vi "MC_8_27_12b_JW.vi"() -> ()   [LabVIEW 2011]
uses:
  <vilib>/Utility/file.llb/Read From Spreadsheet File (string).vi
  <vilib>/Utility/inputDevices.llb/keyboardAcquire.vi
  <vilib>/Utility/file.llb/Write To Spreadsheet File (DBL).vi
  <vilib>/Utility/file.llb/Write To Spreadsheet File (string).vi
  <vilib>/regexp/Match Regular Expression.xnode
panel:
  out "Vd Header Row 2":sgl
  in  "default (0 dbl)":ext format="%.2e"
  out "Vd Header Row":sgl
  out "Transport Array":string[][](array[string])
  in  "Treatment Concentration (mM):":dbl=nan
  in  "Surface Treatment:":string="NaN"
  in  "# Drops*:":dbl=inf
  in  "Solution Temp (C):":dbl=nan
  in  "Relative Humidity (%):":dbl=nan
  in  "Room Temp (F):":dbl=nan
  in  "Time (s):":dbl=nan
  in  "RPM:":dbl=nan
  in  "Wait Time (s):":dbl=nan
  in  "Sample #:":dbl=1.0
  in  "Fabricator:":string="NaN"
  in  "Ramp (s):":dbl=3.0
  out "X Axis Display Type":string
  out "Opj X Axis":string
  in  "Room Temp":dbl=294.0
  out "No Image 2":path=path "\\\\acad1\\physics/Jurchescu-group/JW-PD/Image Not Found.png"
  out "Save1 Array":string[][](array[string])
  out "Lin Vd":dbl
  out "Lin-Vg Array-Used":dbl[](array[numeric])
  out "Lin Id-Used":dbl[](array[numeric])
  out "Rec: Comments":string
  out "Folder Index":dbl caption="Length"
  out "Current \nRecord":string[](array[string])
  out "Transformer \nHeaders":string[](array[string])
  out "Current Device ID":string
  out "Column":string
  out "Row":string
  out "Rec: Concentration":dbl
  out "Rec: Solvent":string
  out "Rec: Method":string
  in  "?":T1(tab)
  in  "Transport File":path
  out "Transport Folder":path
  out "Rec: Material":string
  out "Accel (RPM/s):":dbl
  in  "Transfer File":path
  out "Transfer Folder":path
  in  "Image Folder":path
  out "Image File":path=path "D:/UserData/Desktop/Jeremy/WFU/Research/Programs/VI mods/Image Not Found.png"
  in  "Manual Comments":bool
  in  "Comments:":string
  out "Calc: On/Off":dbl caption="On/Off-Sat" format="%#.2e"
  out "Calc: Off I-Sat":dbl caption="Off I-Sat" format="%#.2e"
  in  "Manuel-Dielectric":bool
  in  "Manuel-Length":bool
  out "Calc: VT-Lin":dbl
  out "New: VT-Lin":dbl
  out "Rec: VT-Lin":dbl caption="VT-Lin" format="%#_3g"
  out "Calc: Trap Density-STS":dbl format="%#.2e"
  out "New: Trap Density-STS":dbl format="%#.2e"
  out "Rec: Trap Density-STS":dbl caption="N-Sat (STS)" format="%#.2e"
  out "Calc: Trap Density-VT":dbl format="%#.2e"
  out "New: Trap Density-VT":dbl format="%#.2e"
  out "Rec: Trap Density-VT":dbl caption="N-Sat (VT)" format="%#.2e"
  out "Calc: Mobility-Lin":dbl format="%#.2e"
  out "New: Mobility-Lin":dbl format="%#_4e"
  out "Rec: Mobility-Lin":dbl caption="Mobility-Lin" format="%#_3e"
  out "Calc: Mobility-Sat":dbl format="%#.2e"
  out "Rec: Length":dbl caption="Length" format="%#_3g"
  out "Rec: Width":dbl caption="Width" format="%#_4g"
  out "Rec: Dielectric (d)":dbl caption="Dielectric (d)" format="%#_3g"
  in  "Cancel Button":bool
  in  "Up Button":bool
  in  "Down Button":bool
  out "Data Name:":string
  in  "Save Changes?":bool
  in  "New: Dielectric":dbl
  in  "New: Length":dbl
  in  "New: Width":dbl
  out "New: Mobility-Sat":dbl format="%#.2e"
  in  "Blank Button":bool
  in  "Zoom":i16(slide)=-3 scale=-5.0..5.0
  out "Image Out 2":T2(plugin-control)
  out "Image Out":T2(plugin-control)
  in  "Magnification":u16(ring) items=["5x", "10x", "20x", "50x", "80x"]
  out "Total Width":dbl
  out "Distances":dbl[](array[numeric])
  in  "Undo Button":bool
  in  "Remove Button":bool
  out "Rec: Mobility-Sat":dbl caption="Mobility-Sat" format="%#.2e"
  in  "Export":bool
  out "Calc: VT-Sat":dbl format="%#.2g"
  out "New: VT-Sat":dbl format="%#.2g"
  in  "Manual-Width":bool caption="Manual"
  out "Calc: STS":dbl format="%#.2g"
  out "New: STS":dbl format="%#.2g"
  out "Rec: VT-Sat":dbl caption="VT-Sat" format="%#.2g"
  out "Rec: STS":dbl caption="STS-Sat" format="%#.2g"
  out "Rec: On/Off":dbl caption="On/Off-Sat" format="%#.2e"
  in  "Save Changes? 2":bool
  in  "Save Changes? 3":bool
  out "Rec: Temp":dbl caption="Sample Temp" format="%.1f"
  in  "New: Temp":dbl format="%.1f"
  out "Rec: Off I-Sat":dbl caption="Off I-Sat" format="%#.2e"
  in  "Independant Variable":string(combo)="Length (um):"
  in  "Transfer Plots":T3(tab)=enum."Saturation"
  in  "Lin-Trans Slider":dbl(slide) step=1.0 scale=-22.0..89.0 scale format="%#_1p"
  out "Sqrt-Lin":cluster{dbl[], dbl[]}[](graph)
  in  "Next Sqrt Lin":bool
  in  "Previous Sqrt Lin":bool
  in  "Sat-Trans Slider":dbl(slide) step=1.0 scale=-22.0..89.0 scale format="%#_1p"
  out "Sqrt-Sat":cluster{dbl[], dbl[]}[](graph)
  in  "Previous Sqrt Sat":bool
  in  "Next Sqrt Sat":bool
  out "Raw- Lin":cluster{dbl[], dbl[]}[](graph)
  out "Raw- Sat":cluster{dbl[], dbl[]}[](graph)
  in  "Log Plots":enum32{"Linear", "Saturation", "Transport"}(tab)=enum."Saturation"
  in  "Lin-Log Slider":dbl(slide) step=1.0 scale=-1.0..82.0 scale format="%#_1p"
  in  "Previous Log Lin":bool
  in  "Next Log Lin":bool
  out "Log-Lin":cluster{dbl[], dbl[]}[](graph)
  in  "Sat-Log Slider":dbl(slide) step=1.0 scale=-1.0..82.0 scale format="%#_1p"
  out "Log-Sat":cluster{dbl[], dbl[]}[](graph)
  in  "Previous Log Sat":bool
  in  "Next Log Sat":bool
  out "Transport":cluster{dbl[], dbl[]}[](graph)
  in  "Manual-Temp":bool caption="Manual"
  out "Date Created":string caption="Fabricated"
  out "Date Recorded":string="Date Recorded" caption="Measured"
  out "Image Name":string
  out "Index":string
  in  "Num Pts":dbl=5.0
  in  "NumPoints Log":dbl=5.0 caption="Num Pts"
  in  "Origin Project File":path=path "\\\\acad1\\physics/Jurchescu-group/JW-PD/Group Library/Origin Project Files/DeviceData_8_10_12a_JW.opj"
  in  "No Image File":path=path "\\\\acad1\\physics/Jurchescu-group/JW-PD/Mega Awesome/Image Not Found.png"
  out "String":string
  out "Index 2":dbl
  out "Sat Id-Log-Used":dbl[](array[numeric])
  out "Vg Array-Log-Used":dbl[](array[numeric])
  out "ROI Descriptor out":T4 {"Contours"."Type" items=["No Selection", "Point", "Line", "Rectangle", "Oval", "Polygon", "Freehand Region", "Annulus", "Unused2", "Unused3", "Broken Line", "Freehand Line", "Rotated Rectangle"]}
  out "ROI Descriptor":T4 {"Contours"."Type" items=["No Selection", "Point", "Line", "Rectangle", "Oval", "Polygon", "Freehand Region", "Annulus", "Unused2", "Unused3", "Broken Line", "Freehand Line", "Rotated Rectangle"]}
  out "Numeric 3":dbl
  out "Array 6":dbl[][](array[numeric])
  out "Cluster":T5
  out "Array 5":dbl[](array[numeric])
  out "Array 4":dbl[](array[numeric])
  out "Array 3":dbl[](array[numeric])
  out "Numeric 2":dbl
  out "Numeric":dbl
  out "Sat Id-Used":dbl[](array[numeric])
  out "Sat Vg Array-Used":dbl[](array[numeric])
  out "MobVi Index":dbl
  in  "Row Start":dbl=20.0
  # "Sample Properties"
  # "*     Inf = Full coverage\n   NaN = Unknown or Not Applicable"
  # "Data Locations"
  # "Transport Location"
  # "Transfer Location"
  # "Image Location"
  # "Recorded"
  # "Calculated"
  # "Re-Calculated"
  # "Manual"
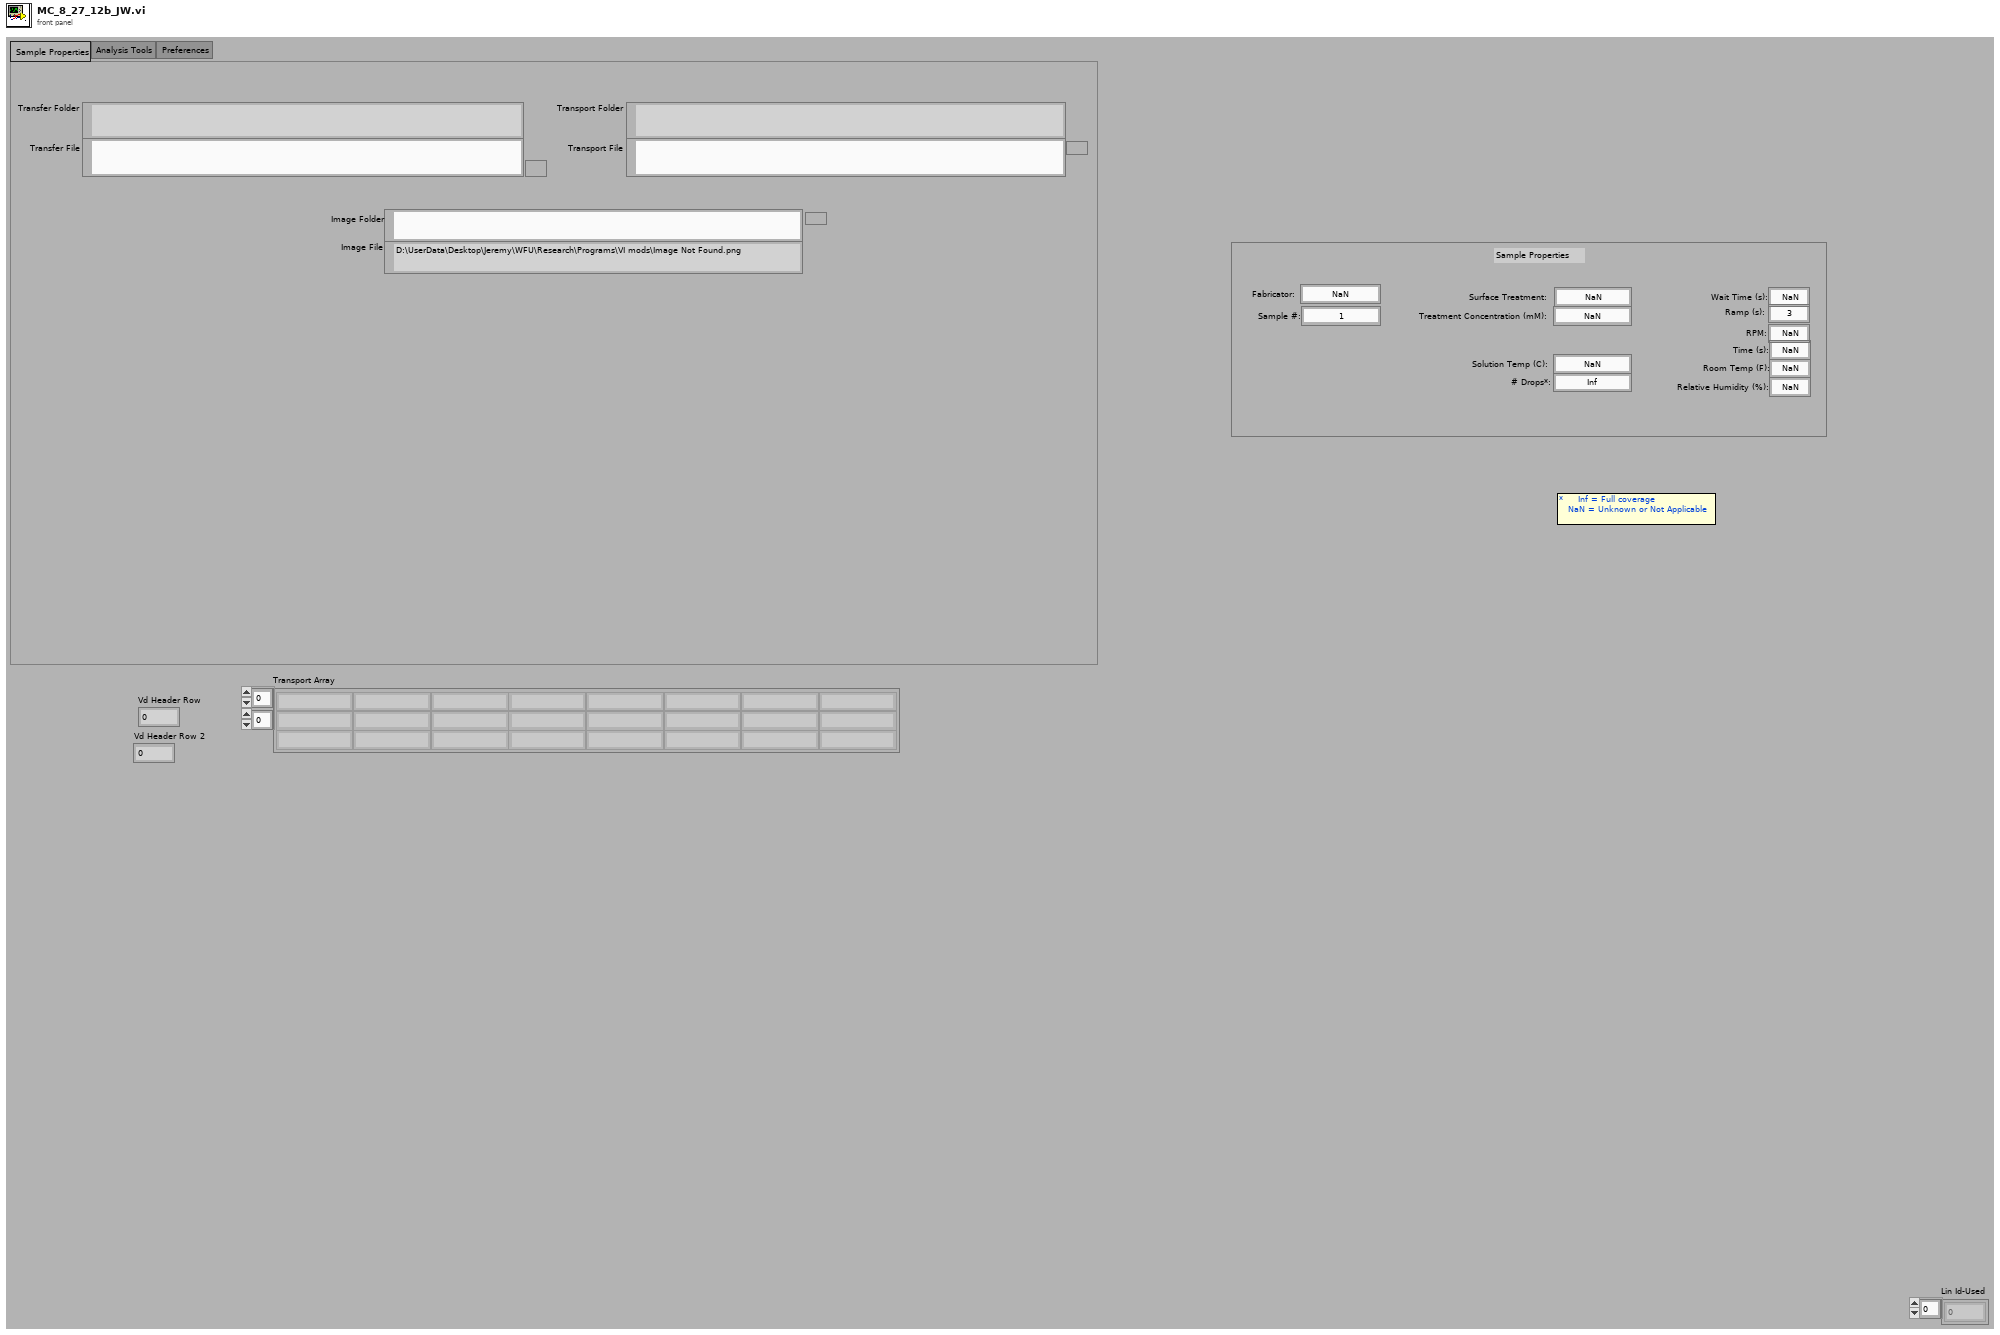
[diagram p1: front panel]
types:
  T1 = enum32{"Sample Properties", "Analysis Tools", "Preferences", "Current Database"}
  T2 = typedef "IMAQ Image.ctl" = refnum<image>
  T3 = enum32{"Linear", "Saturation", "Raw-Linear", "Raw-Saturation"}
  T4 = typedef "ROI Descriptor" = cluster{"Global Rectangle":i32[], "Contours":cluster{"ID":enum32{"External", "Internal"}, "Type":u32, "Coordinates":i32[]}[]}
  T5 = cluster{"Numeric":dbl, "Numeric 2":dbl, "Numeric 3":dbl, "Numeric 4":dbl}
  T6 = cluster{"Mobility-Sat":dbl, "Moblitity-Lin":dbl, "On/Off":dbl, "Off Current":dbl, "Vt-Sat":dbl, "STS":dbl, "Trap Density-VT":dbl, "Trap Density-STS":dbl}
  T7 = cluster{"Date Recorded":string, "Index":string, "Length":dbl, "Width":dbl, "Sample Temp":dbl}
  T8 = cluster{"Date Created":string, "Material":string, "Solvent":string, "Concentration":dbl, "Method":string, "Dielectric (nm)":dbl, "Treatment":string, "Comments":string}
  T9 = cluster{"Raw Sat":cluster{dbl[], dbl[]}[], "Sqrt Sat":cluster{dbl[], dbl[]}[], "Log Sat":cluster{dbl[], dbl[]}[], "Raw Lin":cluster{dbl[], dbl[]}[], "Sqrt Lin":cluster{dbl[], dbl[]}[], "Log Lin":cluster{dbl[], dbl[]}[]}
  T10 = cluster{"Mobility-Sat":dbl, "Vt-Sat":dbl, "Mobility-Lin":dbl, "Vt-Lin":dbl, "Off I-Sat":dbl, "On/Off I-Sat":dbl}
  T11 = cluster{"[0]":cluster{dbl[], dbl[]}, "[1]":cluster{dbl[], dbl[]}, "[2]":cluster{dbl[], dbl[]}, "[3]":cluster{dbl[], dbl[]}, "[4]":cluster{dbl[], dbl[]}, "[5]":cluster{dbl[], dbl[]}, "[6]":cluster{dbl[], dbl[]}, "[7]":cluster{dbl[], dbl[]}, "[8]":cluster{dbl[], dbl[]}}
  T12 = cluster{"Global Rectangle":i32[], "Contours":cluster{"Contour Type":u32, "ROI Type":u32, "Points":i32[]}[]}
  T13 = typedef "LVBoundsTypeDef.ctl" = cluster{"Width":u32, "Height":u32}
  T14 = enum16{"0", "1", "2", "3", "4", "5", "6", "7", "8", "9", "A", "B", "C", "D", "E", "F", "G", "H", "I", "J", "K", "L", "M", "N", "O", "P", "Q", "R", "S", "T", "U", "V", "W", "X", "Y", "Z", "F1", "F2", "F3", "F4", "F5", "F6", "F7", "F8", "F9", "F10", "F11", "F12", "F13", "F14", "F15", "ADD", "BACK", "BACKSLASH", "CAPITAL", "COMMA", "DECIMAL", "DELETE", "DIVIDE", "DOWN", "END", "EQUALS", "ESCAPE", "GRAVE (`)", "HOME", "INSERT", "LBRACKET", "LCONTROL", "LEFT", "L ALT", "LSHIFT", "LWIN", "MINUS", "MULTIPLY", "NEXT", "NUMLOCK", "NUMPAD_0", "NUMPAD_1", "NUMPAD_2", "NUMPAD_3", "NUMPAD_4", "NUMPAD_5", "NUMPAD_6", "NUMPAD_7", "NUMPAD_8", "NUMPAD_9", "PAUSE", "PERIOD", "PRIOR (PG UP)", "RBRACKET", "RCONTROL", "RETURN", "RIGHT", "R ALT", "RSHIFT", "RWIN", "SCROLL", "SEMICOLON", "SLASH", "SPACE", "SUBTRACT", "TAB", "UP", "ENTER (num pad)", "' (quote)"}[]
  T15 = enum16{"0", "1", "2", "3", "4", "5", "6", "7", "8", "9", "A", "B", "C", "D", "E", "F", "G", "H", "I", "J", "K", "L", "M", "N", "O", "P", "Q", "R", "S", "T", "U", "V", "W", "X", "Y", "Z", "F1", "F2", "F3", "F4", "F5", "F6", "F7", "F8", "F9", "F10", "F11", "F12", "F13", "F14", "F15", "ADD", "BACK", "BACKSLASH", "CAPITAL", "COMMA", "DECIMAL", "DELETE", "DIVIDE", "DOWN", "END", "EQUALS", "ESCAPE", "GRAVE (`)", "HOME", "INSERT", "LBRACKET", "LCONTROL", "LEFT", "L ALT", "LSHIFT", "LWIN", "MINUS", "MULTIPLY", "NEXT", "NUMLOCK", "NUMPAD_0", "NUMPAD_1", "NUMPAD_2", "NUMPAD_3", "NUMPAD_4", "NUMPAD_5", "NUMPAD_6", "NUMPAD_7", "NUMPAD_8", "NUMPAD_9", "PAUSE", "PERIOD", "PRIOR (PG UP)", "RBRACKET", "RCONTROL", "RETURN", "RIGHT", "R ALT", "RSHIFT", "RWIN", "SCROLL", "SEMICOLON", "SLASH", "SPACE", "SUBTRACT", "TAB", "UP", "ENTER (num pad)", "' (quote)"}
  T16 = cluster{"Contour Type":u32, "ROI Type":u32, "Points":i32[]}[]
  T17 = cluster{i32[], cluster{"Contour Type":u32, "ROI Type":u32, "Points":i32[]}[]}
  T18 = cluster{"Independant  Variable Indicator":string, "Parameter String Indicator":string}
  T19 = cluster{string, sgl, bool, bool, bool, bool, bool, bool, i32}
  T20 = cluster{i32, cluster{string, sgl, bool, bool, bool, bool, bool, bool, i32}, i32, i32}
  T21 = cluster{"Contour Type":u32, "ROI Type":u32, "Points":i32[]}
  T22 = cluster{"Points[0]":i32, "Points[1]":i32, "Points[2]":i32, "Points[3]":i32, "Points[4]":i32, "Points[5]":i32, "Points[6]":i32, "Points[7]":i32, "Points[8]":i32}
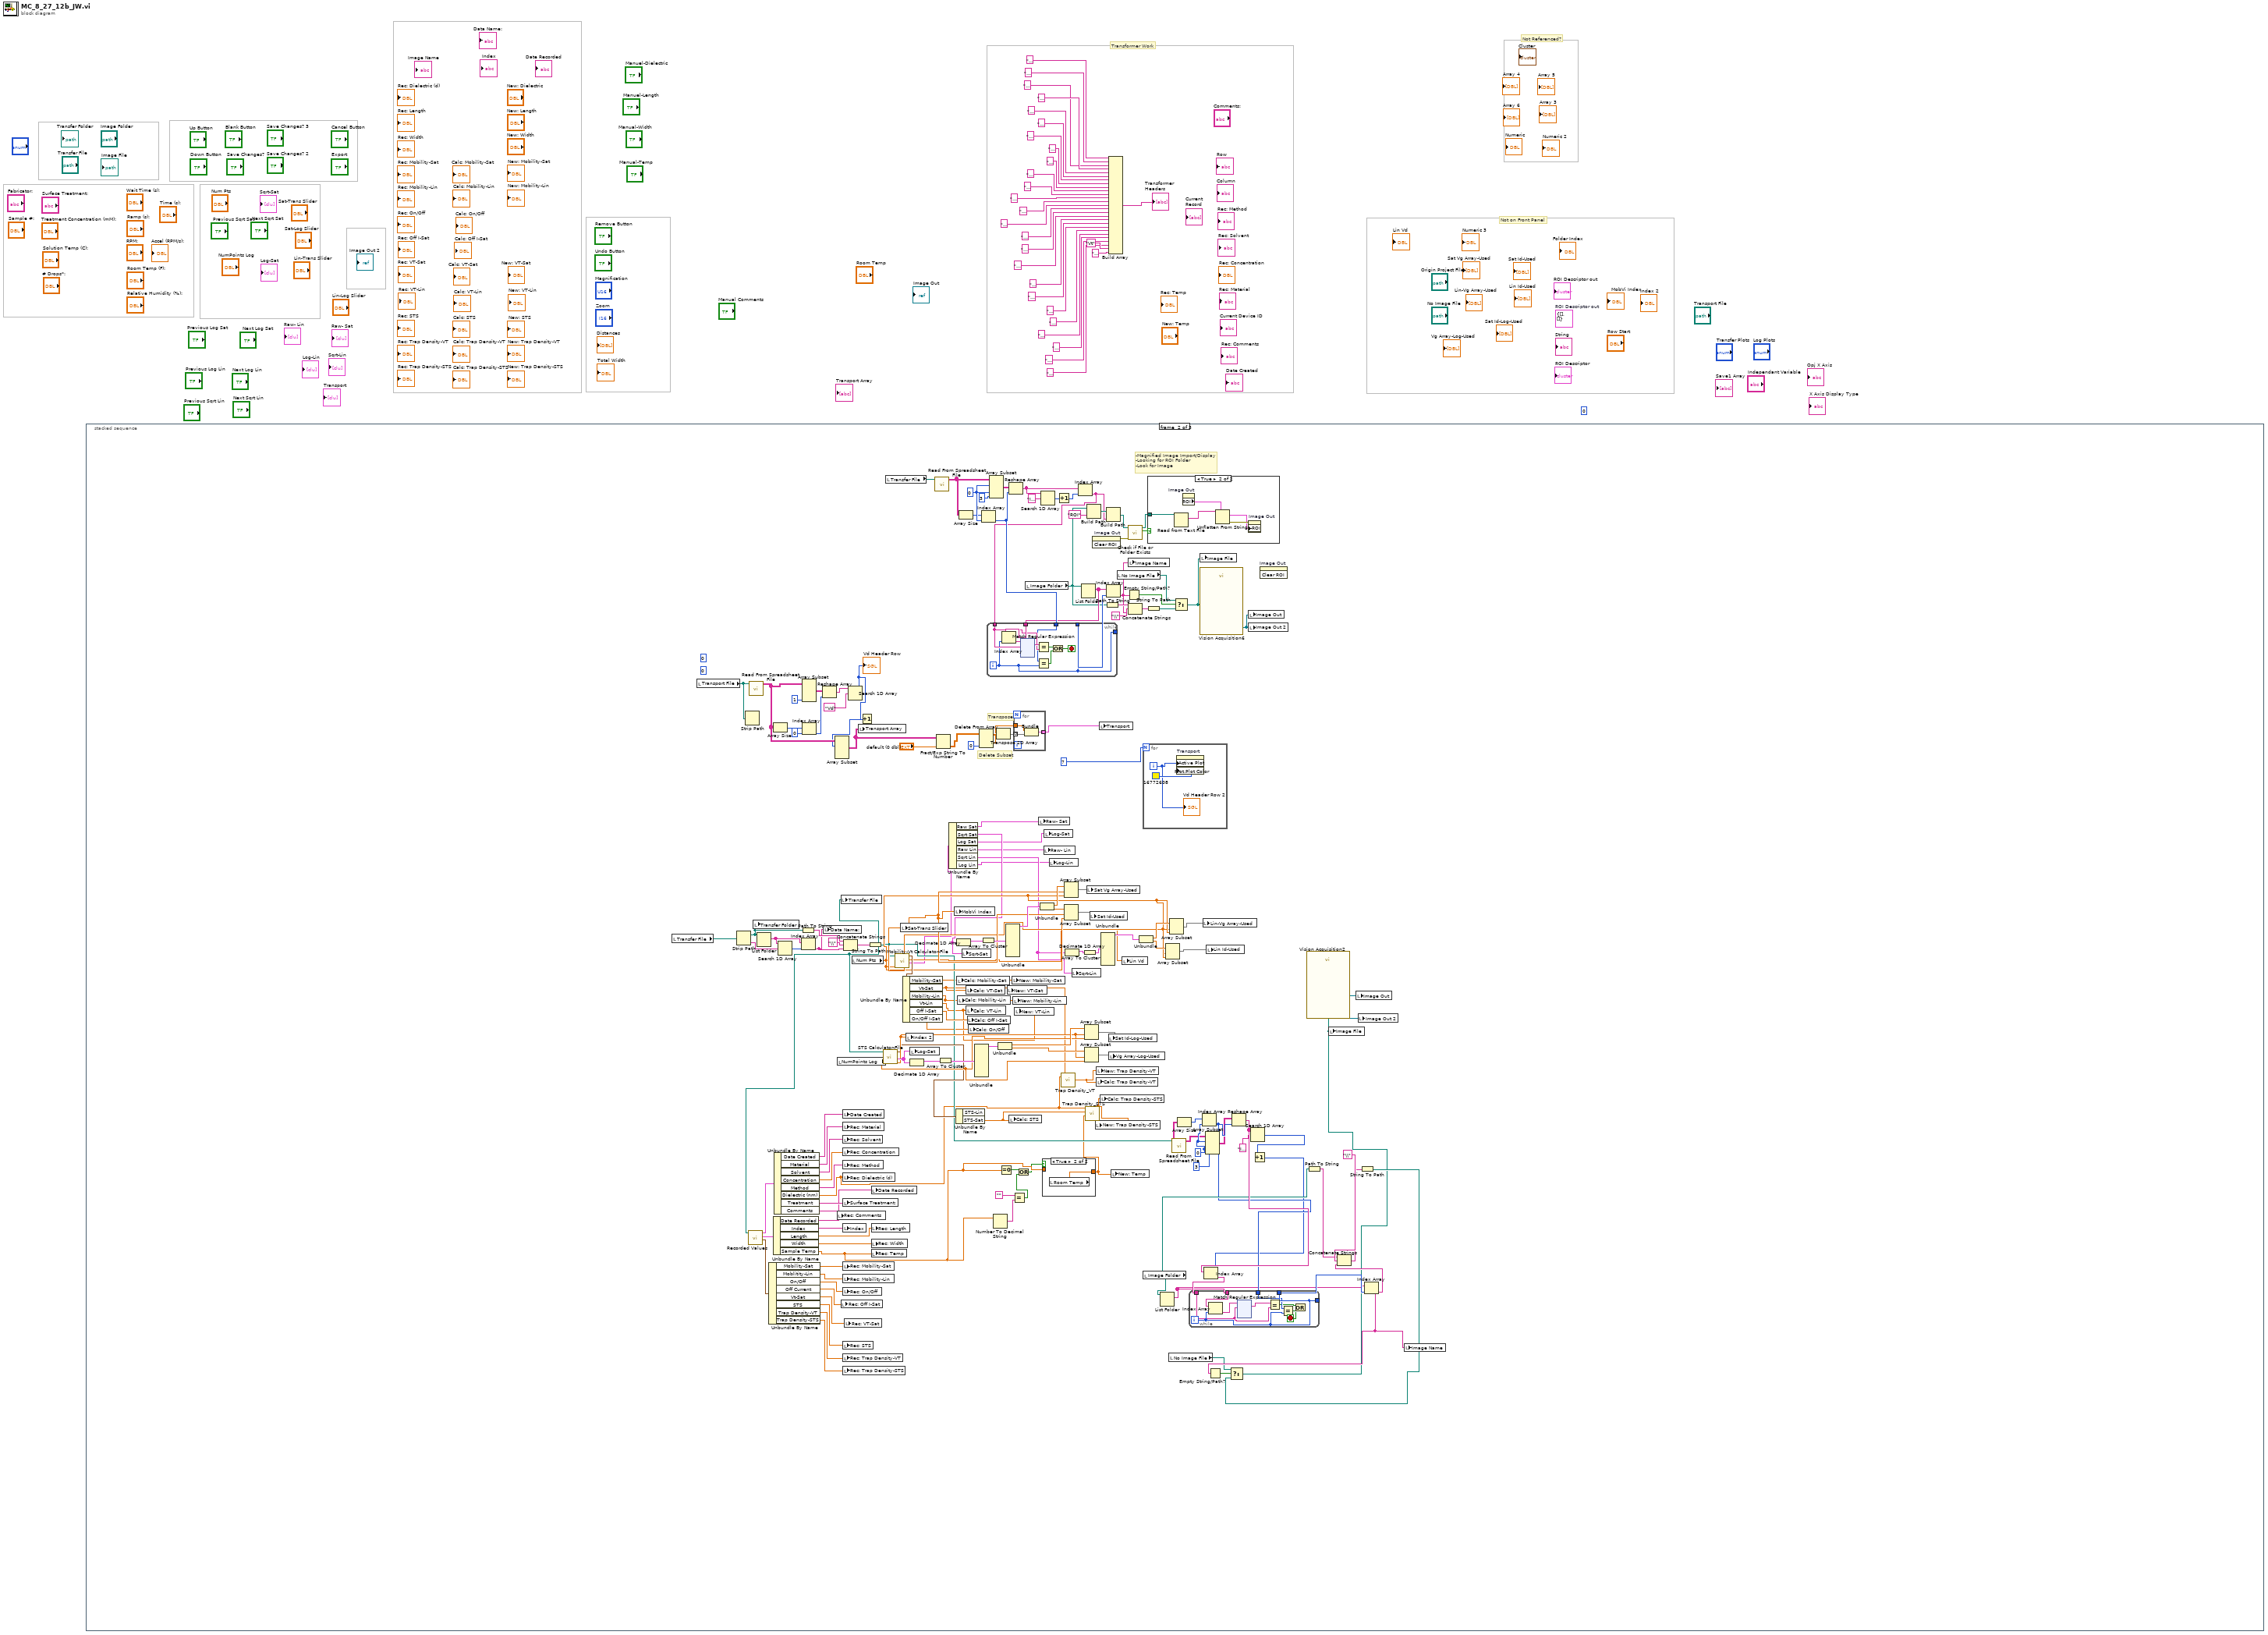
[diagram p0: block diagram]
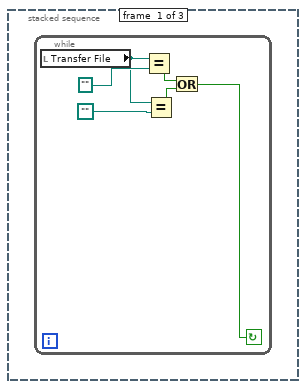
[diagram p2: hidden frame]
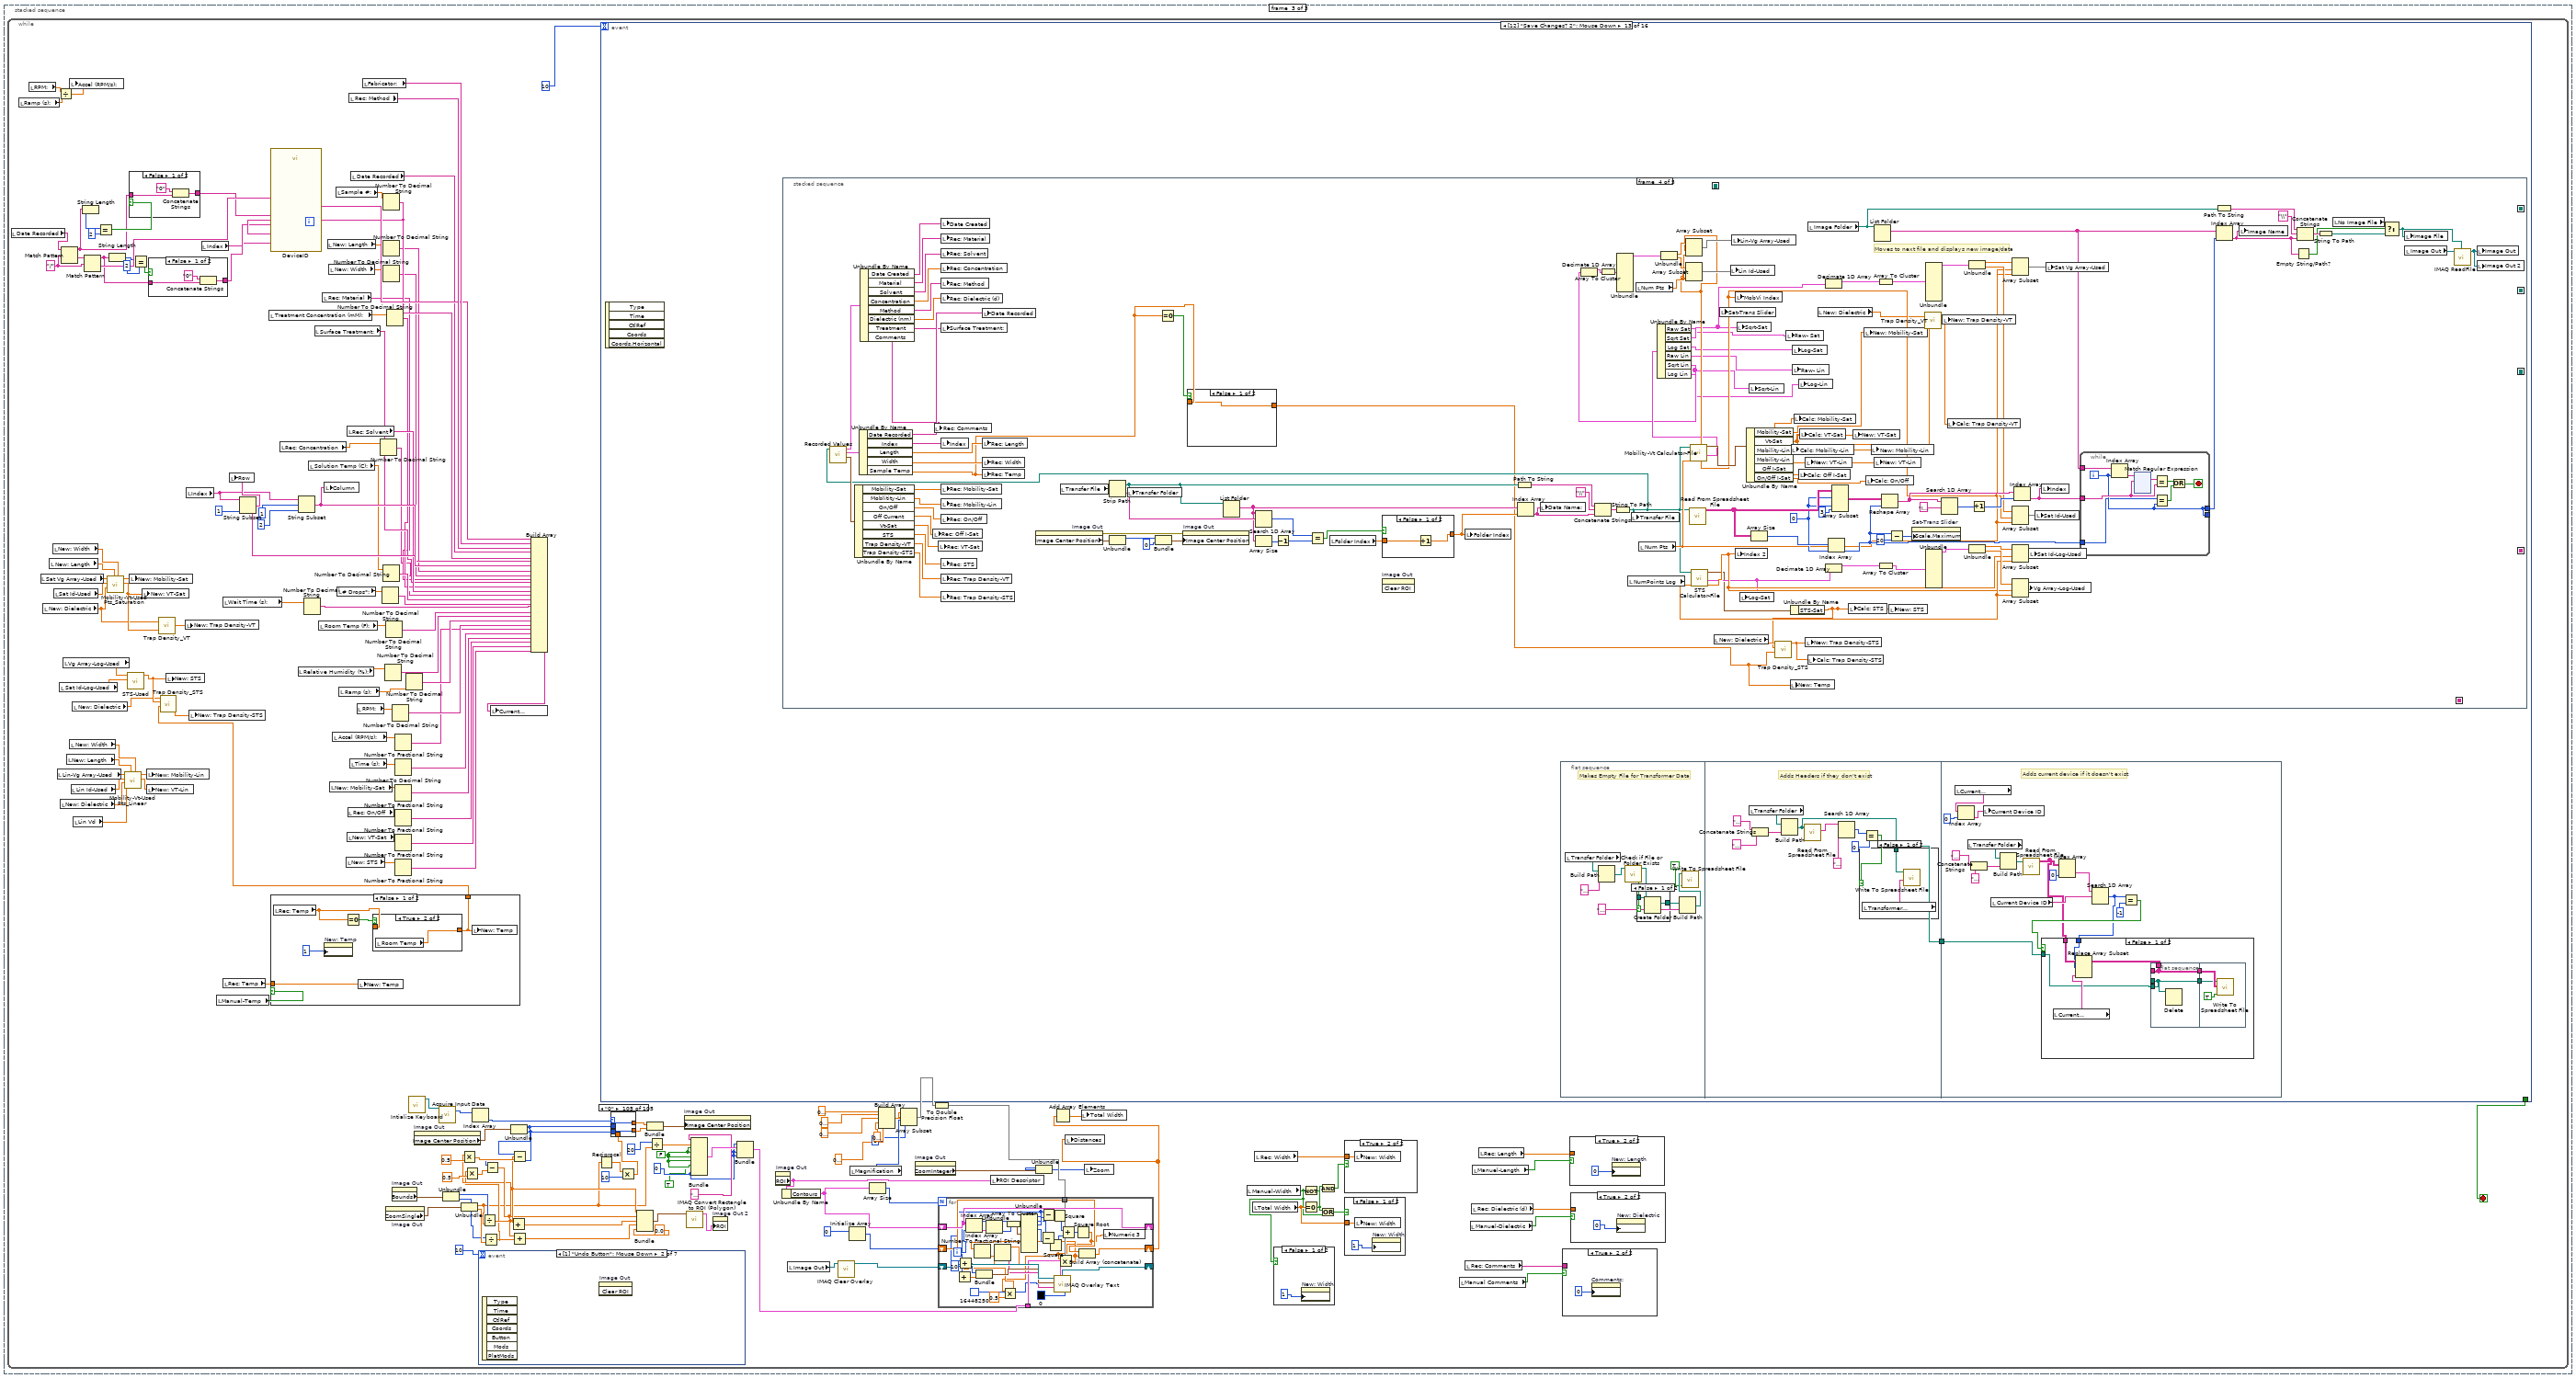
[diagram p5: hidden frame]
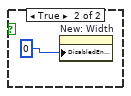
[diagram p6: hidden frame]
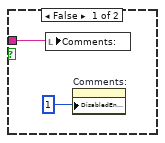
[diagram p7: hidden frame]
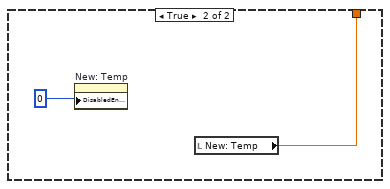
[diagram p9: hidden frame]
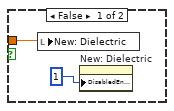
[diagram p10: hidden frame]
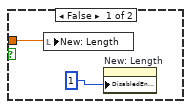
[diagram p11: hidden frame]
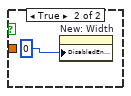
[diagram p15: hidden frame]
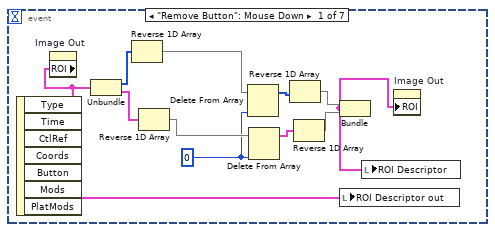
[diagram p16: hidden frame]
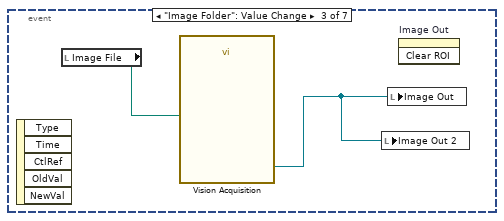
[diagram p17: hidden frame]
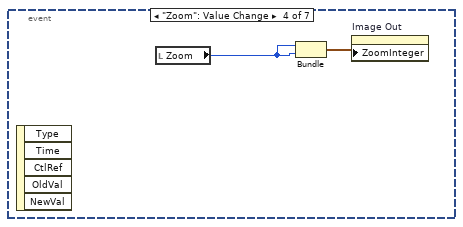
[diagram p18: hidden frame]
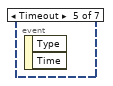
[diagram p19: hidden frame]
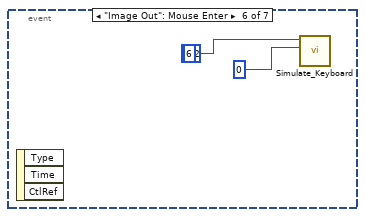
[diagram p20: hidden frame]
diagram:
  (unwired) 0
  (unwired) T4 {"Global Rectangle"=[], "Contours"=[]}  # ROI Descriptor out
  # "Not Referenced?"
  # "Transformer Work"
  # "Not on Front Panel"
  n1 = stacked-sequence {
    frame #0 {
      n2 = while {
        stop <- w29 continue-if-true
        n3 = local read "Transfer File"() -> (w31:path)
        n4 = Equal?(x=w31, y=path "") -> (x = y?=w33:bool)
        n5 = Equal?(x=w31, y=path "") -> (x = y?=w32:bool)
        n6 = Or(x=w33, y=w32) -> (x .or. y?=w29:bool)
      }
    }
    frame #1 {
      (unwired) 0
      (unwired) 0
      w158 = 0
      w182 = 0
      # "Transpose"
      # "Delete Subset"
      # "-Magnified Image Import/Display\n-Looking for ROI Folder\n-Look for Image"
      n7 = local read "Transfer File"() -> (w162:path)
      n8 = local read "Transport File"() -> (w54:path)
      n9 = Strip Path(path=w162) -> (stripped path=w163:path, name=w149:string)
      n10 = Strip Path(path=w54) -> ()  [unwired: 2 out]
      n11 = call-poly <vilib>:"Read From Spreadsheet File.vi"("file path (dialog if empty)"=w54) -> ("all rows"=w47:string[][])  [unwired: 6 in, 4 out]
      n12 = local write "Transfer Folder"(w163) -> ()
      n13 = List Folder(path=w163) -> (filenames=w153:string[])  [unwired: 3 in, 3 out]
      n14 = Array Size(array=w47) -> (size(s)=w53:i32[])
      n15 = Search 1D Array(1D array=w153, element=w149) -> (index of element=w152:i32)  [unwired: 1 in]
      n16 = Path To String(path=w163) -> (string=w148:string)
      n17 = Index Array(array=w153, index=w152) -> (element=w118:string)
      n18 = Array Subset(array=w47, length (col)=1) -> (w49:string[][])  [unwired: 3 in]
      n19 = Index Array(array=w53, index=0) -> (element=w42:i32)
      n20 = Reshape Array(w49, w42) -> (w48:string[])
      n21 = local write "Data Name:"(w118) -> ()
      n22 = local read "NumPoints Log"() -> (w94:dbl)
      n23 = Concatenate Strings(w148, "\\", w118) -> (w150:string)
      n24 = Search 1D Array(1D array=w48, element="Vd") -> (index of element=w46:i32)  [unwired: 1 in]
      "Vd Header Row" <- w46
      n25 = local read "Num Pts"() -> (w85:dbl)
      n26 = Increment(x=w46) -> (x+1=w45:i32)
      n27 = Array Subset(array=w47, index (row)=w45) -> (w43:string[][])  [unwired: 3 in]
      n28 = local write "Transport Array"(w43) -> ()
      n29 = String To Path(string=w150) -> (path=w79:path)
      n30 = call "Recorded Values.vi"("Path"=w79) -> ("Recorded Char"=w116:T6, "Recorded Prop"=w115:T7, "Fabrication Prop"=w117:T8)  [unwired: 8 in]
      n31 = Unbundle By Name(w116) -> ("Mobility-Sat"=w104:dbl, "Moblitity-Lin"=w103:dbl, "On/Off"=w102:dbl, "Off Current"=w101:dbl, "Vt-Sat"=w65:dbl, "STS"=w100:dbl, "Trap Density-VT"=w99:dbl, "Trap Density-STS"=w98:dbl)
      n32 = Unbundle By Name(w115) -> ("Date Recorded"=w108:string, "Index"=w107:string, "Length"=w106:dbl, "Width"=w105:dbl, "Sample Temp"=w71:dbl)
      n33 = Unbundle By Name(w117) -> ("Date Created"=w97:string, "Material"=w114:string, "Solvent"=w113:string, "Concentration"=w112:dbl, "Method"=w111:string, "Dielectric (nm)"=w75:dbl, "Treatment"=w110:string, "Comments"=w109:string)
      n34 = local write "Rec: Comments"(w109) -> ()
      n35 = local write "Transfer File"(w79) -> ()
      n36 = local write "Rec: Off I-Sat"(w101) -> ()
      n37 = local write "Date Created"(w97) -> ()
      n38 = local write "Rec: Material"(w114) -> ()
      n39 = local write "Rec: Solvent"(w113) -> ()
      n40 = local write "Rec: Concentration"(w112) -> ()
      n41 = local write "Rec: Method"(w111) -> ()
      n42 = local write "Rec: Dielectric (d)"(w75) -> ()
      n43 = local write "Surface Treatment:"(w110) -> ()
      n44 = local write "Index"(w107) -> ()
      n45 = local write "Rec: Mobility-Sat"(w104) -> ()
      n46 = local write "Rec: Mobility-Lin"(w103) -> ()
      n47 = local write "Rec: On/Off"(w102) -> ()
      n48 = local write "Rec: STS"(w100) -> ()
      n49 = local write "Rec: Trap Density-VT"(w99) -> ()
      n50 = local write "Rec: Trap Density-STS"(w98) -> ()
      n51 = local write "Rec: VT-Sat"(w65) -> ()
      n52 = local write "Date Recorded"(w108) -> ()
      n53 = local write "Rec: Length"(w106) -> ()
      n54 = local write "Rec: Width"(w105) -> ()
      n55 = local write "Rec: Temp"(w71) -> ()
      n56 = call "STS Calculator-File.vi"("NumPts"=w94, "Path"=w79) -> ("STS Index-Sat"=w92:dbl, "XY Graph-Sat"=w93:cluster{dbl[], dbl[]}[], "Ouput"=w91:cluster{"STS-Sat":dbl, "STS-Lin":dbl})  [unwired: 5 in, 2 out]
      n57 = local read "Transfer File"() -> (w177:path)
      n58 = call "Mobility-Vt Calculator-File.vi"("NumPts"=w85, "Path"=w79) -> ("Graph Cluster"=w55:T9, "Lin Vd"=w81:dbl, "Output"=w96:T10, "Index-Sat"=w95:dbl, "Index-Lin"=w84:dbl)  [unwired: 5 in]
      n59 = local write "Sat-Trans Slider"(w95) -> ()
      n60 = Unbundle By Name(w96) -> ("Mobility-Sat"=w74:dbl, "Vt-Sat"=w73:dbl, "Mobility-Lin"=w64:dbl, "Vt-Lin"=w62:dbl, "Off I-Sat"=w80:dbl, "On/Off I-Sat"=w63:dbl)
      n61 = local write "Index 2"(w92) -> ()
      n62 = Decimate 1D Array(w93) -> (w140:cluster{dbl[], dbl[]}[])  [unwired: 1 out]
      n63 = local write "Log-Sat"(w93) -> ()
      n64 = call-poly <vilib>:"Read From Spreadsheet File.vi"("file path (dialog if empty)"=w177) -> ("all rows"=w180:string[][])  [unwired: 6 in, 4 out]
      n65 = Fract/Exp String To Number(string=w43, default (0 dbl)="default (0 dbl)") -> (number=w37:ext[][])  [unwired: 2 in, 1 out]
      n66 = Array To Cluster(array=w140) -> (cluster=w142:T11)
      n67 = Unbundle By Name(w55) -> ("Raw Sat"=w59:cluster{dbl[], dbl[]}[], "Sqrt Sat"=w61:cluster{dbl[], dbl[]}[], "Log Sat"=w56:cluster{dbl[], dbl[]}[], "Raw Lin"=w58:cluster{dbl[], dbl[]}[], "Sqrt Lin"=w60:cluster{dbl[], dbl[]}[], "Log Lin"=w57:cluster{dbl[], dbl[]}[])
      n68 = local write "MobVi Index"(w95) -> ()
      n69 = Unbundle By Name(w91) -> ("STS-Sat"=w78:dbl)  [unwired: 1 out]
      n70 = Decimate 1D Array(w61) -> (w176:cluster{dbl[], dbl[]}[])  [unwired: 1 out]
      n71 = local write "Calc: Mobility-Sat"(w74) -> ()
      n72 = local write "Calc: Mobility-Lin"(w64) -> ()
      n73 = Array Size(array=w180) -> (size(s)=w181:i32[])
      n74 = local write "Sqrt-Sat"(w61) -> ()
      n75 = local write "Calc: VT-Sat"(w73) -> ()
      n76 = local write "Calc: VT-Lin"(w62) -> ()
      n77 = local write "Calc: Off I-Sat"(w80) -> ()
      n78 = local write "Calc: On/Off"(w63) -> ()
      n79 = Unbundle(w142) -> ("[0]"=w141:cluster{dbl[], dbl[]})  [unwired: 8 out]
      n80 = Delete From Array(array=w37, index (col)=0 ("Deaktivierter Index (Spalte)")) -> (deleted portion=w39:ext[], array with subset deleted=w40:ext[][])  [unwired: 2 in]
      n81 = Array To Cluster(array=w176) -> (cluster=w174:T11)
      n82 = Index Array(array=w181, index=w182) -> (element=w188:i32)
      n83 = Array Subset(array=w180, index (row)=w182, index (col)=w182, length (col)=3) -> (w179:string[][])  [unwired: 1 in]
      n84 = Number To Decimal String(number=w71) -> (decimal integer string=w69:string)  [unwired: 1 in]
      n85 = Transpose 2D Array(2D array=w40) -> (transposed array=w41:ext[][])
      n86 = Unbundle(w141) -> (w138:dbl[], w137:dbl[])
      n87 = Equal To 0?(x=w71) -> (x = 0?=w70:bool)
      n88 = Unbundle(w174) -> ("[0]"=w175:cluster{dbl[], dbl[]})  [unwired: 8 out]
      n89 = local write "New: VT-Sat"(w73) -> ()
      n90 = Reshape Array(w179, w188) -> (w193:string[])
      n91 = local write "Calc: STS"(w78) -> ()
      n92 = local write "New: Mobility-Sat"(w74) -> ()
      n93 = Equal?(x="", y=w69) -> (x = y?=w67:bool)
      n94 = local write "New: Mobility-Lin"(w64) -> ()
      n95 = for {
        tunnel: w39 -> [w197]
        tunnel: w41 -> [w198] mode=indexing
        tunnel: [w196] -> w36 mode=indexing
        n96 = Bundle(w197, w198) -> (w196:cluster{ext[], ext[]})  [unwired: 1 in]
      }
      n97 = local write "New: VT-Lin"(w62) -> ()
      n98 = Or(x=w70, y=w67) -> (x .or. y?=w66:bool)
      n99 = local read "Image Folder"() -> (w119:path)
      n100 = local write "Raw- Sat"(w59) -> ()
      n101 = Unbundle(w175) -> (w139:dbl[], w143:dbl[])
      n102 = Search 1D Array(1D array=w193, element="Index:") -> (index of element=w185:i32)  [unwired: 1 in]
      n103 = case shown="True" w66 {
        tunnel: [w199 w200] -> w77
        tunnel: w71 -> [w199 _]
        frame False {
        }
        frame True {
          n104 = local read "Room Temp"() -> (w200:dbl)
        }
      }
      n105 = local write "Raw- Lin"(w58) -> ()
      n106 = local write "Log-Sat"(w56) -> ()
      n107 = local write "Log-Lin"(w57) -> ()
      n108 = Increment(x=w185) -> (x+1=w184:i32)
      n109 = call "Trap Density_VT.vi"("VT"=w73, "Dielectric"=w75) -> ("Trap Density-VT"=w72:dbl)
      n110 = Array Subset(array=w139, index=w95, length=w85) -> (w146:dbl[])
      n111 = Array Subset(array=w143, index=w95, length=w85) -> (w147:dbl[])
      n112 = Decimate 1D Array(w60) -> (w90:cluster{dbl[], dbl[]}[])  [unwired: 1 out]
      n113 = local write "Sqrt-Lin"(w60) -> ()
      n114 = Index Array(array=w193, index=w184) -> (element=w120:string)
      n115 = List Folder(path=w119) -> (filenames=w186:string[])  [unwired: 3 in, 3 out]
      n116 = while {
        tunnel: w186 -> [w333]
        tunnel: w120 -> [w331]
        tunnel: [w330] -> _
        tunnel: [w330] -> w187
        tunnel: w188 -> [w329]
        i -> [w330]
        stop <- w326 stop-if-true
        n117 = Index Array(array=w333, index=w330) -> (element=w334:string)
        n118 = xnode "Match Regular Expression"("input string"=w334, "regular expression"=w331) -> ("whole match"=w332:string)  [unwired: 4 in, 4 out]
        n119 = Equal?(x=w332, y=w331) -> (x = y?=w328:bool)
        n120 = Equal?(x=w329, y=w330) -> (x = y?=w327:bool)
        n121 = Or(x=w328, y=w327) -> (x .or. y?=w326:bool)
      }
      n122 = Array To Cluster(array=w90) -> (cluster=w89:T11)
      n123 = Array Subset(array=w138, index=w92, length=w94) -> (w145:dbl[])
      n124 = Array Subset(array=w137, index=w92, length=w94) -> (w144:dbl[])
      n125 = call "Trap Density_STS.vi"("Temp (T) [K]"=w77, "S.T.S. (S)"=w78, "Dielectric"=w75) -> ("Trap Density (N)"=w76:dbl)  [unwired: 8 in]
      n126 = Build Path(base path=w119, name or relative path="ROI") -> (appended path=w122:path)
      n127 = local write "Sat Vg Array-Used"(w146) -> ()
      n128 = local write "Sat Id-Used"(w147) -> ()
      n129 = invoke on="Image Out" class="ImageControl" method="Clear ROI"() -> (error out=w126:errorcluster)  [unwired: 3 in, 2 out]
      n130 = local write "New: Trap Density-STS"(w76) -> ()
      n131 = local write "Calc: Trap Density-VT"(w72) -> ()
      n132 = local write "New: Trap Density-VT"(w72) -> ()
      n133 = local write "Transport"(w36) -> ()
      n134 = local write "Calc: Trap Density-STS"(w76) -> ()
      n135 = Unbundle(w89) -> ("[0]"=w88:cluster{dbl[], dbl[]})  [unwired: 8 out]
      n136 = Path To String(path=w119) -> (string=w190:string)
      n137 = Build Path(base path=w122, name or relative path=w120) -> (appended path=w121:path)
      n138 = Index Array(array=w186, index=w187) -> (element=w136:string)
      n139 = local write "Sat Id-Log-Used"(w145) -> ()
      n140 = local write "Vg Array-Log-Used"(w144) -> ()
      n141 = local write "New: Temp"(w77) -> ()
      n142 = local read "No Image File"() -> (w127:path)
      n143 = local write "Lin Vd"(w81) -> ()
      n144 = Empty String/Path?(string/path=w136) -> (empty?=w135:bool)
      n145 = call <vilib>:"Check if File or Folder Exists.vi"("error in (no error)"=w126, "path"=w121) -> ("file or folder exists?"=w124:bool, "dup path"=w125:path)  [unwired: 7 in, 1 out]
      n146 = local write "Image Name"(w136) -> ()
      n147 = Concatenate Strings(w190, "\\", w136) -> (w191:string)
      n148 = Unbundle(w88) -> (w87:dbl[], w86:dbl[])
      n149 = for {
        N: 7 -> [_]
        i -> [w194]
        n150 = property on="Transport" class="XYGraph (strict)"("Active Plot"=w194, "Plot.Plot Color"=u32 16772608) -> ()  [unwired: 2 in, 2 out]
        "Vd Header Row 2" <- w194
      }
      n151 = local read "Image Folder"() -> (w169:path)
      n152 = String To Path(string=w191) -> (path=w134:path)
      n153 = case shown="True" w124 {
        tunnel: w125 -> [_ w201]
        frame False {
        }
        frame True {
          n154 = Read from Text File(file (use dialog)=w201) -> (text=w205:string)  [unwired: 3 in, 3 out]
          n155 = property on="Image Out" class="ImageControl"() -> ("ROI"=w202:T12)  [unwired: 2 in, 2 out]
          n156 = Unflatten From String(type=w202, binary string=w205) -> (value=w203:T12, error out=w204:errorcluster)  [unwired: 3 in, 1 out]
          n157 = property on="Image Out" class="ImageControl"(error in=w204, "ROI"=w203) -> ()  [unwired: 1 in, 2 out]
        }
      }
      n158 = List Folder(path=w169) -> (filenames=w165:string[])  [unwired: 3 in, 3 out]
      n159 = Array Subset(array=w86, index=w84, length=w85) -> (w82:dbl[])
      n160 = local read "No Image File"() -> (w128:path)
      n161 = Array Subset(array=w87, index=w84, length=w85) -> (w83:dbl[])
      n162 = call-poly <vilib>:"Read From Spreadsheet File.vi"("file path (dialog if empty)"=w79) -> ("all rows"=w156:string[][])  [unwired: 6 in, 4 out]
      n163 = Select(t=w127, s=w135, f=w134) -> (s? t:f=w133:path)
      n164 = Array Size(array=w156) -> (size(s)=w157:i32[])
      n165 = local write "Image File"(w133) -> ()
      n166 = call "Vision Acquisition6"("Image Path"=w133) -> ("Image Out"=w189:T2)  [unwired: 25 in, 1 out]
      n167 = Index Array(array=w157, index=w158) -> (element=w168:i32)
      n168 = local write "Lin-Vg Array-Used"(w83) -> ()
      n169 = Array Subset(array=w156, index (row)=w158, index (col)=w158, length (col)=3) -> (w155:string[][])  [unwired: 1 in]
      n170 = local write "Lin Id-Used"(w82) -> ()
      n171 = Reshape Array(w155, w168) -> (w173:string[])
      n172 = local write "Image Out"(w189) -> ()
      n173 = local write "Image Out 2"(w189) -> ()
      n174 = Search 1D Array(1D array=w173, element="Index:") -> (index of element=w161:i32)  [unwired: 1 in]
      n175 = Increment(x=w161) -> (x+1=w160:i32)
      n176 = Index Array(array=w173, index=w160) -> (element=w166:string)
      n177 = while {
        tunnel: w165 -> [w213]
        tunnel: w166 -> [w211]
        tunnel: [w210] -> _
        tunnel: [w210] -> w167
        tunnel: w168 -> [w209]
        i -> [w210]
        stop <- w206 stop-if-true
        n178 = Index Array(array=w213, index=w210) -> (element=w214:string)
        n179 = xnode "Match Regular Expression"("input string"=w214, "regular expression"=w211) -> ("whole match"=w212:string)  [unwired: 4 in, 4 out]
        n180 = Equal?(x=w212, y=w211) -> (x = y?=w208:bool)
        n181 = Equal?(x=w209, y=w210) -> (x = y?=w207:bool)
        n182 = Or(x=w208, y=w207) -> (x .or. y?=w206:bool)
      }
      n183 = invoke on="Image Out" class="ImageControl" method="Clear ROI"() -> ()  [unwired: 3 in, 3 out]
      n184 = Path To String(path=w169) -> (string=w170:string)
      n185 = Index Array(array=w165, index=w167) -> (element=w131:string)
      n186 = Empty String/Path?(string/path=w131) -> (empty?=w132:bool)
      n187 = Concatenate Strings(w170, "\\", w131) -> (w171:string)
      n188 = String To Path(string=w171) -> (path=w130:path)
      n189 = Select(t=w128, s=w132, f=w130) -> (s? t:f=w129:path)
      n190 = call "Vision Acquisition2"("Image Path"=w129) -> ("Image Out"=w164:T2)  [unwired: 25 in, 1 out]
      n191 = local write "Image File"(w129) -> ()
      n192 = local write "Image Out"(w164) -> ()
      n193 = local write "Image Out 2"(w164) -> ()
      n194 = local write "Image Name"(w131) -> ()
    }
    frame #2 {
      n195 = while {
        stop <- w613 stop-if-true
        w510 = "/"
        w563 = FALSE
        w561 = 0
        n196 = local read "Date Recorded"() -> (w513:string)
        n197 = local read "Ramp (s):"() -> (w480:dbl)
        n198 = local read "RPM:"() -> (w481:dbl)
        n199 = local read "Sat Vg Array-Used"() -> (w469:dbl[])
        n200 = local read "New: Dielectric"() -> (w454:dbl)
        n201 = local read "New: Length"() -> (w470:dbl)
        n202 = local read "New: Width"() -> (w472:dbl)
        n203 = local read "Sat Id-Used"() -> (w468:dbl[])
        n204 = local read "Lin-Vg Array-Used"() -> (w463:dbl[])
        n205 = Divide(x=w481, y=w480) -> (x/y=w479:dbl)
        n206 = local read "Sat Id-Log-Used"() -> (w467:dbl[])
        n207 = local read "New: Dielectric"() -> (w460:dbl)
        n208 = Match Pattern(string=w513, regular expression=w510) -> (before substring=w504:string, after substring=w511:string)  [unwired: 1 in, 2 out]
        n209 = local read "Vg Array-Log-Used"() -> (w466:dbl[])
        n210 = local read "New: Length"() -> (w462:dbl)
        n211 = local write "Accel (RPM/s):"(w479) -> ()
        n212 = local read "New: Width"() -> (w459:dbl)
        n213 = local read "Lin Id-Used"() -> (w464:dbl[])
        n214 = local read "New: Dielectric"() -> (w456:dbl)
        n215 = local read "Lin Vd"() -> (w458:dbl)
        n216 = String Length(string=w504) -> (length=w507:i32)
        n217 = Match Pattern(string=w511, regular expression=w510) -> (before substring=w498:string, after substring=w509:string)  [unwired: 1 in, 2 out]
        n218 = Equal?(x=w507, y=2) -> (x = y?=w505:bool)
        n219 = call "Mobility-Vt-Used Pts_Saturation.vi"("Width"=w472, "Length"=w470, "Dielectric (d)"=w454, "Sat Id Used"=w468, "Vg Used"=w469) -> ("Vt"=w455:dbl, "Mobility"=w471:dbl)  [unwired: 4 in, 1 out]
        n220 = String Length(string=w498) -> (length=w500:i32)
        n221 = call "Mobility-Vt-Used Pts_Linear.vi"("Width"=w459, "Length"=w462, "Vd"=w458, "Dielectric (d)"=w460, "Sat Id Used"=w464, "Vg Used"=w463) -> ("Vt"=w465:dbl, "Mobility"=w461:dbl)  [unwired: 3 in, 1 out]
        n222 = call "STS-Used.vi"("Id Used"=w467, "Vg-Used"=w466) -> ("STS"=w457:dbl)  [unwired: 9 in]
        n223 = case shown="False" w505 {
          tunnel: w504 -> [w639 w641]
          tunnel: [w638 w641] -> w503
          frame False {
            n224 = Concatenate Strings("0", w639) -> (w638:string)
          }
          frame True {
          }
        }
        n225 = local write "New: Mobility-Sat"(w471) -> ()
        n226 = Equal?(x=w500, y=2) -> (x = y?=w502:bool)
        n227 = local write "New: VT-Sat"(w455) -> ()
        n228 = local write "New: Mobility-Lin"(w461) -> ()
        n229 = local write "New: VT-Lin"(w465) -> ()
        n230 = case shown="False" w502 {
          tunnel: w498 -> [w635 w637]
          tunnel: [w634 w637] -> w499
          frame False {
            n231 = Concatenate Strings("0", w635) -> (w634:string)
          }
          frame True {
          }
        }
        n232 = call "Trap Density_VT.vi"("VT"=w455, "Dielectric"=w454) -> ("Trap Density-VT"=w453:dbl)
        n233 = local write "New: STS"(w457) -> ()
        n234 = local write "New: Trap Density-VT"(w453) -> ()
        n235 = local read "Index"() -> (w483:string)
        n236 = local read "Index"() -> (w497:string)
        n237 = local read "Manual-Temp"() -> (w450:bool)
        n238 = local read "Wait Time (s):"() -> (w543:dbl)
        n239 = local read "Rec: Temp"() -> (w451:dbl)
        n240 = String Subset(string=w483, length (rest)=1) -> (substring=w538:string)  [unwired: 1 in]
        n241 = local write "Row"(w538) -> ()
        n242 = local read "Treatment Concentration (mM):"() -> (w491:dbl)
        n243 = case shown="False" w450 {
          tunnel: w451 -> [w623 _]
          tunnel: [w620 w627] -> w449
          frame False {
            n244 = local read "Rec: Temp"() -> (w621:dbl)
            n245 = property on="New: Temp" class="DigNum (strict)"("DisabledEnum"=1) -> ()  [unwired: 2 in, 2 out]
            n246 = Equal To 0?(x=w621) -> (x = 0?=w622:bool)
            n247 = local write "New: Temp"(w623) -> ()
            n248 = case shown="True" w622 {
              tunnel: [w624 w625] -> w620
              tunnel: w621 -> [w624 _]
              frame False {
              }
              frame True {
                n249 = local read "Room Temp"() -> (w625:dbl)
              }
            }
            n250 = local write "New: Temp"(w620) -> ()
          }
          frame True {
            n251 = property on="New: Temp" class="DigNum (strict)"("DisabledEnum"=0) -> ()  [unwired: 2 in, 2 out]
            n252 = local read "New: Temp"() -> (w627:dbl)
          }
        }
        n253 = call "Trap Density_STS.vi"("Temp (T) [K]"=w449, "S.T.S. (S)"=w457, "Dielectric"=w456) -> ("Trap Density (N)"=w452:dbl)  [unwired: 8 in]
        n254 = local write "New: Trap Density-STS"(w452) -> ()
        n255 = local read "Rec: Concentration"() -> (w478:dbl)
        n256 = local read "Relative Humidity (%):"() -> (w488:dbl)
        n257 = String Subset(string=w483, offset (0)=1, length (rest)=2) -> (substring=w539:string)
        n258 = Number To Decimal String(number=w543) -> (decimal integer string=w544:string)  [unwired: 1 in]
        n259 = local read "Solution Temp (C):"() -> (w532:dbl)
        n260 = local read "Surface Treatment:"() -> (w490:string)
        n261 = local read "Room Temp (F):"() -> (w536:dbl)
        n262 = local read "Rec: Material"() -> (w486:string)
        n263 = local write "Column"(w539) -> ()
        n264 = local read "New: Length"() -> (w496:dbl)
        n265 = local read "New: Width"() -> (w495:dbl)
        n266 = local read "New: Mobility-Sat"() -> (w525:dbl)
        n267 = local read "Accel (RPM/s):"() -> (w523:dbl)
        n268 = local read "Sample #:"() -> (w515:dbl)
        n269 = local read "# Drops*:"() -> (w533:dbl)
        n270 = local read "Ramp (s):"() -> (w541:dbl)
        n271 = local read "New: STS"() -> (w517:dbl)
        n272 = local read "Rec: Solvent"() -> (w492:string)
        n273 = local read "New: VT-Sat"() -> (w519:dbl)
        n274 = local read "Rec: On/Off"() -> (w521:dbl)
        n275 = local read "Rec: Method"() -> (w516:string)
        n276 = local read "Time (s):"() -> (w528:dbl)
        n277 = local read "Date Recorded"() -> (w512:string)
        n278 = local read "RPM:"() -> (w529:dbl)
        n279 = local read "Fabricator:"() -> (w537:string)
        n280 = Number To Decimal String(number=w478) -> (decimal integer string=w477:string)  [unwired: 1 in]
        n281 = Number To Decimal String(number=w533) -> (decimal integer string=w534:string)  [unwired: 1 in]
        n282 = Number To Decimal String(number=w515) -> (decimal integer string=w508:string)  [unwired: 1 in]
        n283 = call "DeviceID"("Sample"=w508, "Year"=w509, "Month"=w503, "Day"=w499, "Index"=w497) -> ("Result"=w514:string)  [unwired: 9 in, 1 out]
        n284 = Number To Decimal String(number=w496) -> (decimal integer string=w494:string)  [unwired: 1 in]
        n285 = Number To Decimal String(number=w495) -> (decimal integer string=w493:string)  [unwired: 1 in]
        n286 = Number To Decimal String(number=w532) -> (decimal integer string=w531:string)  [unwired: 1 in]
        n287 = Number To Decimal String(number=w488) -> (decimal integer string=w487:string)  [unwired: 1 in]
        n288 = Number To Decimal String(number=w536) -> (decimal integer string=w535:string)  [unwired: 1 in]
        n289 = property on="Image Out" class="ImageControl"() -> ("ZoomSingle"=w581:cluster{"X":sgl, "Y":sgl})  [unwired: 2 in, 2 out]
        n290 = Number To Decimal String(number=w491) -> (decimal integer string=w489:string)  [unwired: 1 in]
        n291 = property on="Image Out" class="ImageControl"() -> ("Bounds"=w582:T13)  [unwired: 2 in, 2 out]
        n292 = Number To Decimal String(number=w529) -> (decimal integer string=w530:string)  [unwired: 1 in]
        n293 = Number To Fractional String(number=w523) -> (F-format string=w524:string)  [unwired: 3 in]
        n294 = Number To Decimal String(number=w528) -> (decimal integer string=w527:string)  [unwired: 1 in]
        n295 = Number To Fractional String(number=w525) -> (F-format string=w526:string)  [unwired: 3 in]
        n296 = Number To Fractional String(number=w521) -> (F-format string=w522:string)  [unwired: 3 in]
        n297 = Number To Fractional String(number=w519) -> (F-format string=w520:string)  [unwired: 3 in]
        n298 = Number To Fractional String(number=w517) -> (F-format string=w518:string)  [unwired: 3 in]
        n299 = Number To Decimal String(number=w541) -> (decimal integer string=w542:string)  [unwired: 1 in]
        n300 = call <vilib>:"Intialize Keyboard.vi"() -> ("device ID"=w593:refnum<k1>)  [unwired: 10 in, 1 out]
        n301 = property on="Image Out" class="ImageControl"() -> ("Image Center Position"=w588:cluster{"X":u32, "Y":u32})  [unwired: 2 in, 2 out]
        n302 = call-poly <vilib>:"Acquire Input Data.vi"("device ID"=w593) -> ("keys pressed"=w592:T14)  [unwired: 16 in, 2 out]
        n303 = Unbundle(w582) -> ("Width"=w579:u32, "Height"=w578:u32)
        n304 = Unbundle(w581) -> ("X"=w556:sgl, "Y"=w580:sgl)
        n305 = Index Array(array=w592) -> (element=w596:T15)  [unwired: 1 in]
        n306 = event shown="[1] \"Undo Button\": Mouse Down" {
          selector: _ -> [_ _ _ _ _ _ _]
          dyn-events: _ -> [_ _ _ _ _ _ _]
          timeout: 10 -> [_ _ _ _ _ _ _]
          event "Remove Button": Mouse Down {
            w648 = 0
            n307 = event-data() -> ()  [unwired: 1 in, 7 out]
            n308 = property on="Image Out" class="ImageControl"() -> ("ROI"=w646:T12)  [unwired: 2 in, 2 out]
            n309 = Unbundle(w646) -> ("Global Rectangle"=w649:i32[], "Contours"=w651:T16)
            n310 = Reverse 1D Array(array=w649) -> (reversed array=w650:i32[])
            n311 = Reverse 1D Array(array=w651) -> (reversed array=w652:T16)
            n312 = Delete From Array(array=w650, index=w648) -> (array with subset deleted=w653:i32[])  [unwired: 1 in, 1 out]
            n313 = Delete From Array(array=w652, index=w648) -> (array with subset deleted=w654:T16)  [unwired: 1 in, 1 out]
            n314 = Reverse 1D Array(array=w653) -> (reversed array=w655:i32[])
            n315 = Reverse 1D Array(array=w654) -> (reversed array=w656:T16)
            n316 = Bundle(w655, w656) -> (w647:T17)  [unwired: 1 in]
            n317 = local write "ROI Descriptor out"(w646) -> ()
            n318 = local write "ROI Descriptor"(w647) -> ()
            n319 = property on="Image Out" class="ImageControl"("ROI"=w647) -> ()  [unwired: 2 in, 2 out]
          }
          event "Undo Button": Mouse Down {
            n320 = event-data() -> ()  [unwired: 1 in, 7 out]
            n321 = invoke on="Image Out" class="ImageControl" method="Clear ROI"() -> ()  [unwired: 3 in, 3 out]
          }
          event "Image Folder": Value Change {
            n322 = event-data() -> ()  [unwired: 1 in, 5 out]
            n323 = local read "Image File"() -> (w658:path)
            n324 = call "Vision Acquisition"("Image Path"=w658) -> ("Image Out"=w657:T2)  [unwired: 25 in, 1 out]
            n325 = local write "Image Out 2"(w657) -> ()
            n326 = local write "Image Out"(w657) -> ()
            n327 = invoke on="Image Out" class="ImageControl" method="Clear ROI"() -> ()  [unwired: 3 in, 3 out]
          }
          event "Zoom": Value Change {
            n328 = event-data() -> ()  [unwired: 1 in, 5 out]
            n329 = local read "Zoom"() -> (w659:i16)
            n330 = Bundle("Zoom"=w659, "Zoom"=w659) -> (w660:cluster{"Zoom":i16, "Zoom":i16})  [unwired: 1 in]
            n331 = property on="Image Out" class="ImageControl"("ZoomInteger"=w660) -> ()  [unwired: 2 in, 2 out]
          }
          event Timeout {
            n332 = event-data() -> ()  [unwired: 1 in, 2 out]
          }
          event "Image Out": Mouse Enter {
            (unwired) 6
            n333 = event-data() -> ()  [unwired: 1 in, 3 out]
            n334 = call "Simulate_Keyboard.vi"("Action"=0, "Virtual Key"=162) -> ()  [unwired: 7 in, 1 out]
          }
          event "Image Out": Mouse Leave {
            n335 = event-data() -> ()  [unwired: 1 in, 3 out]
            n336 = flat-sequence {
              frame #0 {
                n337 = Wait (ms)(milliseconds to wait=10) -> ()  [unwired: 1 out]
              }
              frame #1 {
                (unwired) 6
                n338 = call "Simulate_Keyboard.vi"("Action"=2, "Virtual Key"=162) -> ()  [unwired: 7 in, 1 out]
              }
            }
          }
        }
        n339 = Divide(x=w579, y=w556) -> (x/y=w569:sgl)
        n340 = Multiply(x=w569, y=0.5) -> (x*y=w575:dbl)
        n341 = Divide(x=w578, y=w580) -> (x/y=w568:sgl)
        n342 = Multiply(x=w568, y=0.5) -> (x*y=w574:dbl)
        n343 = Unbundle(w588) -> ("X"=w570:u32, "Y"=w571:u32)
        n344 = Subtract(x=w571, y=w574) -> (x-y=w572:dbl)
        n345 = Subtract(x=w570, y=w575) -> (x-y=w573:dbl)
        n346 = Add(x=w573, y=w569) -> (x+y=w587:dbl)
        n347 = Add(x=w572, y=w568) -> (x+y=w586:dbl)
        n348 = Build Array(w514, w537, w516, w512, w508, w538, w539, w494, w493, w486, w490, w489, w492, w477, w531, w534, w544, w535, w487, w542, w530, w524, w527, w526, w522, w520, w518) -> (w540:string[])
        n349 = local write "Current \nRecord"(w540) -> ()
        n350 = Reciprocal(x=w556) -> (1/x=w555:sgl)
        n351 = event shown="[12] \"Save Changes? 2\": Mouse Down" {
          selector: _ -> [_ _ _ _ _ _ _ _ _ _ _ _ _ _ _ _]
          dyn-events: _ -> [_ _ _ _ _ _ _ _ _ _ _ _ _ _ _ _]
          timeout: 10 -> [_ _ _ _ _ _ _ _ _ _ _ _ _ _ _ _]
          tunnel: [_ _ _ _ _ _ _ _ _ _ _ _ _ TRUE _ TRUE] -> w613
          event Timeout {
            n352 = event-data() -> ()  [unwired: 1 in, 2 out]
          }
          event "Down Button": Mouse Down {
            w1005 = 0
            n353 = event-data() -> ()  [unwired: 1 in, 7 out]
            n354 = local read "Transfer File"() -> (w1010:path)
            n355 = Strip Path(path=w1010) -> (stripped path=w1001:path, name=w1019:string)
            n356 = local write "Transfer Folder"(w1001) -> ()
            n357 = List Folder(path=w1001) -> (filenames=w1015:string[], error out=w955:errorcluster)  [unwired: 3 in, 2 out]
            n358 = local read "Folder Index"() -> (w957:dbl)
            n359 = Array Size(array=w1015) -> (size(s)=w1011:i32)
            n360 = Search 1D Array(1D array=w1015, element=w1019) -> (index of element=w1012:i32)  [unwired: 1 in]
            n361 = property on="Image Out" class="ImageControl"() -> (error out=w958:errorcluster, "Image Center Position"=w962:cluster{"X":u32, "Y":u32})  [unwired: 2 in, 1 out]
            n362 = Decrement(x=w1011) -> (x-1=w1013:i32)
            n363 = Equal?(x=w1012, y=w1013) -> (x = y?=w1014:bool)
            n364 = invoke on="Image Out" class="ImageControl" method="Clear ROI"() -> ()  [unwired: 3 in, 3 out]
            n365 = case shown="False" w1014 {
              tunnel: w957 -> [w1172 _]
              tunnel: [w1171 0] -> w956
              tunnel: w955 -> [w1170 w1173]
              tunnel: [w1170 w1173] -> w954
              frame False {
                n366 = Increment(x=w1172) -> (x+1=w1171:dbl)
              }
              frame True {
              }
            }
            n367 = Unbundle(w962) -> ("X"=w960:u32)  [unwired: 1 out]
            n368 = local write "Folder Index"(w956) -> ()
            n369 = Bundle("X"=w960, 0) -> (w961:cluster{"X":u32, i32})  [unwired: 1 in]
            n370 = property on="Image Out" class="ImageControl"(error in=w958, "Image Center Position"=w961) -> ()  [unwired: 1 in, 2 out]
            n371 = Path To String(path=w1001) -> (string=w1020:string)
            n372 = Index Array(array=w1015, index=w956) -> (element=w1016:string)
            n373 = local write "Data Name:"(w1016) -> ()
            n374 = Concatenate Strings(w1020, "\\", w1016) -> (w1018:string)
            n375 = String To Path(string=w1018) -> (path=w929:path)
            n376 = call "Recorded Values.vi"("Path"=w929) -> ("Recorded Char"=w1022:T6, "Recorded Prop"=w1023:T7, "Fabrication Prop"=w1021:T8)  [unwired: 8 in]
            n377 = Unbundle By Name(w1022) -> ("Mobility-Sat"=w1035:dbl, "Moblitity-Lin"=w1036:dbl, "On/Off"=w1037:dbl, "Off Current"=w1038:dbl, "Vt-Sat"=w924:dbl, "STS"=w1039:dbl, "Trap Density-VT"=w1040:dbl, "Trap Density-STS"=w1041:dbl)
            n378 = Unbundle By Name(w1021) -> ("Date Created"=w1042:string, "Material"=w1024:string, "Solvent"=w1025:string, "Concentration"=w1026:dbl, "Method"=w1027:string, "Dielectric (nm)"=w1028:dbl, "Treatment"=w1029:string, "Comments"=w1030:string)
            n379 = Unbundle By Name(w1023) -> ("Date Recorded"=w1031:string, "Index"=w1032:string, "Length"=w1033:dbl, "Width"=w1034:dbl, "Sample Temp"=w926:dbl)
            n380 = local write "Date Created"(w1042) -> ()
            n381 = local write "Rec: Off I-Sat"(w1038) -> ()
            n382 = local write "Rec: Comments"(w1030) -> ()
            n383 = local write "Rec: Material"(w1024) -> ()
            n384 = local write "Rec: VT-Sat"(w924) -> ()
            n385 = local write "Rec: Concentration"(w1026) -> ()
            n386 = local write "Rec: Method"(w1027) -> ()
            n387 = local write "Rec: Dielectric (d)"(w1028) -> ()
            n388 = local write "Surface Treatment:"(w1029) -> ()
            n389 = local write "Index"(w1032) -> ()
            n390 = local write "Rec: Mobility-Sat"(w1035) -> ()
            n391 = local write "Rec: Mobility-Lin"(w1036) -> ()
            n392 = local write "Rec: On/Off"(w1037) -> ()
            n393 = local write "Rec: STS"(w1039) -> ()
            n394 = local write "Rec: Trap Density-VT"(w1040) -> ()
            n395 = local write "Rec: Trap Density-STS"(w1041) -> ()
            n396 = local write "Rec: Solvent"(w1025) -> ()
            n397 = local write "Date Recorded"(w1031) -> ()
            n398 = local write "Rec: Length"(w1033) -> ()
            n399 = local write "Rec: Width"(w1034) -> ()
            n400 = local write "Rec: Temp"(w926) -> ()
            n401 = Equal To 0?(x=w926) -> (x = 0?=w927:bool)
            n402 = case shown="True" w927 {
              tunnel: [w1043 w1044] -> w925
              tunnel: w926 -> [w1043 _]
              frame False {
              }
              frame True {
                n403 = local read "Room Temp"() -> (w1044:dbl)
              }
            }
            n404 = local read "NumPoints Log"() -> (w950:dbl)
            n405 = local write "Transfer File"(w929) -> ()
            n406 = local read "Num Pts"() -> (w953:dbl)
            n407 = call-poly <vilib>:"Read From Spreadsheet File.vi"("file path (dialog if empty)"=w929) -> ("all rows"=w1007:string[][])  [unwired: 6 in, 4 out]
            n408 = call "Mobility-Vt Calculator-File.vi"("NumPts"=w953, "Path"=w929) -> ("Graph Cluster"=w922:T9, "Output"=w952:T10, "Index-Sat"=w951:dbl, "Index-Lin"=w937:dbl)  [unwired: 5 in, 1 out]
            n409 = local read "New: Dielectric"() -> (w934:dbl)
            n410 = call "STS Calculator-File.vi"("NumPts"=w950, "Path"=w929) -> ("STS Index-Sat"=w949:dbl, "XY Graph-Sat"=w948:cluster{dbl[], dbl[]}[], "Ouput"=w947:cluster{"STS-Sat":dbl, "STS-Lin":dbl})  [unwired: 5 in, 2 out]
            n411 = local write "Sat-Trans Slider"(w951) -> ()
            n412 = Unbundle By Name(w952) -> ("Mobility-Sat"=w946:dbl, "Vt-Sat"=w933:dbl, "Mobility-Lin"=w945:dbl, "Vt-Lin"=w944:dbl, "Off I-Sat"=w930:dbl, "On/Off I-Sat"=w923:dbl)
            n413 = Unbundle By Name(w947) -> ("STS-Sat"=w928:dbl)  [unwired: 1 out]
            n414 = local write "Index 2"(w949) -> ()
            n415 = local write "MobVi Index"(w951) -> ()
            n416 = local write "Log-Sat"(w948) -> ()
            n417 = Array Size(array=w1007) -> (size(s)=w1006:i32[])
            n418 = Unbundle By Name(w922) -> ("Raw Sat"=w919:cluster{dbl[], dbl[]}[], "Sqrt Sat"=w921:cluster{dbl[], dbl[]}[], "Log Sat"=w918:cluster{dbl[], dbl[]}[], "Raw Lin"=w917:cluster{dbl[], dbl[]}[], "Sqrt Lin"=w920:cluster{dbl[], dbl[]}[], "Log Lin"=w916:cluster{dbl[], dbl[]}[])
            n419 = local write "Sqrt-Sat"(w921) -> ()
            n420 = call "Trap Density_VT.vi"("VT"=w933, "Dielectric"=w934) -> ("Trap Density-VT"=w932:dbl)
            n421 = call "Trap Density_STS.vi"("Temp (T) [K]"=w925, "S.T.S. (S)"=w928, "Dielectric"=w934) -> ("Trap Density (N)"=w931:dbl)  [unwired: 8 in]
            n422 = local write "New: STS"(w928) -> ()
            n423 = local write "Calc: STS"(w928) -> ()
            n424 = local write "Calc: Mobility-Sat"(w946) -> ()
            n425 = local write "Calc: Off I-Sat"(w944) -> ()
            n426 = local write "Calc: Mobility-Lin"(w945) -> ()
            n427 = Index Array(array=w1006, index=w1005) -> (element=w987:i32)
            n428 = Decimate 1D Array(w948) -> (w981:cluster{dbl[], dbl[]}[])  [unwired: 1 out]
            n429 = Decimate 1D Array(w921) -> (w991:cluster{dbl[], dbl[]}[])  [unwired: 1 out]
            n430 = local write "Calc: Off I-Sat"(w930) -> ()
            n431 = local write "Calc: On/Off"(w923) -> ()
            n432 = Decimate 1D Array(w920) -> (w943:cluster{dbl[], dbl[]}[])  [unwired: 1 out]
            n433 = local write "Calc: VT-Sat"(w933) -> ()
            n434 = Array Subset(array=w1007, index (row)=w1005, index (col)=w1005, length (col)=3) -> (w1008:string[][])  [unwired: 1 in]
            n435 = local write "Calc: Trap Density-VT"(w932) -> ()
            n436 = local write "Calc: Trap Density-STS"(w931) -> ()
            n437 = local write "New: Trap Density-STS"(w931) -> ()
            n438 = local write "New: Trap Density-VT"(w932) -> ()
            n439 = Array To Cluster(array=w981) -> (cluster=w979:T11)
            n440 = Array To Cluster(array=w991) -> (cluster=w993:T11)
            n441 = local write "Raw- Sat"(w919) -> ()
            n442 = local write "Sqrt-Lin"(w920) -> ()
            n443 = local write "Raw- Lin"(w917) -> ()
            n444 = local write "Log-Sat"(w918) -> ()
            n445 = local write "New: VT-Lin"(w944) -> ()
            n446 = local write "Log-Lin"(w916) -> ()
            n447 = local write "New: VT-Sat"(w933) -> ()
            n448 = local write "New: Mobility-Sat"(w946) -> ()
            n449 = local write "New: Mobility-Lin"(w945) -> ()
            n450 = Reshape Array(w1008, w987) -> (w994:string[])
            n451 = Array To Cluster(array=w943) -> (cluster=w942:T11)
            n452 = Subtract(x=w987, y=20) -> (x-y=w986:i32)
            n453 = property on="Sat-Trans Slider" class="Slide (strict)"("Scale.Maximum"=w986) -> ()  [unwired: 2 in, 2 out]
            n454 = Unbundle(w979) -> ("[0]"=w980:cluster{dbl[], dbl[]})  [unwired: 8 out]
            n455 = Unbundle(w993) -> ("[0]"=w992:cluster{dbl[], dbl[]})  [unwired: 8 out]
            n456 = Unbundle(w942) -> ("[0]"=w939:cluster{dbl[], dbl[]})  [unwired: 8 out]
            n457 = Search 1D Array(1D array=w994, element="Index:") -> (index of element=w1002:i32)  [unwired: 1 in]
            n458 = local read "Num Pts"() -> (w938:dbl)
            n459 = Unbundle(w939) -> (w941:dbl[], w940:dbl[])
            n460 = Increment(x=w1002) -> (x+1=w1003:i32)
            n461 = Unbundle(w980) -> (w978:dbl[], w977:dbl[])
            n462 = Unbundle(w992) -> (w983:dbl[], w982:dbl[])
            n463 = Array Subset(array=w941, index=w937, length=w938) -> (w936:dbl[])
            n464 = Array Subset(array=w940, index=w937, length=w938) -> (w935:dbl[])
            n465 = Array Subset(array=w978, index=w949, length=w950) -> (w985:dbl[])
            n466 = Array Subset(array=w977, index=w949, length=w950) -> (w984:dbl[])
            n467 = Array Subset(array=w983, index=w951, length=w953) -> (w990:dbl[])
            n468 = Array Subset(array=w982, index=w951, length=w953) -> (w989:dbl[])
            n469 = Index Array(array=w994, index=w1003) -> (element=w966:string)
            n470 = local write "Lin-Vg Array-Used"(w936) -> ()
            n471 = local write "Sat Vg Array-Used"(w990) -> ()
            n472 = local write "Vg Array-Log-Used"(w984) -> ()
            n473 = local write "Lin Id-Used"(w935) -> ()
            n474 = local read "Image Folder"() -> (w964:path)
            n475 = local write "Sat Id-Used"(w989) -> ()
            n476 = local write "Sat Id-Log-Used"(w985) -> ()
            n477 = List Folder(path=w964, error in=w954) -> (filenames=w1000:string[], error out=w967:errorcluster)  [unwired: 2 in, 2 out]
            n478 = while {
              tunnel: w1000 -> [w1057]
              tunnel: w966 -> [w1055]
              tunnel: [w1054] -> _
              tunnel: [w1054] -> w999
              tunnel: w987 -> [w1053]
              i -> [w1054]
              stop <- w1050 stop-if-true
              n479 = Index Array(array=w1057, index=w1054) -> (element=w1058:string)
              n480 = xnode "Match Regular Expression"("input string"=w1058, "regular expression"=w1055) -> ("whole match"=w1056:string)  [unwired: 4 in, 4 out]
              n481 = Equal?(x=w1056, y=w1055) -> (x = y?=w1052:bool)
              n482 = Equal?(x=w1053, y=w1054) -> (x = y?=w1051:bool)
              n483 = Or(x=w1052, y=w1051) -> (x .or. y?=w1050:bool)
            }
            n484 = Build Path(base path=w964, name or relative path="ROI") -> (appended path=w963:path)
            n485 = Path To String(path=w964) -> (string=w997:string)
            n486 = Index Array(array=w1000, index=w999) -> (element=w975:string)
            n487 = invoke on="Image Out" class="ImageControl" method="Clear ROI"(error in=w967) -> (error out=w970:errorcluster)  [unwired: 2 in, 2 out]
            n488 = local write "Image Name"(w975) -> ()
            n489 = Build Path(base path=w963, name or relative path=w966) -> (appended path=w971:path)
            n490 = call <vilib>:"Check if File or Folder Exists.vi"("error in (no error)"=w970, "path"=w971) -> ("file or folder exists?"=w968:bool, "dup path"=w969:path)  [unwired: 7 in, 1 out]
            n491 = Concatenate Strings(w997, "\\", w975) -> (w996:string)
            n492 = case shown="False" w968 {
              tunnel: w969 -> [_ w1045]
              frame False {
              }
              frame True {
                n493 = Read from Text File(file (use dialog)=w1045) -> (text=w1049:string)  [unwired: 3 in, 3 out]
                n494 = property on="Image Out" class="ImageControl"() -> ("ROI"=w1046:T12)  [unwired: 2 in, 2 out]
                n495 = Unflatten From String(type=w1046, binary string=w1049) -> (value=w1047:T12, error out=w1048:errorcluster)  [unwired: 3 in, 1 out]
                n496 = property on="Image Out" class="ImageControl"(error in=w1048, "ROI"=w1047) -> ()  [unwired: 1 in, 2 out]
              }
            }
            n497 = String To Path(string=w996) -> (path=w974:path)
            n498 = Empty String/Path?(string/path=w975) -> (empty?=w976:bool)
            n499 = local read "No Image File"() -> (w972:path)
            n500 = Select(t=w972, s=w976, f=w974) -> (s? t:f=w973:path)
            n501 = local write "Image File"(w973) -> ()
            n502 = call "Vision Acquisition4"("Image Path"=w973) -> ("Image Out"=w998:T2)  [unwired: 25 in, 1 out]
            n503 = local write "Image Out"(w998) -> ()
            n504 = local write "Image Out 2"(w998) -> ()
          }
          event "Transfer File": Value Change {
            w1286 = 0
            n505 = event-data() -> ()  [unwired: 1 in, 5 out]
            n506 = local read "Transfer File"() -> (w1282:path)
            n507 = Strip Path(path=w1282) -> (stripped path=w1281:path, name=w1295:string)
            n508 = local write "Transfer Folder"(w1281) -> ()
            n509 = property on="Image Out" class="ImageControl"() -> (error out=w1237:errorcluster, "Image Center Position"=w1241:cluster{"X":u32, "Y":u32})  [unwired: 2 in, 1 out]
            n510 = List Folder(path=w1281) -> (filenames=w1291:string[], error out=w1247:errorcluster)  [unwired: 3 in, 2 out]
            n511 = Search 1D Array(1D array=w1291, element=w1295) -> (index of element=w1236:i32)  [unwired: 1 in]
            n512 = local write "Folder Index"(w1236) -> ()
            n513 = Unbundle(w1241) -> ("X"=w1239:u32)  [unwired: 1 out]
            n514 = Path To String(path=w1281) -> (string=w1296:string)
            n515 = Index Array(array=w1291, index=w1236) -> (element=w1292:string)
            n516 = Bundle("X"=w1239, 0) -> (w1240:cluster{"X":u32, i32})  [unwired: 1 in]
            n517 = local write "Data Name:"(w1292) -> ()
            n518 = property on="Image Out" class="ImageControl"(error in=w1237, "Image Center Position"=w1240) -> ()  [unwired: 1 in, 2 out]
            n519 = Concatenate Strings(w1296, "\\", w1292) -> (w1294:string)
            n520 = String To Path(string=w1294) -> (path=w1188:path)
            n521 = call "Recorded Values.vi"("Path"=w1188) -> ("Recorded Char"=w1234:T6, "Recorded Prop"=w1233:T7, "Fabrication Prop"=w1235:T8)  [unwired: 8 in]
            n522 = Unbundle By Name(w1234) -> ("Mobility-Sat"=w1221:dbl, "Moblitity-Lin"=w1220:dbl, "On/Off"=w1219:dbl, "Off Current"=w1218:dbl, "Vt-Sat"=w1184:dbl, "STS"=w1217:dbl, "Trap Density-VT"=w1216:dbl, "Trap Density-STS"=w1215:dbl)
            n523 = Unbundle By Name(w1235) -> ("Date Created"=w1214:string, "Material"=w1232:string, "Solvent"=w1231:string, "Concentration"=w1230:dbl, "Method"=w1229:string, "Dielectric (nm)"=w1228:dbl, "Treatment"=w1227:string, "Comments"=w1226:string)
            n524 = Unbundle By Name(w1233) -> ("Date Recorded"=w1225:string, "Index"=w1224:string, "Length"=w1223:dbl, "Width"=w1222:dbl, "Sample Temp"=w1186:dbl)
            n525 = local write "Date Created"(w1214) -> ()
            n526 = local write "Rec: Material"(w1232) -> ()
            n527 = local write "Rec: Off I-Sat"(w1218) -> ()
            n528 = local write "Rec: Comments"(w1226) -> ()
            n529 = local write "Rec: VT-Sat"(w1184) -> ()
            n530 = local write "Rec: Concentration"(w1230) -> ()
            n531 = local write "Rec: Method"(w1229) -> ()
            n532 = local write "Rec: Dielectric (d)"(w1228) -> ()
            n533 = local write "Surface Treatment:"(w1227) -> ()
            n534 = local write "Index"(w1224) -> ()
            n535 = local write "Rec: Mobility-Sat"(w1221) -> ()
            n536 = local write "Rec: Mobility-Lin"(w1220) -> ()
            n537 = local write "Rec: On/Off"(w1219) -> ()
            n538 = local write "Rec: STS"(w1217) -> ()
            n539 = local write "Rec: Trap Density-VT"(w1216) -> ()
            n540 = local write "Rec: Trap Density-STS"(w1215) -> ()
            n541 = local write "Rec: Solvent"(w1231) -> ()
            n542 = local write "Date Recorded"(w1225) -> ()
            n543 = local write "Rec: Length"(w1223) -> ()
            n544 = local write "Rec: Width"(w1222) -> ()
            n545 = local write "Rec: Temp"(w1186) -> ()
            n546 = Equal To 0?(x=w1186) -> (x = 0?=w1187:bool)
            n547 = case shown="False" w1187 {
              tunnel: [w1297 w1298] -> w1185
              tunnel: w1186 -> [w1297 _]
              frame False {
              }
              frame True {
                n548 = local read "Room Temp"() -> (w1298:dbl)
              }
            }
            n549 = local read "NumPoints Log"() -> (w1210:dbl)
            n550 = local write "Transfer File"(w1188) -> ()
            n551 = local read "Num Pts"() -> (w1211:dbl)
            n552 = call-poly <vilib>:"Read From Spreadsheet File.vi"("file path (dialog if empty)"=w1188) -> ("all rows"=w1288:string[][])  [unwired: 6 in, 4 out]
            n553 = local read "New: Dielectric"() -> (w1194:dbl)
            n554 = call "STS Calculator-File.vi"("NumPts"=w1210, "Path"=w1188) -> ("STS Index-Sat"=w1208:dbl, "XY Graph-Sat"=w1209:cluster{dbl[], dbl[]}[], "Ouput"=w1207:cluster{"STS-Sat":dbl, "STS-Lin":dbl})  [unwired: 5 in, 2 out]
            n555 = call "Mobility-Vt Calculator-File.vi"("NumPts"=w1211, "Path"=w1188) -> ("Graph Cluster"=w1181:T9, "Output"=w1212:T10, "Index-Sat"=w1213:dbl, "Index-Lin"=w1200:dbl)  [unwired: 5 in, 1 out]
            n556 = Unbundle By Name(w1212) -> ("Mobility-Sat"=w1196:dbl, "Vt-Sat"=w1190:dbl, "Mobility-Lin"=w1195:dbl, "Vt-Lin"=w1182:dbl, "Off I-Sat"=w1189:dbl, "On/Off I-Sat"=w1183:dbl)
            n557 = local write "Index 2"(w1208) -> ()
            n558 = Unbundle By Name(w1207) -> ("STS-Sat"=w1191:dbl)  [unwired: 1 out]
            n559 = local write "MobVi Index"(w1213) -> ()
            n560 = local write "Log-Sat"(w1209) -> ()
            n561 = local write "Sat-Trans Slider"(w1213) -> ()
            n562 = Array Size(array=w1288) -> (size(s)=w1287:i32[])
            n563 = call "Trap Density_VT.vi"("VT"=w1190, "Dielectric"=w1194) -> ("Trap Density-VT"=w1193:dbl)
            n564 = call "Trap Density_STS.vi"("Temp (T) [K]"=w1185, "S.T.S. (S)"=w1191, "Dielectric"=w1194) -> ("Trap Density (N)"=w1192:dbl)  [unwired: 8 in]
            n565 = local write "Calc: Mobility-Lin"(w1195) -> ()
            n566 = local write "Calc: Mobility-Sat"(w1196) -> ()
            n567 = local write "Calc: VT-Sat"(w1190) -> ()
            n568 = local write "Calc: Off I-Sat"(w1189) -> ()
            n569 = local write "Calc: VT-Lin"(w1182) -> ()
            n570 = local write "Calc: On/Off"(w1183) -> ()
            n571 = local write "Calc: STS"(w1191) -> ()
            n572 = Unbundle By Name(w1181) -> ("Raw Sat"=w1178:cluster{dbl[], dbl[]}[], "Sqrt Sat"=w1179:cluster{dbl[], dbl[]}[], "Log Sat"=w1177:cluster{dbl[], dbl[]}[], "Raw Lin"=w1176:cluster{dbl[], dbl[]}[], "Sqrt Lin"=w1180:cluster{dbl[], dbl[]}[], "Log Lin"=w1175:cluster{dbl[], dbl[]}[])
            n573 = Decimate 1D Array(w1180) -> (w1206:cluster{dbl[], dbl[]}[])  [unwired: 1 out]
            n574 = local write "Calc: Trap Density-VT"(w1193) -> ()
            n575 = local write "Calc: Trap Density-STS"(w1192) -> ()
            n576 = local write "New: Trap Density-STS"(w1192) -> ()
            n577 = local write "New: Trap Density-VT"(w1193) -> ()
            n578 = local write "Sqrt-Lin"(w1180) -> ()
            n579 = local write "New: VT-Sat"(w1190) -> ()
            n580 = Decimate 1D Array(w1209) -> (w1262:cluster{dbl[], dbl[]}[])  [unwired: 1 out]
            n581 = Index Array(array=w1287, index=w1286) -> (element=w1268:i32)
            n582 = Decimate 1D Array(w1179) -> (w1271:cluster{dbl[], dbl[]}[])  [unwired: 1 out]
            n583 = local write "Sqrt-Sat"(w1179) -> ()
            n584 = local write "New: Mobility-Lin"(w1195) -> ()
            n585 = Array Subset(array=w1288, index (row)=w1286, index (col)=w1286, length (col)=3) -> (w1289:string[][])  [unwired: 1 in]
            n586 = local write "New: VT-Lin"(w1182) -> ()
            n587 = Array To Cluster(array=w1206) -> (cluster=w1205:T11)
            n588 = local write "New: STS"(w1191) -> ()
            n589 = local write "New: Mobility-Sat"(w1196) -> ()
            n590 = Array To Cluster(array=w1262) -> (cluster=w1260:T11)
            n591 = Array To Cluster(array=w1271) -> (cluster=w1273:T11)
            n592 = Reshape Array(w1289, w1268) -> (w1274:string[])
            n593 = Subtract(x=w1268, y=20) -> (x-y=w1266:i32)
            n594 = local write "Raw- Sat"(w1178) -> ()
            n595 = Unbundle(w1205) -> ("[0]"=w1204:cluster{dbl[], dbl[]})  [unwired: 8 out]
            n596 = local write "Raw- Lin"(w1176) -> ()
            n597 = local write "Log-Sat"(w1177) -> ()
            n598 = local read "Num Pts"() -> (w1201:dbl)
            n599 = property on="Sat-Trans Slider" class="Slide (strict)"("Scale.Maximum"=w1266) -> ()  [unwired: 2 in, 2 out]
            n600 = local write "Log-Lin"(w1175) -> ()
            n601 = Unbundle(w1204) -> (w1203:dbl[], w1202:dbl[])
            n602 = Unbundle(w1260) -> ("[0]"=w1261:cluster{dbl[], dbl[]})  [unwired: 8 out]
            n603 = Unbundle(w1273) -> ("[0]"=w1272:cluster{dbl[], dbl[]})  [unwired: 8 out]
            n604 = Search 1D Array(1D array=w1274, element="Index:") -> (index of element=w1283:i32)  [unwired: 1 in]
            n605 = local read "Num Pts"() -> (w1197:dbl)
            n606 = Array Subset(array=w1203, index=w1200, length=w1201) -> (w1199:dbl[])
            n607 = Array Subset(array=w1202, index=w1200, length=w1201) -> (w1198:dbl[])
            n608 = Increment(x=w1283) -> (x+1=w1284:i32)
            n609 = Unbundle(w1261) -> (w1258:dbl[], w1257:dbl[])
            n610 = Unbundle(w1272) -> (w1259:dbl[], w1263:dbl[])
            n611 = local read "Image Folder"() -> (w1243:path)
            n612 = local write "Lin-Vg Array-Used"(w1199) -> ()
            n613 = Array Subset(array=w1258, index=w1208, length=w1210) -> (w1265:dbl[])
            n614 = Array Subset(array=w1257, index=w1208, length=w1210) -> (w1264:dbl[])
            n615 = Array Subset(array=w1259, index=w1213, length=w1197) -> (w1270:dbl[])
            n616 = Array Subset(array=w1263, index=w1213, length=w1197) -> (w1269:dbl[])
            n617 = Index Array(array=w1274, index=w1284) -> (element=w1245:string)
            n618 = local write "Lin Id-Used"(w1198) -> ()
            n619 = local write "Sat Vg Array-Used"(w1270) -> ()
            n620 = local write "Vg Array-Log-Used"(w1264) -> ()
            n621 = local write "Sat Id-Log-Used"(w1265) -> ()
            n622 = local write "Sat Id-Used"(w1269) -> ()
            n623 = local write "Index"(w1245) -> ()
            n624 = List Folder(path=w1243, error in=w1247) -> (filenames=w1279:string[], error out=w1246:errorcluster)  [unwired: 2 in, 2 out]
            n625 = Build Path(base path=w1243, name or relative path="ROI") -> (appended path=w1242:path)
            n626 = invoke on="Image Out" class="ImageControl" method="Clear ROI"(error in=w1246) -> (error out=w1250:errorcluster)  [unwired: 2 in, 2 out]
            n627 = Build Path(base path=w1242, name or relative path=w1245) -> (appended path=w1251:path)
            n628 = while {
              tunnel: w1279 -> [w1311]
              tunnel: w1245 -> [w1309]
              tunnel: [w1308] -> _
              tunnel: [w1308] -> w1278
              tunnel: w1268 -> [w1307]
              i -> [w1308]
              stop <- w1304 stop-if-true
              n629 = Index Array(array=w1311, index=w1308) -> (element=w1312:string)
              n630 = xnode "Match Regular Expression"("input string"=w1312, "regular expression"=w1309) -> ("whole match"=w1310:string)  [unwired: 4 in, 4 out]
              n631 = Equal?(x=w1310, y=w1309) -> (x = y?=w1306:bool)
              n632 = Equal?(x=w1307, y=w1308) -> (x = y?=w1305:bool)
              n633 = Or(x=w1306, y=w1305) -> (x .or. y?=w1304:bool)
            }
            n634 = call <vilib>:"Check if File or Folder Exists.vi"("error in (no error)"=w1250, "path"=w1251) -> ("file or folder exists?"=w1248:bool, "dup path"=w1249:path)  [unwired: 7 in, 1 out]
            n635 = case shown="True" w1248 {
              tunnel: w1249 -> [_ w1299]
              frame False {
              }
              frame True {
                n636 = Read from Text File(file (use dialog)=w1299) -> (text=w1303:string)  [unwired: 3 in, 3 out]
                n637 = property on="Image Out" class="ImageControl"() -> ("ROI"=w1300:T12)  [unwired: 2 in, 2 out]
                n638 = Unflatten From String(type=w1300, binary string=w1303) -> (value=w1301:T12, error out=w1302:errorcluster)  [unwired: 3 in, 1 out]
                n639 = property on="Image Out" class="ImageControl"(error in=w1302, "ROI"=w1301) -> ()  [unwired: 1 in, 2 out]
              }
            }
            n640 = invoke on="Image Out" class="ImageControl" method="Clear ROI"() -> ()  [unwired: 3 in, 3 out]
            n641 = Path To String(path=w1243) -> (string=w1277:string)
            n642 = Index Array(array=w1279, index=w1278) -> (element=w1255:string)
            n643 = Concatenate Strings(w1277, "\\", w1255) -> (w1276:string)
            n644 = local write "Image Name"(w1255) -> ()
            n645 = String To Path(string=w1276) -> (path=w1254:path)
            n646 = Empty String/Path?(string/path=w1255) -> (empty?=w1256:bool)
            n647 = local read "No Image File"() -> (w1252:path)
            n648 = Select(t=w1252, s=w1256, f=w1254) -> (s? t:f=w1253:path)
            n649 = local write "Image File"(w1253) -> ()
            n650 = call "Vision Acquisition3"("Image Path"=w1253) -> ("Image Out"=w1280:T2)  [unwired: 25 in, 1 out]
            n651 = local write "Image Out"(w1280) -> ()
            n652 = local write "Image Out 2"(w1280) -> ()
          }
          event "Up Button": Mouse Down {
            w1536 = 0
            n653 = event-data() -> ()  [unwired: 1 in, 5 out]
            n654 = local read "Transfer File"() -> (w1532:path)
            n655 = Strip Path(path=w1532) -> (stripped path=w1531:path, name=w1547:string)
            n656 = local write "Transfer Folder"(w1531) -> ()
            n657 = List Folder(path=w1531) -> (filenames=w1541:string[], error out=w1498:errorcluster)  [unwired: 3 in, 2 out]
            n658 = Array Size(array=w1541) -> (size(s)=w1486:i32)
            n659 = Search 1D Array(1D array=w1541, element=w1547) -> (index of element=w1542:i32)  [unwired: 1 in]
            n660 = Equal To 0?(x=w1542) -> (x = 0?=w1543:bool)
            n661 = local read "Folder Index"() -> (w1485:dbl)
            n662 = property on="Image Out" class="ImageControl"() -> (error out=w1488:errorcluster, "Image Center Position"=w1492:cluster{"X":u32, "Y":u32})  [unwired: 2 in, 1 out]
            n663 = case shown="True" w1543 {
              tunnel: w1485 -> [w1677 _]
              tunnel: [w1676 w1678] -> w1484
              tunnel: w1486 -> [_ w1679]
              frame False {
                n664 = Decrement(x=w1677) -> (x-1=w1676:dbl)
              }
              frame True {
                n665 = Decrement(x=w1679) -> (x-1=w1678:i32)
              }
            }
            n666 = Unbundle(w1492) -> ("X"=w1490:u32)  [unwired: 1 out]
            n667 = local write "Folder Index"(w1484) -> ()
            n668 = Bundle("X"=w1490, 0) -> (w1491:cluster{"X":u32, i32})  [unwired: 1 in]
            n669 = Path To String(path=w1531) -> (string=w1548:string)
            n670 = Index Array(array=w1541, index=w1484) -> (element=w1544:string)
            n671 = local write "Data Name:"(w1544) -> ()
            n672 = property on="Image Out" class="ImageControl"(error in=w1488, "Image Center Position"=w1491) -> ()  [unwired: 1 in, 2 out]
            n673 = Concatenate Strings(w1548, "\\", w1544) -> (w1546:string)
            n674 = String To Path(string=w1546) -> (path=w1436:path)
            n675 = call "Recorded Values.vi"("Path"=w1436) -> ("Recorded Char"=w1482:T6, "Recorded Prop"=w1481:T7, "Fabrication Prop"=w1483:T8)  [unwired: 8 in]
            n676 = Unbundle By Name(w1482) -> ("Mobility-Sat"=w1469:dbl, "Moblitity-Lin"=w1468:dbl, "On/Off"=w1467:dbl, "Off Current"=w1466:dbl, "Vt-Sat"=w1432:dbl, "STS"=w1465:dbl, "Trap Density-VT"=w1464:dbl, "Trap Density-STS"=w1463:dbl)
            n677 = Unbundle By Name(w1483) -> ("Date Created"=w1462:string, "Material"=w1480:string, "Solvent"=w1479:string, "Concentration"=w1478:dbl, "Method"=w1477:string, "Dielectric (nm)"=w1476:dbl, "Treatment"=w1475:string, "Comments"=w1474:string)
            n678 = Unbundle By Name(w1481) -> ("Date Recorded"=w1473:string, "Index"=w1472:string, "Length"=w1471:dbl, "Width"=w1470:dbl, "Sample Temp"=w1433:dbl)
            n679 = local write "Date Created"(w1462) -> ()
            n680 = local write "Rec: Material"(w1480) -> ()
            n681 = local write "Rec: Off I-Sat"(w1466) -> ()
            n682 = local write "Rec: Comments"(w1474) -> ()
            n683 = local write "Rec: VT-Sat"(w1432) -> ()
            n684 = local write "Rec: Solvent"(w1479) -> ()
            n685 = local write "Rec: Concentration"(w1478) -> ()
            n686 = local write "Rec: Method"(w1477) -> ()
            n687 = local write "Rec: Dielectric (d)"(w1476) -> ()
            n688 = local write "Surface Treatment:"(w1475) -> ()
            n689 = local write "Index"(w1472) -> ()
            n690 = local write "Rec: Mobility-Sat"(w1469) -> ()
            n691 = local write "Rec: Mobility-Lin"(w1468) -> ()
            n692 = local write "Rec: On/Off"(w1467) -> ()
            n693 = local write "Rec: STS"(w1465) -> ()
            n694 = local write "Rec: Trap Density-VT"(w1464) -> ()
            n695 = local write "Rec: Trap Density-STS"(w1463) -> ()
            n696 = local write "Date Recorded"(w1473) -> ()
            n697 = local write "Rec: Length"(w1471) -> ()
            n698 = local write "Rec: Width"(w1470) -> ()
            n699 = local write "Rec: Temp"(w1433) -> ()
            n700 = Equal To 0?(x=w1433) -> (x = 0?=w1435:bool)
            n701 = case shown="False" w1435 {
              tunnel: [w1549 w1550] -> w1434
              tunnel: w1433 -> [w1549 _]
              frame False {
              }
              frame True {
                n702 = local read "Room Temp"() -> (w1550:dbl)
              }
            }
            n703 = local read "NumPoints Log"() -> (w1458:dbl)
            n704 = local write "Transfer File"(w1436) -> ()
            n705 = local read "Num Pts"() -> (w1461:dbl)
            n706 = local read "New: Dielectric"() -> (w1442:dbl)
            n707 = call "Mobility-Vt Calculator-File.vi"("NumPts"=w1461, "Path"=w1436) -> ("Graph Cluster"=w1430:T9, "Output"=w1460:T10, "Index-Sat"=w1459:dbl, "Index-Lin"=w1446:dbl)  [unwired: 5 in, 1 out]
            n708 = call "STS Calculator-File.vi"("NumPts"=w1458, "Path"=w1436) -> ("STS Index-Sat"=w1457:dbl, "XY Graph-Sat"=w1456:cluster{dbl[], dbl[]}[], "Ouput"=w1455:cluster{"STS-Sat":dbl, "STS-Lin":dbl})  [unwired: 5 in, 2 out]
            n709 = call-poly <vilib>:"Read From Spreadsheet File.vi"("file path (dialog if empty)"=w1436) -> ("all rows"=w1538:string[][])  [unwired: 6 in, 4 out]
            n710 = Unbundle By Name(w1460) -> ("Mobility-Sat"=w1445:dbl, "Vt-Sat"=w1438:dbl, "Mobility-Lin"=w1444:dbl, "Vt-Lin"=w1443:dbl, "Off I-Sat"=w1437:dbl, "On/Off I-Sat"=w1431:dbl)
            n711 = local write "Sat-Trans Slider"(w1459) -> ()
            n712 = Unbundle By Name(w1455) -> ("STS-Sat"=w1439:dbl)  [unwired: 1 out]
            n713 = local write "Index 2"(w1457) -> ()
            n714 = local write "MobVi Index"(w1459) -> ()
            n715 = local write "Log-Sat"(w1456) -> ()
            n716 = local write "Calc: Mobility-Sat"(w1445) -> ()
            n717 = local write "Calc: VT-Sat"(w1438) -> ()
            n718 = local write "Calc: Mobility-Lin"(w1444) -> ()
            n719 = local write "Calc: Off I-Sat"(w1437) -> ()
            n720 = local write "Calc: On/Off"(w1431) -> ()
            n721 = Array Size(array=w1538) -> (size(s)=w1537:i32[])
            n722 = local write "Calc: VT-Lin"(w1443) -> ()
            n723 = call "Trap Density_VT.vi"("VT"=w1438, "Dielectric"=w1442) -> ("Trap Density-VT"=w1441:dbl)
            n724 = call "Trap Density_STS.vi"("Temp (T) [K]"=w1434, "S.T.S. (S)"=w1439, "Dielectric"=w1442) -> ("Trap Density (N)"=w1440:dbl)  [unwired: 8 in]
            n725 = Unbundle By Name(w1430) -> ("Raw Sat"=w1427:cluster{dbl[], dbl[]}[], "Sqrt Sat"=w1428:cluster{dbl[], dbl[]}[], "Log Sat"=w1426:cluster{dbl[], dbl[]}[], "Raw Lin"=w1425:cluster{dbl[], dbl[]}[], "Sqrt Lin"=w1429:cluster{dbl[], dbl[]}[], "Log Lin"=w1424:cluster{dbl[], dbl[]}[])
            n726 = local write "Sqrt-Sat"(w1428) -> ()
            n727 = local write "Calc: STS"(w1439) -> ()
            n728 = local write "New: STS"(w1439) -> ()
            n729 = Decimate 1D Array(w1429) -> (w1454:cluster{dbl[], dbl[]}[])  [unwired: 1 out]
            n730 = local write "Calc: Trap Density-VT"(w1441) -> ()
            n731 = local write "New: VT-Sat"(w1438) -> ()
            n732 = local write "Calc: Trap Density-STS"(w1440) -> ()
            n733 = local write "New: Trap Density-STS"(w1440) -> ()
            n734 = local write "New: Trap Density-VT"(w1441) -> ()
            n735 = local write "New: VT-Lin"(w1443) -> ()
            n736 = local write "Sqrt-Lin"(w1429) -> ()
            n737 = local write "New: Mobility-Sat"(w1445) -> ()
            n738 = local write "New: Mobility-Lin"(w1444) -> ()
            n739 = Decimate 1D Array(w1456) -> (w1515:cluster{dbl[], dbl[]}[])  [unwired: 1 out]
            n740 = Index Array(array=w1537, index=w1536) -> (element=w1521:i32)
            n741 = Decimate 1D Array(w1428) -> (w1525:cluster{dbl[], dbl[]}[])  [unwired: 1 out]
            n742 = Array To Cluster(array=w1454) -> (cluster=w1453:T11)
            n743 = Array Subset(array=w1538, index (row)=w1536, index (col)=w1536, length (col)=3) -> (w1539:string[][])  [unwired: 1 in]
            n744 = local write "Raw- Sat"(w1427) -> ()
            n745 = local write "Raw- Lin"(w1425) -> ()
            n746 = local write "Log-Sat"(w1426) -> ()
            n747 = local write "Log-Lin"(w1424) -> ()
            n748 = Array To Cluster(array=w1515) -> (cluster=w1513:T11)
            n749 = Array To Cluster(array=w1525) -> (cluster=w1527:T11)
            n750 = Reshape Array(w1539, w1521) -> (w1528:string[])
            n751 = Subtract(x=w1521, y=20) -> (x-y=w1520:i32)
            n752 = Unbundle(w1453) -> ("[0]"=w1450:cluster{dbl[], dbl[]})  [unwired: 8 out]
            n753 = property on="Sat-Trans Slider" class="Slide (strict)"("Scale.Maximum"=w1520) -> ()  [unwired: 2 in, 2 out]
            n754 = local read "Num Pts"() -> (w1447:dbl)
            n755 = Unbundle(w1513) -> ("[0]"=w1514:cluster{dbl[], dbl[]})  [unwired: 8 out]
            n756 = Unbundle(w1527) -> ("[0]"=w1526:cluster{dbl[], dbl[]})  [unwired: 8 out]
            n757 = Unbundle(w1450) -> (w1449:dbl[], w1448:dbl[])
            n758 = Search 1D Array(1D array=w1528, element="Index:") -> (index of element=w1533:i32)  [unwired: 1 in]
            n759 = Increment(x=w1533) -> (x+1=w1534:i32)
            n760 = Unbundle(w1514) -> (w1512:dbl[], w1511:dbl[])
            n761 = Unbundle(w1526) -> (w1519:dbl[], w1518:dbl[])
            n762 = Array Subset(array=w1449, index=w1446, length=w1447) -> (w1451:dbl[])
            n763 = Array Subset(array=w1448, index=w1446, length=w1447) -> (w1452:dbl[])
            n764 = local read "Image Folder"() -> (w1487:path)
            n765 = local write "Lin-Vg Array-Used"(w1451) -> ()
            n766 = Array Subset(array=w1512, index=w1457, length=w1458) -> (w1517:dbl[])
            n767 = Array Subset(array=w1511, index=w1457, length=w1458) -> (w1516:dbl[])
            n768 = Array Subset(array=w1519, index=w1459, length=w1461) -> (w1524:dbl[])
            n769 = Array Subset(array=w1518, index=w1459, length=w1461) -> (w1523:dbl[])
            n770 = local write "Lin Id-Used"(w1452) -> ()
            n771 = Index Array(array=w1528, index=w1534) -> (element=w1494:string)
            n772 = local write "Sat Vg Array-Used"(w1524) -> ()
            n773 = local write "Vg Array-Log-Used"(w1516) -> ()
            n774 = local write "Sat Id-Log-Used"(w1517) -> ()
            n775 = local write "Sat Id-Used"(w1523) -> ()
            n776 = local write "Index"(w1494) -> ()
            n777 = List Folder(path=w1487, error in=w1498) -> (filenames=w1530:string[], error out=w1497:errorcluster)  [unwired: 2 in, 2 out]
            n778 = Build Path(base path=w1487, name or relative path="ROI") -> (appended path=w1495:path)
            n779 = invoke on="Image Out" class="ImageControl" method="Clear ROI"(error in=w1497) -> (error out=w1501:errorcluster)  [unwired: 2 in, 2 out]
            n780 = while {
              tunnel: w1530 -> [w1563]
              tunnel: w1494 -> [w1561]
              tunnel: [w1560] -> w1529
              tunnel: w1521 -> [w1559]
              i -> [w1560]
              stop <- w1556 stop-if-true
              n781 = Index Array(array=w1563, index=w1560) -> (element=w1564:string)
              n782 = xnode "Match Regular Expression"("input string"=w1564, "regular expression"=w1561) -> ("whole match"=w1562:string)  [unwired: 4 in, 4 out]
              n783 = Equal?(x=w1562, y=w1561) -> (x = y?=w1558:bool)
              n784 = Equal?(x=w1559, y=w1560) -> (x = y?=w1557:bool)
              n785 = Or(x=w1558, y=w1557) -> (x .or. y?=w1556:bool)
            }
            n786 = Build Path(base path=w1495, name or relative path=w1494) -> (appended path=w1493:path)
            n787 = call <vilib>:"Check if File or Folder Exists.vi"("error in (no error)"=w1501, "path"=w1493) -> ("file or folder exists?"=w1499:bool, "dup path"=w1500:path)  [unwired: 7 in, 1 out]
            n788 = case shown="True" w1499 {
              tunnel: w1500 -> [_ w1551]
              frame False {
              }
              frame True {
                n789 = Read from Text File(file (use dialog)=w1551) -> (text=w1555:string)  [unwired: 3 in, 3 out]
                n790 = property on="Image Out" class="ImageControl"() -> ("ROI"=w1552:T12)  [unwired: 2 in, 2 out]
                n791 = Unflatten From String(type=w1552, binary string=w1555) -> (value=w1553:T12, error out=w1554:errorcluster)  [unwired: 3 in, 1 out]
                n792 = property on="Image Out" class="ImageControl"(error in=w1554, "ROI"=w1553) -> ()  [unwired: 1 in, 2 out]
              }
            }
            n793 = Index Array(array=w1530, index=w1529) -> (element=w1503:string)
            n794 = local write "Image Name"(w1503) -> ()
            n795 = Empty String/Path?(string/path=w1503) -> (empty?=w1510:bool)
            n796 = Build Path(base path=w1487, name or relative path=w1503) -> (appended path=w1502:path)
            n797 = local read "No Image File"() -> (w1509:path)
            n798 = Select(t=w1509, s=w1510, f=w1502) -> (s? t:f=w1504:path)
            n799 = call <vilib>:"Get File Extension.vi"("file"=w1504) -> ("lowercase file extension"=w1506:string)  [unwired: 7 in, 3 out]
            n800 = local write "Image File"(w1504) -> ()
            n801 = local write "String"(w1506) -> ()
            n802 = Search 1D Array(1D array=string[] ["bmp", "jpeg", "png", "jpg", "gif"], element=w1506) -> (index of element=w1505:i32)  [unwired: 1 in]
            n803 = call "Vision Acquisition5"("Image Path"=w1504) -> ("Image Out"=w1508:T2)  [unwired: 25 in, 1 out]
            n804 = Less Than 0?(x=w1505) -> ()  [unwired: 1 out]
            n805 = local write "Image Out"(w1508) -> ()
            n806 = local write "Image Out 2"(w1508) -> ()
          }
          event "Save Changes? 3": Mouse Down {
            n807 = event-data() -> ()  [unwired: 1 in, 7 out]
            n808 = local read "Image Folder"() -> (w1680:path)
            n809 = Build Path(base path=w1680, name or relative path="ROI") -> (appended path=w1687:path)
            n810 = call <vilib>:"Check if File or Folder Exists.vi"("path"=w1687) -> ("file or folder exists?"=w1689:bool, "dup path"=w1686:path)  [unwired: 8 in, 1 out]
            n811 = case shown="False" w1689 {
              tunnel: w1686 -> [w1691 w1692]
              tunnel: [w1690 w1692] -> w1681
              frame False {
                n812 = Create Folder(path (use dialog)=w1691) -> (created path=w1690:path)  [unwired: 2 in, 2 out]
              }
              frame True {
              }
            }
            n813 = local read "Index"() -> (w1683:string)
            n814 = property on="Image Out" class="ImageControl"() -> ("ROI"=w1685:T12)  [unwired: 2 in, 2 out]
            n815 = Build Path(base path=w1681, name or relative path=w1683) -> (appended path=w1682:path)
            n816 = Flatten To String(anything=w1685) -> (data string=w1684:string)  [unwired: 3 in, 2 out]
            n817 = Write to Text File(file (use dialog)=w1682, text=w1684) -> ()  [unwired: 2 in, 3 out]
          }
          event "Next Sqrt Sat": Mouse Down {
            n818 = event-data() -> ()  [unwired: 1 in, 5 out]
            n819 = local read "Sqrt-Sat"() -> (w1705:cluster{dbl[], dbl[]}[])
            n820 = Decimate 1D Array(w1705) -> (w1701:cluster{dbl[], dbl[]}[], w1700:cluster{dbl[], dbl[]}[])
            n821 = Array To Cluster(array=w1701) -> (cluster=w1711:T11)
            n822 = local read "MobVi Index"() -> (w1707:dbl)
            n823 = Unbundle(w1711) -> ("[0]"=w1710:cluster{dbl[], dbl[]})  [unwired: 8 out]
            n824 = local read "Num Pts"() -> (w1706:dbl)
            n825 = Unbundle(w1710) -> (w1709:dbl[], w1708:dbl[])
            n826 = Increment(x=w1707) -> (x+1=w1702:dbl)
            n827 = local read "New: Dielectric"() -> (w1696:dbl)
            n828 = local read "New: Length"() -> (w1695:dbl)
            n829 = local read "New: Width"() -> (w1694:dbl)
            n830 = local write "MobVi Index"(w1702) -> ()
            n831 = Array Subset(array=w1709, index=w1702, length=w1706) -> (w1698:dbl[])
            n832 = Array Subset(array=w1708, index=w1702, length=w1706) -> (w1697:dbl[])
            n833 = local write "Sat Vg Array-Used"(w1698) -> ()
            n834 = local write "Sat Id-Used"(w1697) -> ()
            n835 = call "Mobility-Vt-Used Pts_Saturation.vi"("Width"=w1694, "Length"=w1695, "Dielectric (d)"=w1696, "Sat Id Used"=w1697, "Vg Used"=w1698) -> ("Vt"=w1693:dbl, "Mobility"=w1699:dbl)  [unwired: 4 in, 1 out]
            n836 = Bundle(w1698, w1697) -> (w1704:cluster{dbl[], dbl[]})  [unwired: 1 in]
            n837 = Build Array (concatenate)(w1701, w1700, w1704) -> (w1703:cluster{dbl[], dbl[]}[])
            n838 = local write "New: Mobility-Sat"(w1699) -> ()
            n839 = local write "New: VT-Sat"(w1693) -> ()
            n840 = local write "Sqrt-Sat"(w1703) -> ()
          }
          event "Next Log Sat": Mouse Down {
            n841 = event-data() -> ()  [unwired: 1 in, 7 out]
            n842 = local read "Log-Sat"() -> (w1720:cluster{dbl[], dbl[]}[])
            n843 = Decimate 1D Array(w1720) -> (w1716:cluster{dbl[], dbl[]}[], w1715:cluster{dbl[], dbl[]}[])
            n844 = Array To Cluster(array=w1716) -> (cluster=w1726:T11)
            n845 = local read "Index 2"() -> (w1722:dbl)
            n846 = local read "NumPoints Log"() -> (w1721:dbl)
            n847 = Unbundle(w1726) -> ("[0]"=w1725:cluster{dbl[], dbl[]})  [unwired: 8 out]
            n848 = Unbundle(w1725) -> (w1724:dbl[], w1723:dbl[])
            n849 = Increment(x=w1722) -> (x+1=w1717:dbl)
            n850 = local write "Index 2"(w1717) -> ()
            n851 = Array Subset(array=w1723, index=w1717, length=w1721) -> (w1712:dbl[])
            n852 = Array Subset(array=w1724, index=w1717, length=w1721) -> (w1713:dbl[])
            n853 = call "STS-Used.vi"("Id Used"=w1713, "Vg-Used"=w1712) -> ("STS"=w1714:dbl)  [unwired: 9 in]
            n854 = Bundle(w1713, w1712) -> (w1719:cluster{dbl[], dbl[]})  [unwired: 1 in]
            n855 = local write "Vg Array-Log-Used"(w1712) -> ()
            n856 = local write "Sat Id-Log-Used"(w1713) -> ()
            n857 = local write "New: STS"(w1714) -> ()
            n858 = Build Array (concatenate)(w1716, w1715, w1719) -> (w1718:cluster{dbl[], dbl[]}[])
            n859 = local write "Log-Sat"(w1718) -> ()
          }
          event "Previous Log Sat": Mouse Down {
            n860 = event-data() -> ()  [unwired: 1 in, 7 out]
            n861 = local read "Log-Sat"() -> (w1736:cluster{dbl[], dbl[]}[])
            n862 = Decimate 1D Array(w1736) -> (w1733:cluster{dbl[], dbl[]}[], w1732:cluster{dbl[], dbl[]}[])
            n863 = Array To Cluster(array=w1733) -> (cluster=w1741:T11)
            n864 = local read "Index 2"() -> (w1729:dbl)
            n865 = local read "NumPoints Log"() -> (w1737:dbl)
            n866 = Unbundle(w1741) -> ("[0]"=w1740:cluster{dbl[], dbl[]})  [unwired: 8 out]
            n867 = Unbundle(w1740) -> (w1739:dbl[], w1738:dbl[])
            n868 = Decrement(x=w1729) -> (x-1=w1730:dbl)
            n869 = local write "Index 2"(w1730) -> ()
            n870 = Array Subset(array=w1739, index=w1730, length=w1737) -> (w1727:dbl[])
            n871 = Array Subset(array=w1738, index=w1730, length=w1737) -> (w1728:dbl[])
            n872 = local write "Vg Array-Log-Used"(w1728) -> ()
            n873 = local write "Sat Id-Log-Used"(w1727) -> ()
            n874 = Bundle(w1727, w1728) -> (w1735:cluster{dbl[], dbl[]})  [unwired: 1 in]
            n875 = call "STS-Used.vi"("Id Used"=w1727, "Vg-Used"=w1728) -> ("STS"=w1731:dbl)  [unwired: 9 in]
            n876 = Build Array (concatenate)(w1733, w1732, w1735) -> (w1734:cluster{dbl[], dbl[]}[])
            n877 = local write "New: STS"(w1731) -> ()
            n878 = local write "Log-Sat"(w1734) -> ()
          }
          event "Previous Sqrt Sat": Mouse Down {
            n879 = event-data() -> ()  [unwired: 1 in, 5 out]
            n880 = local read "Sqrt-Sat"() -> (w1755:cluster{dbl[], dbl[]}[])
            n881 = Decimate 1D Array(w1755) -> (w1752:cluster{dbl[], dbl[]}[], w1751:cluster{dbl[], dbl[]}[])
            n882 = Array To Cluster(array=w1752) -> (cluster=w1760:T11)
            n883 = local read "MobVi Index"() -> (w1750:dbl)
            n884 = Unbundle(w1760) -> ("[0]"=w1759:cluster{dbl[], dbl[]})  [unwired: 8 out]
            n885 = local read "Num Pts"() -> (w1756:dbl)
            n886 = Unbundle(w1759) -> (w1758:dbl[], w1757:dbl[])
            n887 = Decrement(x=w1750) -> (x-1=w1749:dbl)
            n888 = local read "New: Dielectric"() -> (w1743:dbl)
            n889 = local read "New: Length"() -> (w1744:dbl)
            n890 = local read "New: Width"() -> (w1745:dbl)
            n891 = local write "MobVi Index"(w1749) -> ()
            n892 = Array Subset(array=w1758, index=w1749, length=w1756) -> (w1748:dbl[])
            n893 = Array Subset(array=w1757, index=w1749, length=w1756) -> (w1747:dbl[])
            n894 = local write "Sat Vg Array-Used"(w1748) -> ()
            n895 = local write "Sat Id-Used"(w1747) -> ()
            n896 = call "Mobility-Vt-Used Pts_Linear.vi"("Width"=w1745, "Length"=w1744, "Dielectric (d)"=w1743, "Sat Id Used"=w1747, "Vg Used"=w1748) -> ("Vt"=w1742:dbl, "Mobility"=w1746:dbl)  [unwired: 4 in, 1 out]
            n897 = Bundle(w1748, w1747) -> (w1754:cluster{dbl[], dbl[]})  [unwired: 1 in]
            n898 = local write "New: VT-Sat"(w1742) -> ()
            n899 = Build Array (concatenate)(w1752, w1751, w1754) -> (w1753:cluster{dbl[], dbl[]}[])
            n900 = local write "New: Mobility-Sat"(w1746) -> ()
            n901 = local write "Sqrt-Sat"(w1753) -> ()
          }
          event "Sat-Trans Slider": Value Change {
            n902 = event-data() -> ()  [unwired: 1 in, 5 out]
            n903 = local read "Sqrt-Sat"() -> (w1773:cluster{dbl[], dbl[]}[])
            n904 = Decimate 1D Array(w1773) -> (w1770:cluster{dbl[], dbl[]}[], w1769:cluster{dbl[], dbl[]}[])
            n905 = Array To Cluster(array=w1770) -> (cluster=w1778:T11)
            n906 = Unbundle(w1778) -> ("[0]"=w1777:cluster{dbl[], dbl[]})  [unwired: 8 out]
            n907 = local read "Sat-Trans Slider"() -> (w1762:dbl)
            n908 = local read "Num Pts"() -> (w1774:dbl)
            n909 = Unbundle(w1777) -> (w1776:dbl[], w1775:dbl[])
            n910 = local read "New: Dielectric"() -> (w1763:dbl)
            n911 = local read "New: Length"() -> (w1764:dbl)
            n912 = local read "New: Width"() -> (w1765:dbl)
            n913 = local write "MobVi Index"(w1762) -> ()
            n914 = Array Subset(array=w1776, index=w1762, length=w1774) -> (w1768:dbl[])
            n915 = Array Subset(array=w1775, index=w1762, length=w1774) -> (w1767:dbl[])
            n916 = local write "Sat Vg Array-Used"(w1768) -> ()
            n917 = local write "Sat Id-Used"(w1767) -> ()
            n918 = call "Mobility-Vt-Used Pts_Linear.vi"("Width"=w1765, "Length"=w1764, "Dielectric (d)"=w1763, "Sat Id Used"=w1767, "Vg Used"=w1768) -> ("Vt"=w1761:dbl, "Mobility"=w1766:dbl)  [unwired: 4 in, 1 out]
            n919 = Bundle(w1768, w1767) -> (w1772:cluster{dbl[], dbl[]})  [unwired: 1 in]
            n920 = local write "New: VT-Sat"(w1761) -> ()
            n921 = Build Array (concatenate)(w1770, w1769, w1772) -> (w1771:cluster{dbl[], dbl[]}[])
            n922 = local write "New: Mobility-Sat"(w1766) -> ()
            n923 = local write "Sqrt-Sat"(w1771) -> ()
          }
          event "Sat-Log Slider": Value Change {
            n924 = event-data() -> ()  [unwired: 1 in, 5 out]
            n925 = local read "Log-Sat"() -> (w1787:cluster{dbl[], dbl[]}[])
            n926 = Decimate 1D Array(w1787) -> (w1784:cluster{dbl[], dbl[]}[], w1783:cluster{dbl[], dbl[]}[])
            n927 = Array To Cluster(array=w1784) -> (cluster=w1792:T11)
            n928 = Unbundle(w1792) -> ("[0]"=w1791:cluster{dbl[], dbl[]})  [unwired: 8 out]
            n929 = local read "NumPoints Log"() -> (w1788:dbl)
            n930 = local read "Sat-Log Slider"() -> (w1782:dbl)
            n931 = Unbundle(w1791) -> (w1790:dbl[], w1789:dbl[])
            n932 = local write "Index 2"(w1782) -> ()
            n933 = Array Subset(array=w1790, index=w1782, length=w1788) -> (w1780:dbl[])
            n934 = Array Subset(array=w1789, index=w1782, length=w1788) -> (w1779:dbl[])
            n935 = local write "Vg Array-Log-Used"(w1779) -> ()
            n936 = local write "Sat Id-Log-Used"(w1780) -> ()
            n937 = call "STS-Used.vi"("Id Used"=w1780, "Vg-Used"=w1779) -> ("STS"=w1781:dbl)  [unwired: 9 in]
            n938 = Bundle(w1780, w1779) -> (w1786:cluster{dbl[], dbl[]})  [unwired: 1 in]
            n939 = local write "New: STS"(w1781) -> ()
            n940 = Build Array (concatenate)(w1784, w1783, w1786) -> (w1785:cluster{dbl[], dbl[]}[])
            n941 = local write "Log-Sat"(w1785) -> ()
          }
          event "Save Changes?": Mouse Down {
            n942 = event-data() -> ()  [unwired: 1 in, 5 out]
            n943 = flat-sequence {
              tunnel: [w1799] -> w1797
              tunnel: [w1807] -> w1796
              tunnel: [w1800] -> w1795
              tunnel: w1797 -> [w2339]
              tunnel: w1796 -> [w2336]
              tunnel: [w2337] -> w1794
              tunnel: w1795 -> [w2337]
              tunnel: [w2336] -> w1793
              tunnel: w1794 -> [w2344]
              tunnel: w1793 -> [w2343]
              frame #0 {
                n944 = Wait (ms)(milliseconds to wait=1) -> ()  [unwired: 1 out]
              }
              frame #1 {
                n945 = local read "Transfer File"() -> (w1799:path)
                n946 = local read "New: Temp"() -> (w1801:dbl)
                n947 = local read "New: Length"() -> (w1805:dbl)
                n948 = local read "New: Width"() -> (w1803:dbl)
                n949 = To Single Precision Float(number=w1801) -> (single precision float=w1802:sgl)
                n950 = Number To Decimal String(number=w1802) -> (decimal integer string=w1810:string)  [unwired: 1 in]
                n951 = To Single Precision Float(number=w1803) -> (single precision float=w1804:sgl)
                n952 = To Single Precision Float(number=w1805) -> (single precision float=w1806:sgl)
                n953 = local read "Index"() -> (w1815:string)
                n954 = Strip Path(path=w1799) -> (stripped path=w1820:path)  [unwired: 1 out]
                n955 = Number To Decimal String(number=w1806) -> (decimal integer string=w1813:string)  [unwired: 1 in]
                n956 = Number To Decimal String(number=w1804) -> (decimal integer string=w1814:string)  [unwired: 1 in]
                n957 = Concatenate Strings("_", w1810, "K") -> (w1808:string)
                n958 = call "Build Text"("Temp"=w1808, "Index"=w1815, "Length"=w1813, "Width"=w1814) -> ("Result"=w1816:string)  [unwired: 10 in, 1 out]
                n959 = flat-sequence {
                  tunnel: [w2293] -> w1812
                  tunnel: w1812 -> [w2310]
                  frame #0 {
                    # "Makes Empty File for Transformer Data"
                    n960 = local read "Transfer Folder"() -> (w2282:path)
                    n961 = Build Path(base path=w2282, name or relative path="Stats") -> (appended path=w2284:path)
                    n962 = call <vilib>:"Check if File or Folder Exists.vi"("path"=w2284) -> ("file or folder exists?"=w2285:bool, "dup path"=w2286:path)  [unwired: 8 in, 1 out]
                    n963 = case shown="False" w2285 {
                      tunnel: [w2290 w2292] -> w2287
                      tunnel: w2286 -> [w2291 w2292]
                      frame False {
                        n964 = Create Folder(path (use dialog)=w2291) -> (created path=w2290:path)  [unwired: 2 in, 2 out]
                      }
                      frame True {
                      }
                    }
                    n965 = Build Path(base path=w2287, name or relative path="Tranformer Data.txt") -> (appended path=w2289:path)
                    n966 = call-poly <vilib>:"Write To Spreadsheet File.vi"("append to file? (new file:F)"=TRUE, "file path (dialog if empty)"=w2289) -> ()  [unwired: 6 in, 1 out]
                  }
                  frame #1 {
                    # "Adds Headers if they don't exist"
                    n967 = local read "Transfer Folder"() -> (w2299:path)
                    n968 = Concatenate Strings("Stats\\", "Tranformer Data.txt") -> (w2300:string)
                    n969 = Build Path(base path=w2299, name or relative path=w2300) -> (appended path=w2293:path)
                    n970 = call-poly <vilib>:"Read From Spreadsheet File.vi"("file path (dialog if empty)"=w2293) -> ("first row"=w2298:string[])  [unwired: 6 in, 4 out]
                    n971 = Search 1D Array(1D array=w2298, element="DeviceID") -> (index of element=w2296:i32)  [unwired: 1 in]
                    n972 = Equal?(x=w2296, y=0) -> (x = y?=w2294:bool)
                    n973 = case shown="False" w2294 {
                      tunnel: w2293 -> [w2304 _]
                      frame False {
                        n974 = local read "Transformer \nHeaders"() -> (w2303:string[])
                        n975 = call-poly <vilib>:"Write To Spreadsheet File.vi"("1D data"=w2303, "file path (dialog if empty)"=w2304) -> ()  [unwired: 6 in, 1 out]
                      }
                      frame True {
                      }
                    }
                  }
                  frame #2 {
                    # "Adds current device if it doesn't exist"
                    n976 = local read "Current \nRecord"() -> (w2309:string[])
                    n977 = Index Array(array=w2309, index=0) -> (element=w2308:string)
                    n978 = local read "Transfer Folder"() -> (w2312:path)
                    n979 = Concatenate Strings("Stats\\", "Tranformer Data.txt") -> (w2313:string)
                    n980 = local write "Current Device ID"(w2308) -> ()
                    n981 = local read "Current Device ID"() -> (w2318:string)
                    n982 = Build Path(base path=w2312, name or relative path=w2313) -> (appended path=w2311:path)
                    n983 = call-poly <vilib>:"Read From Spreadsheet File.vi"("file path (dialog if empty)"=w2311) -> ("all rows"=w2305:string[][])  [unwired: 6 in, 4 out]
                    n984 = Index Array(array=w2305, index (col)=0) -> (element=w2306:string[])  [unwired: 1 in]
                    n985 = Search 1D Array(1D array=w2306, element=w2318) -> (index of element=w2307:i32)  [unwired: 1 in]
                    n986 = Equal?(x=w2307, y=-1) -> (x = y?=w2320:bool)
                    n987 = case shown="False" w2320 {
                      tunnel: w2310 -> [w2323 w2334]
                      tunnel: w2307 -> [w2326 _]
                      tunnel: w2305 -> [w2327 _]
                      frame False {
                        n988 = local read "Current \nRecord"() -> (w2325:string[])
                        n989 = Replace Array Subset(array=w2327, new element=w2325, index (row)=w2326) -> (w2324:string[][])  [unwired: 1 in]
                        n990 = flat-sequence {
                          tunnel: w2323 -> [w2328]
                          tunnel: w2324 -> [w2329]
                          tunnel: [w2329] -> w2322
                          tunnel: [w2328] -> w2321
                          tunnel: w2322 -> [w2331]
                          tunnel: w2321 -> [w2330]
                          frame #0 {
                            n991 = Delete(path (use dialog)=w2328) -> ()  [unwired: 4 in, 3 out]
                          }
                          frame #1 {
                            n992 = call-poly <vilib>:"Write To Spreadsheet File.vi"("append to file? (new file:F)"=TRUE, "2D data"=w2331, "file path (dialog if empty)"=w2330) -> ()  [unwired: 5 in, 1 out]
                          }
                        }
                      }
                      frame True {
                        n993 = local read "Current \nRecord"() -> (w2333:string[])
                        n994 = call-poly <vilib>:"Write To Spreadsheet File.vi"("append to file? (new file:F)"=TRUE, "1D data"=w2333, "file path (dialog if empty)"=w2334) -> ()  [unwired: 5 in, 1 out]
                      }
                    }
                  }
                }
                n995 = Path To String(path=w1820) -> (string=w1818:string)
                n996 = stacked-sequence {
                  tunnel: [_ _ _ _ _ _ _ _ _ _ _ _ _ w2253] -> w1800
                  tunnel: w1799 -> [w1822 _ _ _ _ _ _ _ _ _ _ _ _ _]
                  frame #0 {
                    n997 = call-poly <vilib>:"Read From Spreadsheet File.vi"("file path (dialog if empty)"=w1822) -> ("all rows"=w1821:string[][])  [unwired: 6 in, 4 out]
                    n998 = Array Size(array=w1821) -> (size(s)=w1826:i32[])
                    n999 = Array Subset(array=w1821, index (row)=0, index (col)=0, length (col)=3) -> (w1830:string[][])  [unwired: 1 in]
                    n1000 = Index Array(array=w1826, index=0) -> (element=w1824:i32)
                    n1001 = Reshape Array(w1830, w1824) -> (w1823:string[])
                    n1002 = Search 1D Array(1D array=w1823, element="Dielectric (nm):") -> (index of element=w1833:i32)  [unwired: 1 in]
                    n1003 = Equal?(x=w1833, y=-1) -> (x = y?=w1832:bool)
                    n1004 = case shown="False" w1832 {
                      tunnel: w1821 -> [w1841 w1845]
                      tunnel: w1833 -> [w1837 _]
                      tunnel: [w1836 w1845] -> w1831
                      frame False {
                        n1005 = local read "New: Dielectric"() -> (w1843:dbl)
                        n1006 = Number To Fractional String(number=w1843) -> (F-format string=w1838:string)  [unwired: 3 in]
                        n1007 = Divide(x=w1837, y=3) -> (x/y=w1840:dbl)
                        n1008 = To Word Integer(number=w1840) -> (16bit integer=w1839:i16)
                        n1009 = Replace Array Subset(array=w1841, new element=w1838, index (row)=w1839, index (col)=1) -> (w1836:string[][])
                      }
                      frame True {
                      }
                    }
                    n1010 = local write "Save1 Array"(w1831) -> ()
                  }
                  frame #1 {
                    n1011 = local read "Save1 Array"() -> (w1847:string[][])
                    n1012 = Array Size(array=w1847) -> (size(s)=w1850:i32[])
                    n1013 = Array Subset(array=w1847, index (row)=0, index (col)=0, length (col)=3) -> (w1854:string[][])  [unwired: 1 in]
                    n1014 = Index Array(array=w1850, index=0) -> (element=w1848:i32)
                    n1015 = Reshape Array(w1854, w1848) -> (w1846:string[])
                    n1016 = Search 1D Array(1D array=w1846, element="Comments:") -> (index of element=w1857:i32)  [unwired: 1 in]
                    n1017 = Equal?(x=w1857, y=-1) -> (x = y?=w1856:bool)
                    n1018 = case shown="False" w1856 {
                      tunnel: w1847 -> [w1865 w1868]
                      tunnel: w1857 -> [w1862 _]
                      tunnel: [w1861 w1868] -> w1855
                      frame False {
                        n1019 = local read "Comments:"() -> (w1860:string)
                        n1020 = Divide(x=w1862, y=3) -> (x/y=w1864:dbl)
                        n1021 = To Word Integer(number=w1864) -> (16bit integer=w1863:i16)
                        n1022 = Replace Array Subset(array=w1865, new element=w1860, index (row)=w1863, index (col)=1) -> (w1861:string[][])
                      }
                      frame True {
                      }
                    }
                    n1023 = local write "Save1 Array"(w1855) -> ()
                  }
                  frame #2 {
                    n1024 = local read "Save1 Array"() -> (w1870:string[][])
                    n1025 = Array Size(array=w1870) -> (size(s)=w1873:i32[])
                    n1026 = Array Subset(array=w1870, index (row)=0, index (col)=0, length (col)=3) -> (w1877:string[][])  [unwired: 1 in]
                    n1027 = Index Array(array=w1873, index=0) -> (element=w1871:i32)
                    n1028 = Reshape Array(w1877, w1871) -> (w1869:string[])
                    n1029 = Search 1D Array(1D array=w1869, element="Length (um):") -> (index of element=w1880:i32)  [unwired: 1 in]
                    n1030 = Equal?(x=w1880, y=-1) -> (x = y?=w1879:bool)
                    n1031 = case shown="False" w1879 {
                      tunnel: w1870 -> [w1890 w1893]
                      tunnel: w1880 -> [w1887 _]
                      tunnel: [w1886 w1893] -> w1878
                      frame False {
                        n1032 = local read "New: Length"() -> (w1883:dbl)
                        n1033 = Divide(x=w1887, y=3) -> (x/y=w1889:dbl)
                        n1034 = Format Value(format string="%#g", value (0)=w1883) -> (output string=w1884:string)  [unwired: 1 in]
                        n1035 = To Word Integer(number=w1889) -> (16bit integer=w1888:i16)
                        n1036 = Replace Array Subset(array=w1890, new element=w1884, index (row)=w1888, index (col)=1) -> (w1886:string[][])
                      }
                      frame True {
                      }
                    }
                    n1037 = local write "Save1 Array"(w1878) -> ()
                  }
                  frame #3 {
                    n1038 = local read "Save1 Array"() -> (w1895:string[][])
                    n1039 = Array Size(array=w1895) -> (size(s)=w1900:i32[])
                    n1040 = Array Subset(array=w1895, index (row)=0, index (col)=0, length (col)=3) -> (w1896:string[][])  [unwired: 1 in]
                    n1041 = Index Array(array=w1900, index=0) -> (element=w1902:i32)
                    n1042 = Reshape Array(w1896, w1902) -> (w1894:string[])
                    n1043 = Search 1D Array(1D array=w1894, element="Width (um):") -> (index of element=w1905:i32)  [unwired: 1 in]
                    n1044 = Equal?(x=w1905, y=-1) -> (x = y?=w1904:bool)
                    n1045 = case shown="False" w1904 {
                      tunnel: w1905 -> [w1913 _]
                      tunnel: w1895 -> [w1912 w1918]
                      tunnel: [w1911 w1918] -> w1903
                      frame False {
                        n1046 = local read "New: Width"() -> (w1908:dbl)
                        n1047 = Divide(x=w1913, y=3) -> (x/y=w1915:dbl)
                        n1048 = To Word Integer(number=w1915) -> (16bit integer=w1914:i16)
                        n1049 = Format Value(format string="%#g", value (0)=w1908) -> (output string=w1909:string)  [unwired: 1 in]
                        n1050 = Replace Array Subset(array=w1912, new element=w1909, index (row)=w1914, index (col)=1) -> (w1911:string[][])
                      }
                      frame True {
                      }
                    }
                    n1051 = local write "Save1 Array"(w1903) -> ()
                  }
                  frame #4 {
                    w1928 = "Sample Temp (K):"
                    n1052 = local read "Save1 Array"() -> (w1920:string[][])
                    n1053 = Array Size(array=w1920) -> (size(s)=w1925:i32[])
                    n1054 = Array Subset(array=w1920, index (row)=0, index (col)=0, length (col)=3) -> (w1921:string[][])  [unwired: 1 in]
                    n1055 = Index Array(array=w1925, index=0) -> (element=w1927:i32)
                    n1056 = Reshape Array(w1921, w1927) -> (w1919:string[])
                    n1057 = Search 1D Array(1D array=w1919, element=w1928) -> (index of element=w1931:i32)  [unwired: 1 in]
                    n1058 = Equal?(x=w1931, y=-1) -> (x = y?=w1930:bool)
                    n1059 = case shown="True" w1930 {
                      tunnel: w1920 -> [w1940 w1954]
                      tunnel: w1931 -> [w1937 _]
                      tunnel: [w1936 w1953] -> w1929
                      tunnel: w1919 -> [_ w1956]
                      tunnel: w1928 -> [_ w1943]
                      frame False {
                        n1060 = local read "New: Temp"() -> (w1934:dbl)
                        n1061 = Divide(x=w1937, y=3) -> (x/y=w1939:dbl)
                        n1062 = Format Value(format string="%#g", value (0)=w1934) -> (output string=w1933:string)  [unwired: 1 in]
                        n1063 = To Word Integer(number=w1939) -> (16bit integer=w1938:i16)
                        n1064 = Replace Array Subset(array=w1940, new element=w1933, index (row)=w1938, index (col)=1) -> (w1936:string[][])
                      }
                      frame True {
                        n1065 = local read "New: Temp"() -> (w1945:dbl)
                        n1066 = Search 1D Array(1D array=w1956, element="Width (um):") -> (index of element=w1950:i32)  [unwired: 1 in]
                        n1067 = Divide(x=w1950, y=3) -> (x/y=w1951:dbl)
                        n1068 = To Word Integer(number=w1951) -> (16bit integer=w1949:i16)
                        n1069 = Format Value(format string="%#g", value (0)=w1945) -> (output string=w1944:string)  [unwired: 1 in]
                        n1070 = Build Array(w1943, w1944) -> (w1947:string[])
                        n1071 = Increment(x=w1949) -> (x+1=w1948:i16)
                        n1072 = Insert Into Array(array=w1954, index (row)=w1948, new element=w1947) -> (w1953:string[][])  [unwired: 1 in]
                      }
                    }
                    n1073 = local write "Save1 Array"(w1929) -> ()
                  }
                  frame #5 {
                    w1966 = "Mobility-Sat (cm^2/Vs):"
                    n1074 = local read "Save1 Array"() -> (w1958:string[][])
                    n1075 = Array Size(array=w1958) -> (size(s)=w1963:i32[])
                    n1076 = Array Subset(array=w1958, index (row)=0, index (col)=0, length (col)=3) -> (w1959:string[][])  [unwired: 1 in]
                    n1077 = Index Array(array=w1963, index=0) -> (element=w1965:i32)
                    n1078 = Reshape Array(w1959, w1965) -> (w1957:string[])
                    n1079 = Search 1D Array(1D array=w1957, element=w1966) -> (index of element=w1969:i32)  [unwired: 1 in]
                    n1080 = Equal?(x=w1969, y=-1) -> (x = y?=w1968:bool)
                    n1081 = case shown="True" w1968 {
                      tunnel: w1958 -> [w1978 w1986]
                      tunnel: w1969 -> [w1975 _]
                      tunnel: [w1974 w1985] -> w1967
                      tunnel: w1957 -> [_ w1983]
                      tunnel: w1966 -> [_ w1981]
                      frame False {
                        n1082 = local read "New: Mobility-Sat"() -> (w1971:dbl)
                        n1083 = Divide(x=w1975, y=3) -> (x/y=w1977:dbl)
                        n1084 = To Word Integer(number=w1977) -> (16bit integer=w1976:i16)
                        n1085 = Format Value(format string="%#g", value (0)=w1971) -> (output string=w1972:string)  [unwired: 1 in]
                        n1086 = Replace Array Subset(array=w1978, new element=w1972, index (row)=w1976, index (col)=1) -> (w1974:string[][])
                      }
                      frame True {
                        n1087 = local read "New: Mobility-Sat"() -> (w1987:dbl)
                        n1088 = Search 1D Array(1D array=w1983, element="Mobility (cm^2/Vs):") -> (index of element=w1990:i32)  [unwired: 1 in]
                        n1089 = Divide(x=w1990, y=3) -> (x/y=w1991:dbl)
                        n1090 = To Word Integer(number=w1991) -> (16bit integer=w1982:i16)
                        n1091 = Format Value(format string="%#g", value (0)=w1987) -> (output string=w1984:string)  [unwired: 1 in]
                        n1092 = Build Array(w1981, w1984) -> (w1989:string[])
                        n1093 = Replace Array Subset(array=w1986, new element=w1989, index (row)=w1982) -> (w1985:string[][])  [unwired: 1 in]
                      }
                    }
                    n1094 = local write "Save1 Array"(w1967) -> ()
                  }
                  frame #6 {
                    w2003 = "Mobility-Lin (cm^2/Vs):"
                    n1095 = local read "Save1 Array"() -> (w1994:string[][])
                    n1096 = Array Size(array=w1994) -> (size(s)=w2000:i32[])
                    n1097 = Array Subset(array=w1994, index (row)=0, index (col)=0, length (col)=3) -> (w1996:string[][])  [unwired: 1 in]
                    n1098 = Index Array(array=w2000, index=0) -> (element=w2002:i32)
                    n1099 = Reshape Array(w1996, w2002) -> (w1995:string[])
                    n1100 = Search 1D Array(1D array=w1995, element=w2003) -> (index of element=w2006:i32)  [unwired: 1 in]
                    n1101 = Equal?(x=w2006, y=-1) -> (x = y?=w2005:bool)
                    n1102 = case shown="True" w2005 {
                      tunnel: w1994 -> [w2015 w2021]
                      tunnel: w2006 -> [w2012 _]
                      tunnel: [w2011 w2020] -> w2004
                      tunnel: w1995 -> [_ w2019]
                      tunnel: w2003 -> [_ w2018]
                      frame False {
                        n1103 = local read "Calc: Mobility-Lin"() -> (w2008:dbl)
                        n1104 = Divide(x=w2012, y=3) -> (x/y=w2014:dbl)
                        n1105 = To Word Integer(number=w2014) -> (16bit integer=w2013:i16)
                        n1106 = Format Value(format string="%#g", value (0)=w2008) -> (output string=w2009:string)  [unwired: 1 in]
                        n1107 = Replace Array Subset(array=w2015, new element=w2009, index (row)=w2013, index (col)=1) -> (w2011:string[][])
                      }
                      frame True {
                        n1108 = local read "Calc: Mobility-Lin"() -> (w2022:dbl)
                        n1109 = Search 1D Array(1D array=w2019, element="Mobility-Sat (cm^2/Vs):") -> (index of element=w2027:i32)  [unwired: 1 in]
                        n1110 = Divide(x=w2027, y=3) -> (x/y=w2028:dbl)
                        n1111 = To Word Integer(number=w2028) -> (16bit integer=w2026:i16)
                        n1112 = Format Value(format string="%#g", value (0)=w2022) -> (output string=w2031:string)  [unwired: 1 in]
                        n1113 = Build Array(w2018, w2031) -> (w2024:string[])
                        n1114 = Increment(x=w2026) -> (x+1=w2025:i16)
                        n1115 = Insert Into Array(array=w2021, index (row)=w2025, new element=w2024) -> (w2020:string[][])  [unwired: 1 in]
                      }
                    }
                    n1116 = local write "Save1 Array"(w2004) -> ()
                  }
                  frame #7 {
                    w2041 = "On/Off I-Sat:"
                    n1117 = local read "Save1 Array"() -> (w2032:string[][])
                    n1118 = Array Size(array=w2032) -> (size(s)=w2038:i32[])
                    n1119 = Array Subset(array=w2032, index (row)=0, index (col)=0, length (col)=3) -> (w2034:string[][])  [unwired: 1 in]
                    n1120 = Index Array(array=w2038, index=0) -> (element=w2040:i32)
                    n1121 = Reshape Array(w2034, w2040) -> (w2033:string[])
                    n1122 = Search 1D Array(1D array=w2033, element=w2041) -> (index of element=w2044:i32)  [unwired: 1 in]
                    n1123 = Equal?(x=w2044, y=-1) -> (x = y?=w2043:bool)
                    n1124 = case shown="True" w2043 {
                      tunnel: w2032 -> [w2053 w2060]
                      tunnel: w2044 -> [w2050 _]
                      tunnel: [w2049 w2061] -> w2042
                      tunnel: w2033 -> [_ w2058]
                      tunnel: w2041 -> [_ w2056]
                      frame False {
                        n1125 = local read "Calc: On/Off"() -> (w2046:dbl)
                        n1126 = Divide(x=w2050, y=3) -> (x/y=w2052:dbl)
                        n1127 = To Word Integer(number=w2052) -> (16bit integer=w2051:i16)
                        n1128 = Format Value(format string="%#g", value (0)=w2046) -> (output string=w2047:string)  [unwired: 1 in]
                        n1129 = Replace Array Subset(array=w2053, new element=w2047, index (row)=w2051, index (col)=1) -> (w2049:string[][])
                      }
                      frame True {
                        n1130 = local read "Calc: On/Off"() -> (w2062:dbl)
                        n1131 = Search 1D Array(1D array=w2058, element="On/Off Current:") -> (index of element=w2065:i32)  [unwired: 1 in]
                        n1132 = Divide(x=w2065, y=3) -> (x/y=w2066:dbl)
                        n1133 = To Word Integer(number=w2066) -> (16bit integer=w2057:i16)
                        n1134 = Format Value(format string="%#g", value (0)=w2062) -> (output string=w2059:string)  [unwired: 1 in]
                        n1135 = Build Array(w2056, w2059) -> (w2064:string[])
                        n1136 = Replace Array Subset(array=w2060, new element=w2064, index (row)=w2057) -> (w2061:string[][])  [unwired: 1 in]
                      }
                    }
                    n1137 = local write "Save1 Array"(w2042) -> ()
                  }
                  frame #8 {
                    w2078 = "Off I-Sat (A):"
                    n1138 = local read "Save1 Array"() -> (w2069:string[][])
                    n1139 = Array Size(array=w2069) -> (size(s)=w2075:i32[])
                    n1140 = Array Subset(array=w2069, index (row)=0, index (col)=0, length (col)=3) -> (w2071:string[][])  [unwired: 1 in]
                    n1141 = Index Array(array=w2075, index=0) -> (element=w2077:i32)
                    n1142 = Reshape Array(w2071, w2077) -> (w2070:string[])
                    n1143 = Search 1D Array(1D array=w2070, element=w2078) -> (index of element=w2081:i32)  [unwired: 1 in]
                    n1144 = Equal?(x=w2081, y=-1) -> (x = y?=w2080:bool)
                    n1145 = case shown="True" w2080 {
                      tunnel: w2069 -> [w2090 w2096]
                      tunnel: w2081 -> [w2087 _]
                      tunnel: [w2086 w2095] -> w2079
                      tunnel: w2070 -> [_ w2094]
                      tunnel: w2078 -> [_ w2093]
                      frame False {
                        n1146 = local read "Calc: Off I-Sat"() -> (w2085:dbl)
                        n1147 = Divide(x=w2087, y=3) -> (x/y=w2089:dbl)
                        n1148 = Format Value(format string="%#g", value (0)=w2085) -> (output string=w2083:string)  [unwired: 1 in]
                        n1149 = To Word Integer(number=w2089) -> (16bit integer=w2088:i16)
                        n1150 = Replace Array Subset(array=w2090, new element=w2083, index (row)=w2088, index (col)=1) -> (w2086:string[][])
                      }
                      frame True {
                        n1151 = local read "Calc: Off I-Sat"() -> (w2097:dbl)
                        n1152 = Search 1D Array(1D array=w2094, element="On/Off I-Sat:") -> (index of element=w2102:i32)  [unwired: 1 in]
                        n1153 = Divide(x=w2102, y=3) -> (x/y=w2103:dbl)
                        n1154 = To Word Integer(number=w2103) -> (16bit integer=w2101:i16)
                        n1155 = Format Value(format string="%#g", value (0)=w2097) -> (output string=w2106:string)  [unwired: 1 in]
                        n1156 = Build Array(w2093, w2106) -> (w2099:string[])
                        n1157 = Increment(x=w2101) -> (x+1=w2100:i16)
                        n1158 = Insert Into Array(array=w2096, index (row)=w2100, new element=w2099) -> (w2095:string[][])  [unwired: 1 in]
                      }
                    }
                    n1159 = local write "Save1 Array"(w2079) -> ()
                  }
                  frame #9 {
                    w2108 = "Vt-Sat (V):"
                    n1160 = local read "Save1 Array"() -> (w2109:string[][])
                    n1161 = Array Size(array=w2109) -> (size(s)=w2114:i32[])
                    n1162 = Array Subset(array=w2109, index (row)=0, index (col)=0, length (col)=3) -> (w2110:string[][])  [unwired: 1 in]
                    n1163 = Index Array(array=w2114, index=0) -> (element=w2116:i32)
                    n1164 = Reshape Array(w2110, w2116) -> (w2107:string[])
                    n1165 = Search 1D Array(1D array=w2107, element=w2108) -> (index of element=w2119:i32)  [unwired: 1 in]
                    n1166 = Equal?(x=w2119, y=-1) -> (x = y?=w2118:bool)
                    n1167 = case shown="True" w2118 {
                      tunnel: w2109 -> [w2126 w2135]
                      tunnel: w2119 -> [w2122 _]
                      tunnel: [w2121 w2134] -> w2117
                      tunnel: w2108 -> [_ w2133]
                      tunnel: w2107 -> [_ w2132]
                      frame False {
                        n1168 = local read "New: VT-Sat"() -> (w2128:dbl)
                        n1169 = Number To Fractional String(number=w2128) -> (F-format string=w2123:string)  [unwired: 3 in]
                        n1170 = Divide(x=w2122, y=3) -> (x/y=w2125:dbl)
                        n1171 = To Word Integer(number=w2125) -> (16bit integer=w2124:i16)
                        n1172 = Replace Array Subset(array=w2126, new element=w2123, index (row)=w2124, index (col)=1) -> (w2121:string[][])
                      }
                      frame True {
                        n1173 = local read "New: VT-Sat"() -> (w2136:dbl)
                        n1174 = Search 1D Array(1D array=w2132, element="Threshold V (V):") -> (index of element=w2131:i32)  [unwired: 1 in]
                        n1175 = Divide(x=w2131, y=3) -> (x/y=w2139:dbl)
                        n1176 = To Word Integer(number=w2139) -> (16bit integer=w2130:i16)
                        n1177 = Format Value(format string="%#g", value (0)=w2136) -> (output string=w2142:string)  [unwired: 1 in]
                        n1178 = Build Array(w2133, w2142) -> (w2138:string[])
                        n1179 = Replace Array Subset(array=w2135, new element=w2138, index (row)=w2130) -> (w2134:string[][])  [unwired: 1 in]
                      }
                    }
                    n1180 = local write "Save1 Array"(w2117) -> ()
                  }
                  frame #10 {
                    n1181 = local read "Save1 Array"() -> (w2143:string[][])
                    n1182 = Array Size(array=w2143) -> (size(s)=w2149:i32[])
                    n1183 = Array Subset(array=w2143, index (row)=0, index (col)=0, length (col)=3) -> (w2145:string[][])  [unwired: 1 in]
                    n1184 = Index Array(array=w2149, index=0) -> (element=w2151:i32)
                    n1185 = Reshape Array(w2145, w2151) -> (w2144:string[])
                    n1186 = Search 1D Array(1D array=w2144, element="VT-Lin (V):") -> (index of element=w2154:i32)  [unwired: 1 in]
                    n1187 = Equal?(x=w2154, y=-1) -> (x = y?=w2153:bool)
                    n1188 = case shown="False" w2153 {
                      tunnel: w2143 -> [w2164 w2167]
                      tunnel: w2154 -> [w2161 _]
                      tunnel: [w2160 w2167] -> w2152
                      frame False {
                        n1189 = local read "New: VT-Lin"() -> (w2158:dbl)
                        n1190 = Divide(x=w2161, y=3) -> (x/y=w2163:dbl)
                        n1191 = Format Value(format string="%#g", value (0)=w2158) -> (output string=w2157:string)  [unwired: 1 in]
                        n1192 = To Word Integer(number=w2163) -> (16bit integer=w2162:i16)
                        n1193 = Replace Array Subset(array=w2164, new element=w2157, index (row)=w2162, index (col)=1) -> (w2160:string[][])
                      }
                      frame True {
                      }
                    }
                    n1194 = local write "Save1 Array"(w2152) -> ()
                  }
                  frame #11 {
                    w2168 = "STS-Sat (V/decade):"
                    n1195 = local read "Save1 Array"() -> (w2170:string[][])
                    n1196 = Array Size(array=w2170) -> (size(s)=w2175:i32[])
                    n1197 = Array Subset(array=w2170, index (row)=0, index (col)=0, length (col)=3) -> (w2171:string[][])  [unwired: 1 in]
                    n1198 = Index Array(array=w2175, index=0) -> (element=w2177:i32)
                    n1199 = Reshape Array(w2171, w2177) -> (w2169:string[])
                    n1200 = Search 1D Array(1D array=w2169, element=w2168) -> (index of element=w2180:i32)  [unwired: 1 in]
                    n1201 = Equal?(x=w2180, y=-1) -> (x = y?=w2179:bool)
                    n1202 = case shown="True" w2179 {
                      tunnel: w2170 -> [w2189 w2195]
                      tunnel: w2180 -> [w2186 _]
                      tunnel: [w2185 w2196] -> w2178
                      tunnel: w2169 -> [_ w2194]
                      tunnel: w2168 -> [_ w2193]
                      frame False {
                        n1203 = local read "New: STS"() -> (w2183:dbl)
                        n1204 = Divide(x=w2186, y=3) -> (x/y=w2188:dbl)
                        n1205 = Format Value(format string="%#g", value (0)=w2183) -> (output string=w2182:string)  [unwired: 1 in]
                        n1206 = To Word Integer(number=w2188) -> (16bit integer=w2187:i16)
                        n1207 = Replace Array Subset(array=w2189, new element=w2182, index (row)=w2187, index (col)=1) -> (w2185:string[][])
                      }
                      frame True {
                        n1208 = local read "New: STS"() -> (w2197:dbl)
                        n1209 = Search 1D Array(1D array=w2194, element="S.T.S. (V/decade):") -> (index of element=w2200:i32)  [unwired: 1 in]
                        n1210 = Divide(x=w2200, y=3) -> (x/y=w2201:dbl)
                        n1211 = To Word Integer(number=w2201) -> (16bit integer=w2192:i16)
                        n1212 = Format Value(format string="%#g", value (0)=w2197) -> (output string=w2204:string)  [unwired: 1 in]
                        n1213 = Build Array(w2193, w2204) -> (w2199:string[])
                        n1214 = Replace Array Subset(array=w2195, new element=w2199, index (row)=w2192) -> (w2196:string[][])  [unwired: 1 in]
                      }
                    }
                    n1215 = local write "Save1 Array"(w2178) -> ()
                  }
                  frame #12 {
                    w2205 = "Trap Density-VT (Traps/Vcm^2):"
                    n1216 = local read "Save1 Array"() -> (w2207:string[][])
                    n1217 = Array Size(array=w2207) -> (size(s)=w2212:i32[])
                    n1218 = Array Subset(array=w2207, index (row)=0, index (col)=0, length (col)=3) -> (w2208:string[][])  [unwired: 1 in]
                    n1219 = Index Array(array=w2212, index=0) -> (element=w2214:i32)
                    n1220 = Reshape Array(w2208, w2214) -> (w2206:string[])
                    n1221 = Search 1D Array(1D array=w2206, element=w2205) -> (index of element=w2217:i32)  [unwired: 1 in]
                    n1222 = Equal?(x=w2217, y=-1) -> (x = y?=w2216:bool)
                    n1223 = case shown="True" w2216 {
                      tunnel: w2207 -> [w2226 w2231]
                      tunnel: w2217 -> [w2222 _]
                      tunnel: [w2221 w2232] -> w2215
                      tunnel: w2206 -> [_ w2230]
                      tunnel: w2205 -> [_ w2229]
                      frame False {
                        n1224 = local read "New: Trap Density-VT"() -> (w2220:dbl)
                        n1225 = Format Value(format string="%#g", value (0)=w2220) -> (output string=w2223:string)  [unwired: 1 in]
                        n1226 = Divide(x=w2222, y=3) -> (x/y=w2225:dbl)
                        n1227 = To Word Integer(number=w2225) -> (16bit integer=w2224:i16)
                        n1228 = Replace Array Subset(array=w2226, new element=w2223, index (row)=w2224, index (col)=1) -> (w2221:string[][])
                      }
                      frame True {
                        n1229 = local read "New: Trap Density-VT"() -> (w2242:dbl)
                        n1230 = Search 1D Array(1D array=w2230, element="STS-Sat (V/decade):") -> (index of element=w2237:i32)  [unwired: 1 in]
                        n1231 = Divide(x=w2237, y=3) -> (x/y=w2236:dbl)
                        n1232 = To Word Integer(number=w2236) -> (16bit integer=w2238:i16)
                        n1233 = Format Value(format string="%#g", value (0)=w2242) -> (output string=w2233:string)  [unwired: 1 in]
                        n1234 = Build Array(w2229, w2233) -> (w2240:string[])
                        n1235 = Increment(x=w2238) -> (x+1=w2239:i16)
                        n1236 = Insert Into Array(array=w2231, index (row)=w2239, new element=w2240) -> (w2232:string[][])  [unwired: 1 in]
                      }
                    }
                    n1237 = local write "Save1 Array"(w2215) -> ()
                  }
                  frame #13 {
                    w2243 = "Trap Density-STS (Traps/Vcm^2):"
                    n1238 = local read "Save1 Array"() -> (w2245:string[][])
                    n1239 = Array Size(array=w2245) -> (size(s)=w2250:i32[])
                    n1240 = Array Subset(array=w2245, index (row)=0, index (col)=0, length (col)=3) -> (w2246:string[][])  [unwired: 1 in]
                    n1241 = Index Array(array=w2250, index=0) -> (element=w2252:i32)
                    n1242 = Reshape Array(w2246, w2252) -> (w2244:string[])
                    n1243 = Search 1D Array(1D array=w2244, element=w2243) -> (index of element=w2255:i32)  [unwired: 1 in]
                    n1244 = Equal?(x=w2255, y=-1) -> (x = y?=w2254:bool)
                    n1245 = case shown="True" w2254 {
                      tunnel: w2245 -> [w2264 w2269]
                      tunnel: w2255 -> [w2261 _]
                      tunnel: [w2260 w2270] -> w2253
                      tunnel: w2244 -> [_ w2268]
                      tunnel: w2243 -> [_ w2267]
                      frame False {
                        n1246 = local read "New: Trap Density-STS"() -> (w2258:dbl)
                        n1247 = Divide(x=w2261, y=3) -> (x/y=w2263:dbl)
                        n1248 = To Word Integer(number=w2263) -> (16bit integer=w2262:i16)
                        n1249 = Format Value(format string="%#g", value (0)=w2258) -> (output string=w2257:string)  [unwired: 1 in]
                        n1250 = Replace Array Subset(array=w2264, new element=w2257, index (row)=w2262, index (col)=1) -> (w2260:string[][])
                      }
                      frame True {
                        n1251 = local read "New: Trap Density-STS"() -> (w2271:dbl)
                        n1252 = Search 1D Array(1D array=w2268, element="Trap Density-VT (Traps/Vcm^2):") -> (index of element=w2276:i32)  [unwired: 1 in]
                        n1253 = Divide(x=w2276, y=3) -> (x/y=w2277:dbl)
                        n1254 = To Word Integer(number=w2277) -> (16bit integer=w2275:i16)
                        n1255 = Format Value(format string="%#g", value (0)=w2271) -> (output string=w2280:string)  [unwired: 1 in]
                        n1256 = Build Array(w2267, w2280) -> (w2273:string[])
                        n1257 = Increment(x=w2275) -> (x+1=w2274:i16)
                        n1258 = Insert Into Array(array=w2269, index (row)=w2274, new element=w2273) -> (w2270:string[][])  [unwired: 1 in]
                      }
                    }
                    n1259 = local write "Save1 Array"(w2253) -> ()
                  }
                }
                n1260 = Concatenate Strings(w1818, "\\", w1816) -> (w1817:string)
                n1261 = String To Path(string=w1817) -> (path=w1807:path)
                n1262 = disable-structure shown="Disabled" {
                  frame Disabled {
                  }
                  frame Enabled {
                  }
                }
              }
              frame #2 {
                n1263 = Equal?(x=w2339, y=w2336) -> (x = y?=w2338:bool)
                n1264 = case shown="False" w2338 {
                  tunnel: w2339 -> [w2342 _]
                  tunnel: w2336 -> [w2341 _]
                  frame False {
                    n1265 = Move(source path=w2342, 9:TRUE, 10:w2341) -> ()  [unwired: 2 in, 3 out]
                  }
                  frame True {
                  }
                }
              }
              frame #3 {
                n1266 = local write "Transfer File"(w2343) -> ()
                n1267 = call-poly <vilib>:"Write To Spreadsheet File.vi"("2D data"=w2344, "file path (dialog if empty)"=w2343) -> ()  [unwired: 6 in, 1 out]
              }
            }
          }
          event "Save Changes? 2": Mouse Down {
            n1268 = event-data() -> ()  [unwired: 1 in, 5 out]
            n1269 = stacked-sequence {
              seq-local: [w2402 _ _ _ _] -> [_ w2885 _ _ _]
              seq-local: [w2401 _ _ _ _] -> [_ w2886 _ _ _]
              seq-local: [w2401 _ _ _ _] -> [_ w2884 _ _ _]
              seq-local: [w2403 _ _ _ _] -> [_ w2882 _ _ _]
              seq-local: [_ w2886 _ _ _] -> [_ _ w2891 _ _]
              seq-local: [_ w2882 _ _ _] -> [_ _ w2890 _ _]
              frame #0 {
                n1270 = local read "Transfer File"() -> (w2402:path)
                n1271 = local read "New: Temp"() -> (w2405:dbl)
                n1272 = local read "New: Length"() -> (w2408:dbl)
                n1273 = local read "New: Width"() -> (w2406:dbl)
                n1274 = To Word Integer(number=w2405) -> (16bit integer=w2404:i16)
                n1275 = Number To Decimal String(number=w2404) -> (decimal integer string=w2412:string)  [unwired: 1 in]
                n1276 = To Single Precision Float(number=w2406) -> (single precision float=w2407:sgl)
                n1277 = To Single Precision Float(number=w2408) -> (single precision float=w2409:sgl)
                n1278 = local read "Index"() -> (w2416:string)
                n1279 = Strip Path(path=w2402) -> (stripped path=w2421:path)  [unwired: 1 out]
                n1280 = Number To Decimal String(number=w2409) -> (decimal integer string=w2414:string)  [unwired: 1 in]
                n1281 = Number To Decimal String(number=w2407) -> (decimal integer string=w2415:string)  [unwired: 1 in]
                n1282 = Concatenate Strings("_", w2412, "K") -> (w2410:string)
                n1283 = call "Build Text2"("Temp"=w2410, "Index"=w2416, "Length"=w2414, "Width"=w2415) -> ("Result"=w2417:string)  [unwired: 10 in, 1 out]
                n1284 = Path To String(path=w2421) -> (string=w2419:string)
                n1285 = Concatenate Strings(w2419, "\\", w2417) -> (w2418:string)
                n1286 = stacked-sequence {
                  tunnel: [_ _ _ _ _ _ _ _ _ _ _ _ _ w2844] -> _
                  tunnel: w2402 -> [w2423 _ _ _ _ _ _ _ _ _ _ _ _ _]
                  tunnel: [_ _ _ _ _ _ _ _ _ _ _ _ _ w2844] -> w2403
                  frame #0 {
                    n1287 = call-poly <vilib>:"Read From Spreadsheet File.vi"("file path (dialog if empty)"=w2423) -> ("all rows"=w2422:string[][])  [unwired: 6 in, 4 out]
                    n1288 = Array Size(array=w2422) -> (size(s)=w2427:i32[])
                    n1289 = Array Subset(array=w2422, index (row)=0, index (col)=0, length (col)=3) -> (w2431:string[][])  [unwired: 1 in]
                    n1290 = Index Array(array=w2427, index=0) -> (element=w2425:i32)
                    n1291 = Reshape Array(w2431, w2425) -> (w2424:string[])
                    n1292 = Search 1D Array(1D array=w2424, element="Dielectric (nm):") -> (index of element=w2434:i32)  [unwired: 1 in]
                    n1293 = Equal?(x=w2434, y=-1) -> (x = y?=w2433:bool)
                    n1294 = case shown="False" w2433 {
                      tunnel: w2422 -> [w2442 w2446]
                      tunnel: w2434 -> [w2438 _]
                      tunnel: [w2437 w2446] -> w2432
                      frame False {
                        n1295 = local read "New: Dielectric"() -> (w2444:dbl)
                        n1296 = Number To Fractional String(number=w2444) -> (F-format string=w2439:string)  [unwired: 3 in]
                        n1297 = Divide(x=w2438, y=3) -> (x/y=w2441:dbl)
                        n1298 = To Word Integer(number=w2441) -> (16bit integer=w2440:i16)
                        n1299 = Replace Array Subset(array=w2442, new element=w2439, index (row)=w2440, index (col)=1) -> (w2437:string[][])
                      }
                      frame True {
                      }
                    }
                    n1300 = local write "Save1 Array"(w2432) -> ()
                  }
                  frame #1 {
                    n1301 = local read "Save1 Array"() -> (w2448:string[][])
                    n1302 = Array Size(array=w2448) -> (size(s)=w2451:i32[])
                    n1303 = Array Subset(array=w2448, index (row)=0, index (col)=0, length (col)=3) -> (w2455:string[][])  [unwired: 1 in]
                    n1304 = Index Array(array=w2451, index=0) -> (element=w2449:i32)
                    n1305 = Reshape Array(w2455, w2449) -> (w2447:string[])
                    n1306 = Search 1D Array(1D array=w2447, element="Comments:") -> (index of element=w2458:i32)  [unwired: 1 in]
                    n1307 = Equal?(x=w2458, y=-1) -> (x = y?=w2457:bool)
                    n1308 = case shown="False" w2457 {
                      tunnel: w2448 -> [w2466 w2469]
                      tunnel: w2458 -> [w2463 _]
                      tunnel: [w2462 w2469] -> w2456
                      frame False {
                        n1309 = local read "Comments:"() -> (w2461:string)
                        n1310 = Divide(x=w2463, y=3) -> (x/y=w2465:dbl)
                        n1311 = To Word Integer(number=w2465) -> (16bit integer=w2464:i16)
                        n1312 = Replace Array Subset(array=w2466, new element=w2461, index (row)=w2464, index (col)=1) -> (w2462:string[][])
                      }
                      frame True {
                      }
                    }
                    n1313 = local write "Save1 Array"(w2456) -> ()
                  }
                  frame #2 {
                    n1314 = local read "Save1 Array"() -> (w2471:string[][])
                    n1315 = Array Size(array=w2471) -> (size(s)=w2474:i32[])
                    n1316 = Array Subset(array=w2471, index (row)=0, index (col)=0, length (col)=3) -> (w2478:string[][])  [unwired: 1 in]
                    n1317 = Index Array(array=w2474, index=0) -> (element=w2472:i32)
                    n1318 = Reshape Array(w2478, w2472) -> (w2470:string[])
                    n1319 = Search 1D Array(1D array=w2470, element="Length (um):") -> (index of element=w2481:i32)  [unwired: 1 in]
                    n1320 = Equal?(x=w2481, y=-1) -> (x = y?=w2480:bool)
                    n1321 = case shown="False" w2480 {
                      tunnel: w2471 -> [w2491 w2494]
                      tunnel: w2481 -> [w2488 _]
                      tunnel: [w2487 w2494] -> w2479
                      frame False {
                        n1322 = local read "New: Length"() -> (w2484:dbl)
                        n1323 = Divide(x=w2488, y=3) -> (x/y=w2490:dbl)
                        n1324 = Format Value(format string="%#g", value (0)=w2484) -> (output string=w2485:string)  [unwired: 1 in]
                        n1325 = To Word Integer(number=w2490) -> (16bit integer=w2489:i16)
                        n1326 = Replace Array Subset(array=w2491, new element=w2485, index (row)=w2489, index (col)=1) -> (w2487:string[][])
                      }
                      frame True {
                      }
                    }
                    n1327 = local write "Save1 Array"(w2479) -> ()
                  }
                  frame #3 {
                    n1328 = local read "Save1 Array"() -> (w2496:string[][])
                    n1329 = Array Size(array=w2496) -> (size(s)=w2501:i32[])
                    n1330 = Array Subset(array=w2496, index (row)=0, index (col)=0, length (col)=3) -> (w2497:string[][])  [unwired: 1 in]
                    n1331 = Index Array(array=w2501, index=0) -> (element=w2503:i32)
                    n1332 = Reshape Array(w2497, w2503) -> (w2495:string[])
                    n1333 = Search 1D Array(1D array=w2495, element="Width (um):") -> (index of element=w2506:i32)  [unwired: 1 in]
                    n1334 = Equal?(x=w2506, y=-1) -> (x = y?=w2505:bool)
                    n1335 = case shown="False" w2505 {
                      tunnel: w2506 -> [w2514 _]
                      tunnel: w2496 -> [w2513 w2519]
                      tunnel: [w2512 w2519] -> w2504
                      frame False {
                        n1336 = local read "New: Width"() -> (w2509:dbl)
                        n1337 = Divide(x=w2514, y=3) -> (x/y=w2516:dbl)
                        n1338 = To Word Integer(number=w2516) -> (16bit integer=w2515:i16)
                        n1339 = Format Value(format string="%#g", value (0)=w2509) -> (output string=w2510:string)  [unwired: 1 in]
                        n1340 = Replace Array Subset(array=w2513, new element=w2510, index (row)=w2515, index (col)=1) -> (w2512:string[][])
                      }
                      frame True {
                      }
                    }
                    n1341 = local write "Save1 Array"(w2504) -> ()
                  }
                  frame #4 {
                    w2529 = "Sample Temp (K):"
                    n1342 = local read "Save1 Array"() -> (w2521:string[][])
                    n1343 = Array Size(array=w2521) -> (size(s)=w2526:i32[])
                    n1344 = Array Subset(array=w2521, index (row)=0, index (col)=0, length (col)=3) -> (w2522:string[][])  [unwired: 1 in]
                    n1345 = Index Array(array=w2526, index=0) -> (element=w2528:i32)
                    n1346 = Reshape Array(w2522, w2528) -> (w2520:string[])
                    n1347 = Search 1D Array(1D array=w2520, element=w2529) -> (index of element=w2532:i32)  [unwired: 1 in]
                    n1348 = Equal?(x=w2532, y=-1) -> (x = y?=w2531:bool)
                    n1349 = case shown="True" w2531 {
                      tunnel: w2521 -> [w2541 w2555]
                      tunnel: w2532 -> [w2538 _]
                      tunnel: [w2537 w2554] -> w2530
                      tunnel: w2520 -> [_ w2557]
                      tunnel: w2529 -> [_ w2544]
                      frame False {
                        n1350 = local read "New: Temp"() -> (w2535:dbl)
                        n1351 = Divide(x=w2538, y=3) -> (x/y=w2540:dbl)
                        n1352 = Format Value(format string="%#g", value (0)=w2535) -> (output string=w2534:string)  [unwired: 1 in]
                        n1353 = To Word Integer(number=w2540) -> (16bit integer=w2539:i16)
                        n1354 = Replace Array Subset(array=w2541, new element=w2534, index (row)=w2539, index (col)=1) -> (w2537:string[][])
                      }
                      frame True {
                        n1355 = local read "New: Temp"() -> (w2546:dbl)
                        n1356 = Search 1D Array(1D array=w2557, element="Width (um):") -> (index of element=w2551:i32)  [unwired: 1 in]
                        n1357 = Divide(x=w2551, y=3) -> (x/y=w2552:dbl)
                        n1358 = To Word Integer(number=w2552) -> (16bit integer=w2550:i16)
                        n1359 = Format Value(format string="%#g", value (0)=w2546) -> (output string=w2545:string)  [unwired: 1 in]
                        n1360 = Build Array(w2544, w2545) -> (w2548:string[])
                        n1361 = Increment(x=w2550) -> (x+1=w2549:i16)
                        n1362 = Insert Into Array(array=w2555, index (row)=w2549, new element=w2548) -> (w2554:string[][])  [unwired: 1 in]
                      }
                    }
                    n1363 = local write "Save1 Array"(w2530) -> ()
                  }
                  frame #5 {
                    w2567 = "Mobility-Sat (cm^2/Vs):"
                    n1364 = local read "Save1 Array"() -> (w2559:string[][])
                    n1365 = Array Size(array=w2559) -> (size(s)=w2564:i32[])
                    n1366 = Array Subset(array=w2559, index (row)=0, index (col)=0, length (col)=3) -> (w2560:string[][])  [unwired: 1 in]
                    n1367 = Index Array(array=w2564, index=0) -> (element=w2566:i32)
                    n1368 = Reshape Array(w2560, w2566) -> (w2558:string[])
                    n1369 = Search 1D Array(1D array=w2558, element=w2567) -> (index of element=w2570:i32)  [unwired: 1 in]
                    n1370 = Equal?(x=w2570, y=-1) -> (x = y?=w2569:bool)
                    n1371 = case shown="True" w2569 {
                      tunnel: w2559 -> [w2579 w2587]
                      tunnel: w2570 -> [w2576 _]
                      tunnel: [w2575 w2586] -> w2568
                      tunnel: w2558 -> [_ w2584]
                      tunnel: w2567 -> [_ w2582]
                      frame False {
                        n1372 = local read "New: Mobility-Sat"() -> (w2572:dbl)
                        n1373 = Divide(x=w2576, y=3) -> (x/y=w2578:dbl)
                        n1374 = To Word Integer(number=w2578) -> (16bit integer=w2577:i16)
                        n1375 = Format Value(format string="%#g", value (0)=w2572) -> (output string=w2573:string)  [unwired: 1 in]
                        n1376 = Replace Array Subset(array=w2579, new element=w2573, index (row)=w2577, index (col)=1) -> (w2575:string[][])
                      }
                      frame True {
                        n1377 = local read "New: Mobility-Sat"() -> (w2588:dbl)
                        n1378 = Search 1D Array(1D array=w2584, element="Mobility (cm^2/Vs):") -> (index of element=w2591:i32)  [unwired: 1 in]
                        n1379 = Divide(x=w2591, y=3) -> (x/y=w2592:dbl)
                        n1380 = To Word Integer(number=w2592) -> (16bit integer=w2583:i16)
                        n1381 = Format Value(format string="%#g", value (0)=w2588) -> (output string=w2585:string)  [unwired: 1 in]
                        n1382 = Build Array(w2582, w2585) -> (w2590:string[])
                        n1383 = Replace Array Subset(array=w2587, new element=w2590, index (row)=w2583) -> (w2586:string[][])  [unwired: 1 in]
                      }
                    }
                    n1384 = local write "Save1 Array"(w2568) -> ()
                  }
                  frame #6 {
                    w2604 = "Mobility-Lin (cm^2/Vs):"
                    n1385 = local read "Save1 Array"() -> (w2595:string[][])
                    n1386 = Array Size(array=w2595) -> (size(s)=w2601:i32[])
                    n1387 = Array Subset(array=w2595, index (row)=0, index (col)=0, length (col)=3) -> (w2597:string[][])  [unwired: 1 in]
                    n1388 = Index Array(array=w2601, index=0) -> (element=w2603:i32)
                    n1389 = Reshape Array(w2597, w2603) -> (w2596:string[])
                    n1390 = Search 1D Array(1D array=w2596, element=w2604) -> (index of element=w2607:i32)  [unwired: 1 in]
                    n1391 = Equal?(x=w2607, y=-1) -> (x = y?=w2606:bool)
                    n1392 = case shown="True" w2606 {
                      tunnel: w2595 -> [w2616 w2622]
                      tunnel: w2607 -> [w2613 _]
                      tunnel: [w2612 w2621] -> w2605
                      tunnel: w2596 -> [_ w2620]
                      tunnel: w2604 -> [_ w2619]
                      frame False {
                        n1393 = local read "Calc: Mobility-Lin"() -> (w2609:dbl)
                        n1394 = Divide(x=w2613, y=3) -> (x/y=w2615:dbl)
                        n1395 = To Word Integer(number=w2615) -> (16bit integer=w2614:i16)
                        n1396 = Format Value(format string="%#g", value (0)=w2609) -> (output string=w2610:string)  [unwired: 1 in]
                        n1397 = Replace Array Subset(array=w2616, new element=w2610, index (row)=w2614, index (col)=1) -> (w2612:string[][])
                      }
                      frame True {
                        n1398 = local read "Calc: Mobility-Lin"() -> (w2623:dbl)
                        n1399 = Search 1D Array(1D array=w2620, element="Mobility-Sat (cm^2/Vs):") -> (index of element=w2628:i32)  [unwired: 1 in]
                        n1400 = Divide(x=w2628, y=3) -> (x/y=w2629:dbl)
                        n1401 = To Word Integer(number=w2629) -> (16bit integer=w2627:i16)
                        n1402 = Format Value(format string="%#g", value (0)=w2623) -> (output string=w2632:string)  [unwired: 1 in]
                        n1403 = Build Array(w2619, w2632) -> (w2625:string[])
                        n1404 = Increment(x=w2627) -> (x+1=w2626:i16)
                        n1405 = Insert Into Array(array=w2622, index (row)=w2626, new element=w2625) -> (w2621:string[][])  [unwired: 1 in]
                      }
                    }
                    n1406 = local write "Save1 Array"(w2605) -> ()
                  }
                  frame #7 {
                    w2642 = "On/Off I-Sat:"
                    n1407 = local read "Save1 Array"() -> (w2633:string[][])
                    n1408 = Array Size(array=w2633) -> (size(s)=w2639:i32[])
                    n1409 = Array Subset(array=w2633, index (row)=0, index (col)=0, length (col)=3) -> (w2635:string[][])  [unwired: 1 in]
                    n1410 = Index Array(array=w2639, index=0) -> (element=w2641:i32)
                    n1411 = Reshape Array(w2635, w2641) -> (w2634:string[])
                    n1412 = Search 1D Array(1D array=w2634, element=w2642) -> (index of element=w2645:i32)  [unwired: 1 in]
                    n1413 = Equal?(x=w2645, y=-1) -> (x = y?=w2644:bool)
                    n1414 = case shown="True" w2644 {
                      tunnel: w2633 -> [w2654 w2661]
                      tunnel: w2645 -> [w2651 _]
                      tunnel: [w2650 w2662] -> w2643
                      tunnel: w2634 -> [_ w2659]
                      tunnel: w2642 -> [_ w2657]
                      frame False {
                        n1415 = local read "Calc: On/Off"() -> (w2647:dbl)
                        n1416 = Divide(x=w2651, y=3) -> (x/y=w2653:dbl)
                        n1417 = To Word Integer(number=w2653) -> (16bit integer=w2652:i16)
                        n1418 = Format Value(format string="%#g", value (0)=w2647) -> (output string=w2648:string)  [unwired: 1 in]
                        n1419 = Replace Array Subset(array=w2654, new element=w2648, index (row)=w2652, index (col)=1) -> (w2650:string[][])
                      }
                      frame True {
                        n1420 = local read "Calc: On/Off"() -> (w2663:dbl)
                        n1421 = Search 1D Array(1D array=w2659, element="On/Off Current:") -> (index of element=w2666:i32)  [unwired: 1 in]
                        n1422 = Divide(x=w2666, y=3) -> (x/y=w2667:dbl)
                        n1423 = To Word Integer(number=w2667) -> (16bit integer=w2658:i16)
                        n1424 = Format Value(format string="%#g", value (0)=w2663) -> (output string=w2660:string)  [unwired: 1 in]
                        n1425 = Build Array(w2657, w2660) -> (w2665:string[])
                        n1426 = Replace Array Subset(array=w2661, new element=w2665, index (row)=w2658) -> (w2662:string[][])  [unwired: 1 in]
                      }
                    }
                    n1427 = local write "Save1 Array"(w2643) -> ()
                  }
                  frame #8 {
                    w2679 = "Off I-Sat (A):"
                    n1428 = local read "Save1 Array"() -> (w2670:string[][])
                    n1429 = Array Size(array=w2670) -> (size(s)=w2676:i32[])
                    n1430 = Array Subset(array=w2670, index (row)=0, index (col)=0, length (col)=3) -> (w2672:string[][])  [unwired: 1 in]
                    n1431 = Index Array(array=w2676, index=0) -> (element=w2678:i32)
                    n1432 = Reshape Array(w2672, w2678) -> (w2671:string[])
                    n1433 = Search 1D Array(1D array=w2671, element=w2679) -> (index of element=w2682:i32)  [unwired: 1 in]
                    n1434 = Equal?(x=w2682, y=-1) -> (x = y?=w2681:bool)
                    n1435 = case shown="True" w2681 {
                      tunnel: w2670 -> [w2691 w2697]
                      tunnel: w2682 -> [w2688 _]
                      tunnel: [w2687 w2696] -> w2680
                      tunnel: w2671 -> [_ w2695]
                      tunnel: w2679 -> [_ w2694]
                      frame False {
                        n1436 = local read "Calc: Off I-Sat"() -> (w2686:dbl)
                        n1437 = Divide(x=w2688, y=3) -> (x/y=w2690:dbl)
                        n1438 = Format Value(format string="%#g", value (0)=w2686) -> (output string=w2684:string)  [unwired: 1 in]
                        n1439 = To Word Integer(number=w2690) -> (16bit integer=w2689:i16)
                        n1440 = Replace Array Subset(array=w2691, new element=w2684, index (row)=w2689, index (col)=1) -> (w2687:string[][])
                      }
                      frame True {
                        n1441 = local read "Calc: Off I-Sat"() -> (w2698:dbl)
                        n1442 = Search 1D Array(1D array=w2695, element="On/Off I-Sat:") -> (index of element=w2703:i32)  [unwired: 1 in]
                        n1443 = Divide(x=w2703, y=3) -> (x/y=w2704:dbl)
                        n1444 = To Word Integer(number=w2704) -> (16bit integer=w2702:i16)
                        n1445 = Format Value(format string="%#g", value (0)=w2698) -> (output string=w2707:string)  [unwired: 1 in]
                        n1446 = Build Array(w2694, w2707) -> (w2700:string[])
                        n1447 = Increment(x=w2702) -> (x+1=w2701:i16)
                        n1448 = Insert Into Array(array=w2697, index (row)=w2701, new element=w2700) -> (w2696:string[][])  [unwired: 1 in]
                      }
                    }
                    n1449 = local write "Save1 Array"(w2680) -> ()
                  }
                  frame #9 {
                    w2709 = "Vt-Sat (V):"
                    n1450 = local read "Save1 Array"() -> (w2710:string[][])
                    n1451 = Array Size(array=w2710) -> (size(s)=w2715:i32[])
                    n1452 = Array Subset(array=w2710, index (row)=0, index (col)=0, length (col)=3) -> (w2711:string[][])  [unwired: 1 in]
                    n1453 = Index Array(array=w2715, index=0) -> (element=w2717:i32)
                    n1454 = Reshape Array(w2711, w2717) -> (w2708:string[])
                    n1455 = Search 1D Array(1D array=w2708, element=w2709) -> (index of element=w2720:i32)  [unwired: 1 in]
                    n1456 = Equal?(x=w2720, y=-1) -> (x = y?=w2719:bool)
                    n1457 = case shown="True" w2719 {
                      tunnel: w2710 -> [w2727 w2736]
                      tunnel: w2720 -> [w2723 _]
                      tunnel: [w2722 w2735] -> w2718
                      tunnel: w2709 -> [_ w2734]
                      tunnel: w2708 -> [_ w2733]
                      frame False {
                        n1458 = local read "New: VT-Sat"() -> (w2729:dbl)
                        n1459 = Number To Fractional String(number=w2729) -> (F-format string=w2724:string)  [unwired: 3 in]
                        n1460 = Divide(x=w2723, y=3) -> (x/y=w2726:dbl)
                        n1461 = To Word Integer(number=w2726) -> (16bit integer=w2725:i16)
                        n1462 = Replace Array Subset(array=w2727, new element=w2724, index (row)=w2725, index (col)=1) -> (w2722:string[][])
                      }
                      frame True {
                        n1463 = local read "New: VT-Sat"() -> (w2737:dbl)
                        n1464 = Search 1D Array(1D array=w2733, element="Threshold V (V):") -> (index of element=w2732:i32)  [unwired: 1 in]
                        n1465 = Divide(x=w2732, y=3) -> (x/y=w2740:dbl)
                        n1466 = To Word Integer(number=w2740) -> (16bit integer=w2731:i16)
                        n1467 = Format Value(format string="%#g", value (0)=w2737) -> (output string=w2743:string)  [unwired: 1 in]
                        n1468 = Build Array(w2734, w2743) -> (w2739:string[])
                        n1469 = Replace Array Subset(array=w2736, new element=w2739, index (row)=w2731) -> (w2735:string[][])  [unwired: 1 in]
                      }
                    }
                    n1470 = local write "Save1 Array"(w2718) -> ()
                  }
                  frame #10 {
                    n1471 = local read "Save1 Array"() -> (w2744:string[][])
                    n1472 = Array Size(array=w2744) -> (size(s)=w2750:i32[])
                    n1473 = Array Subset(array=w2744, index (row)=0, index (col)=0, length (col)=3) -> (w2746:string[][])  [unwired: 1 in]
                    n1474 = Index Array(array=w2750, index=0) -> (element=w2752:i32)
                    n1475 = Reshape Array(w2746, w2752) -> (w2745:string[])
                    n1476 = Search 1D Array(1D array=w2745, element="VT-Lin (V):") -> (index of element=w2755:i32)  [unwired: 1 in]
                    n1477 = Equal?(x=w2755, y=-1) -> (x = y?=w2754:bool)
                    n1478 = case shown="False" w2754 {
                      tunnel: w2744 -> [w2765 w2768]
                      tunnel: w2755 -> [w2762 _]
                      tunnel: [w2761 w2768] -> w2753
                      frame False {
                        n1479 = local read "New: VT-Lin"() -> (w2759:dbl)
                        n1480 = Divide(x=w2762, y=3) -> (x/y=w2764:dbl)
                        n1481 = Format Value(format string="%#g", value (0)=w2759) -> (output string=w2758:string)  [unwired: 1 in]
                        n1482 = To Word Integer(number=w2764) -> (16bit integer=w2763:i16)
                        n1483 = Replace Array Subset(array=w2765, new element=w2758, index (row)=w2763, index (col)=1) -> (w2761:string[][])
                      }
                      frame True {
                      }
                    }
                    n1484 = local write "Save1 Array"(w2753) -> ()
                  }
                  frame #11 {
                    w2769 = "STS-Sat (V/decade):"
                    n1485 = local read "Save1 Array"() -> (w2771:string[][])
                    n1486 = Array Size(array=w2771) -> (size(s)=w2776:i32[])
                    n1487 = Array Subset(array=w2771, index (row)=0, index (col)=0, length (col)=3) -> (w2772:string[][])  [unwired: 1 in]
                    n1488 = Index Array(array=w2776, index=0) -> (element=w2778:i32)
                    n1489 = Reshape Array(w2772, w2778) -> (w2770:string[])
                    n1490 = Search 1D Array(1D array=w2770, element=w2769) -> (index of element=w2781:i32)  [unwired: 1 in]
                    n1491 = Equal?(x=w2781, y=-1) -> (x = y?=w2780:bool)
                    n1492 = case shown="True" w2780 {
                      tunnel: w2771 -> [w2790 w2796]
                      tunnel: w2781 -> [w2787 _]
                      tunnel: [w2786 w2797] -> w2779
                      tunnel: w2770 -> [_ w2795]
                      tunnel: w2769 -> [_ w2794]
                      frame False {
                        n1493 = local read "New: STS"() -> (w2784:dbl)
                        n1494 = Divide(x=w2787, y=3) -> (x/y=w2789:dbl)
                        n1495 = Format Value(format string="%#g", value (0)=w2784) -> (output string=w2783:string)  [unwired: 1 in]
                        n1496 = To Word Integer(number=w2789) -> (16bit integer=w2788:i16)
                        n1497 = Replace Array Subset(array=w2790, new element=w2783, index (row)=w2788, index (col)=1) -> (w2786:string[][])
                      }
                      frame True {
                        n1498 = local read "New: STS"() -> (w2798:dbl)
                        n1499 = Search 1D Array(1D array=w2795, element="S.T.S. (V/decade):") -> (index of element=w2801:i32)  [unwired: 1 in]
                        n1500 = Divide(x=w2801, y=3) -> (x/y=w2802:dbl)
                        n1501 = To Word Integer(number=w2802) -> (16bit integer=w2793:i16)
                        n1502 = Format Value(format string="%#g", value (0)=w2798) -> (output string=w2805:string)  [unwired: 1 in]
                        n1503 = Build Array(w2794, w2805) -> (w2800:string[])
                        n1504 = Replace Array Subset(array=w2796, new element=w2800, index (row)=w2793) -> (w2797:string[][])  [unwired: 1 in]
                      }
                    }
                    n1505 = local write "Save1 Array"(w2779) -> ()
                  }
                  frame #12 {
                    w2806 = "Trap Density-VT (Traps/Vcm^2):"
                    n1506 = local read "Save1 Array"() -> (w2808:string[][])
                    n1507 = Array Size(array=w2808) -> (size(s)=w2813:i32[])
                    n1508 = Array Subset(array=w2808, index (row)=0, index (col)=0, length (col)=3) -> (w2809:string[][])  [unwired: 1 in]
                    n1509 = Index Array(array=w2813, index=0) -> (element=w2815:i32)
                    n1510 = Reshape Array(w2809, w2815) -> (w2807:string[])
                    n1511 = Search 1D Array(1D array=w2807, element=w2806) -> (index of element=w2818:i32)  [unwired: 1 in]
                    n1512 = Equal?(x=w2818, y=-1) -> (x = y?=w2817:bool)
                    n1513 = case shown="True" w2817 {
                      tunnel: w2808 -> [w2827 w2832]
                      tunnel: w2818 -> [w2823 _]
                      tunnel: [w2822 w2833] -> w2816
                      tunnel: w2807 -> [_ w2831]
                      tunnel: w2806 -> [_ w2830]
                      frame False {
                        n1514 = local read "New: Trap Density-VT"() -> (w2821:dbl)
                        n1515 = Format Value(format string="%#g", value (0)=w2821) -> (output string=w2824:string)  [unwired: 1 in]
                        n1516 = Divide(x=w2823, y=3) -> (x/y=w2826:dbl)
                        n1517 = To Word Integer(number=w2826) -> (16bit integer=w2825:i16)
                        n1518 = Replace Array Subset(array=w2827, new element=w2824, index (row)=w2825, index (col)=1) -> (w2822:string[][])
                      }
                      frame True {
                        n1519 = local read "New: Trap Density-VT"() -> (w2843:dbl)
                        n1520 = Search 1D Array(1D array=w2831, element="STS-Sat (V/decade):") -> (index of element=w2838:i32)  [unwired: 1 in]
                        n1521 = Divide(x=w2838, y=3) -> (x/y=w2837:dbl)
                        n1522 = To Word Integer(number=w2837) -> (16bit integer=w2839:i16)
                        n1523 = Format Value(format string="%#g", value (0)=w2843) -> (output string=w2834:string)  [unwired: 1 in]
                        n1524 = Build Array(w2830, w2834) -> (w2841:string[])
                        n1525 = Increment(x=w2839) -> (x+1=w2840:i16)
                        n1526 = Insert Into Array(array=w2832, index (row)=w2840, new element=w2841) -> (w2833:string[][])  [unwired: 1 in]
                      }
                    }
                    n1527 = local write "Save1 Array"(w2816) -> ()
                  }
                  frame #13 {
                    w2845 = "Trap Density-STS (Traps/Vcm^2):"
                    n1528 = local read "Save1 Array"() -> (w2847:string[][])
                    n1529 = Array Size(array=w2847) -> (size(s)=w2852:i32[])
                    n1530 = Array Subset(array=w2847, index (row)=0, index (col)=0, length (col)=3) -> (w2848:string[][])  [unwired: 1 in]
                    n1531 = Index Array(array=w2852, index=0) -> (element=w2854:i32)
                    n1532 = Reshape Array(w2848, w2854) -> (w2846:string[])
                    n1533 = Search 1D Array(1D array=w2846, element=w2845) -> (index of element=w2856:i32)  [unwired: 1 in]
                    n1534 = Equal?(x=w2856, y=-1) -> (x = y?=w2855:bool)
                    n1535 = case shown="True" w2855 {
                      tunnel: w2847 -> [w2865 w2870]
                      tunnel: w2856 -> [w2862 _]
                      tunnel: [w2861 w2871] -> w2844
                      tunnel: w2846 -> [_ w2869]
                      tunnel: w2845 -> [_ w2868]
                      frame False {
                        n1536 = local read "New: Trap Density-STS"() -> (w2859:dbl)
                        n1537 = Divide(x=w2862, y=3) -> (x/y=w2864:dbl)
                        n1538 = To Word Integer(number=w2864) -> (16bit integer=w2863:i16)
                        n1539 = Format Value(format string="%#g", value (0)=w2859) -> (output string=w2858:string)  [unwired: 1 in]
                        n1540 = Replace Array Subset(array=w2865, new element=w2858, index (row)=w2863, index (col)=1) -> (w2861:string[][])
                      }
                      frame True {
                        n1541 = local read "New: Trap Density-STS"() -> (w2872:dbl)
                        n1542 = Search 1D Array(1D array=w2869, element="Trap Density-VT (Traps/Vcm^2):") -> (index of element=w2877:i32)  [unwired: 1 in]
                        n1543 = Divide(x=w2877, y=3) -> (x/y=w2878:dbl)
                        n1544 = To Word Integer(number=w2878) -> (16bit integer=w2876:i16)
                        n1545 = Format Value(format string="%#g", value (0)=w2872) -> (output string=w2881:string)  [unwired: 1 in]
                        n1546 = Build Array(w2868, w2881) -> (w2874:string[])
                        n1547 = Increment(x=w2876) -> (x+1=w2875:i16)
                        n1548 = Insert Into Array(array=w2870, index (row)=w2875, new element=w2874) -> (w2871:string[][])  [unwired: 1 in]
                      }
                    }
                    n1549 = local write "Save1 Array"(w2844) -> ()
                  }
                }
                n1550 = String To Path(string=w2418) -> (path=w2401:path)
                "No Image 2" <- w2401
              }
              frame #1 {
                n1551 = Equal?(x=w2885, y=w2884) -> (x = y?=w2883:bool)
                n1552 = case shown="False" w2883 {
                  tunnel: w2885 -> [w2889 _]
                  tunnel: w2884 -> [w2888 _]
                  frame False {
                    n1553 = Move(source path=w2889, 9:TRUE, 10:w2888) -> ()  [unwired: 2 in, 3 out]
                  }
                  frame True {
                  }
                }
              }
              frame #2 {
                n1554 = local write "Transfer File"(w2891) -> ()
                n1555 = call-poly <vilib>:"Write To Spreadsheet File.vi"("2D data"=w2890, "file path (dialog if empty)"=w2891) -> ()  [unwired: 6 in, 1 out]
              }
              frame #3 {
                w2996 = 0
                # "Moves to next file and displays new image/data"
                n1556 = property on="Image Out" class="ImageControl"() -> (error out=w2958:errorcluster, "Image Center Position"=w2962:cluster{"X":u32, "Y":u32})  [unwired: 2 in, 1 out]
                n1557 = local read "Transfer File"() -> (w3001:path)
                n1558 = Strip Path(path=w3001) -> (stripped path=w2992:path, name=w3010:string)
                n1559 = Unbundle(w2962) -> ("X"=w2960:u32)  [unwired: 1 out]
                n1560 = local write "Transfer Folder"(w2992) -> ()
                n1561 = Bundle("X"=w2960, 0) -> (w2961:cluster{"X":u32, i32})  [unwired: 1 in]
                n1562 = property on="Image Out" class="ImageControl"(error in=w2958, "Image Center Position"=w2961) -> ()  [unwired: 1 in, 2 out]
                n1563 = List Folder(path=w2992) -> (filenames=w3006:string[])  [unwired: 3 in, 3 out]
                n1564 = Search 1D Array(1D array=w3006, element=w3010) -> (index of element=w3003:i32)  [unwired: 1 in]
                n1565 = Array Size(array=w3006) -> (size(s)=w3002:i32)
                n1566 = Decrement(x=w3002) -> (x-1=w3004:i32)
                n1567 = Equal?(x=w3003, y=w3004) -> (x = y?=w3005:bool)
                n1568 = local read "Folder Index"() -> (w2954:dbl)
                n1569 = case shown="False" w3005 {
                  tunnel: w2954 -> [w3135 _]
                  tunnel: [w3134 0] -> w2953
                  frame False {
                    n1570 = Increment(x=w3135) -> (x+1=w3134:dbl)
                  }
                  frame True {
                  }
                }
                n1571 = invoke on="Image Out" class="ImageControl" method="Clear ROI"() -> ()  [unwired: 3 in, 3 out]
                n1572 = local write "Folder Index"(w2953) -> ()
                n1573 = Path To String(path=w2992) -> (string=w3011:string)
                n1574 = Index Array(array=w3006, index=w2953) -> (element=w3007:string)
                n1575 = local write "Data Name:"(w3007) -> ()
                n1576 = Concatenate Strings(w3011, "\\", w3007) -> (w3009:string)
                n1577 = String To Path(string=w3009) -> (path=w2907:path)
                n1578 = call "Recorded Values.vi"("Path"=w2907) -> ("Recorded Char"=w2909:T6, "Recorded Prop"=w2910:T7, "Fabrication Prop"=w2908:T8)  [unwired: 8 in]
                n1579 = Unbundle By Name(w2909) -> ("Mobility-Sat"=w2922:dbl, "Moblitity-Lin"=w2923:dbl, "On/Off"=w2924:dbl, "Off Current"=w2925:dbl, "Vt-Sat"=w2901:dbl, "STS"=w2926:dbl, "Trap Density-VT"=w2927:dbl, "Trap Density-STS"=w2928:dbl)
                n1580 = Unbundle By Name(w2910) -> ("Date Recorded"=w2918:string, "Index"=w2919:string, "Length"=w2920:dbl, "Width"=w2921:dbl, "Sample Temp"=w2904:dbl)
                n1581 = Unbundle By Name(w2908) -> ("Date Created"=w2929:string, "Material"=w2911:string, "Solvent"=w2912:string, "Concentration"=w2913:dbl, "Method"=w2914:string, "Dielectric (nm)"=w2915:dbl, "Treatment"=w2916:string, "Comments"=w2917:string)
                n1582 = local write "Rec: Off I-Sat"(w2925) -> ()
                n1583 = local write "Rec: Comments"(w2917) -> ()
                n1584 = local write "Rec: VT-Sat"(w2901) -> ()
                n1585 = local write "Date Created"(w2929) -> ()
                n1586 = local write "Rec: Material"(w2911) -> ()
                n1587 = local write "Rec: Solvent"(w2912) -> ()
                n1588 = local write "Rec: Concentration"(w2913) -> ()
                n1589 = local write "Rec: Method"(w2914) -> ()
                n1590 = local write "Rec: Dielectric (d)"(w2915) -> ()
                n1591 = local write "Surface Treatment:"(w2916) -> ()
                n1592 = local write "Index"(w2919) -> ()
                n1593 = local write "Rec: Mobility-Sat"(w2922) -> ()
                n1594 = local write "Rec: Mobility-Lin"(w2923) -> ()
                n1595 = local write "Rec: On/Off"(w2924) -> ()
                n1596 = local write "Rec: STS"(w2926) -> ()
                n1597 = local write "Rec: Trap Density-VT"(w2927) -> ()
                n1598 = local write "Rec: Trap Density-STS"(w2928) -> ()
                n1599 = local write "Date Recorded"(w2918) -> ()
                n1600 = local write "Rec: Length"(w2920) -> ()
                n1601 = local write "Rec: Width"(w2921) -> ()
                n1602 = local write "Rec: Temp"(w2904) -> ()
                n1603 = Equal To 0?(x=w2904) -> (x = 0?=w2905:bool)
                n1604 = case shown="False" w2905 {
                  tunnel: [w3012 w3013] -> w2902
                  tunnel: w2904 -> [w3012 _]
                  frame False {
                  }
                  frame True {
                    n1605 = local read "Room Temp"() -> (w3013:dbl)
                  }
                }
                n1606 = local read "NumPoints Log"() -> (w2950:dbl)
                n1607 = local write "Transfer File"(w2907) -> ()
                n1608 = local read "Num Pts"() -> (w2939:dbl)
                n1609 = local read "Num Pts"() -> (w2951:dbl)
                n1610 = call-poly <vilib>:"Read From Spreadsheet File.vi"("file path (dialog if empty)"=w2907) -> ("all rows"=w2998:string[][])  [unwired: 6 in, 4 out]
                n1611 = call "Mobility-Vt Calculator-File.vi"("NumPts"=w2951, "Path"=w2907) -> ("Graph Cluster"=w2898:T9, "Output"=w2952:T10, "Index-Sat"=w2932:dbl, "Index-Lin"=w2938:dbl)  [unwired: 5 in, 1 out]
                n1612 = Unbundle By Name(w2898) -> ("Raw Sat"=w2895:cluster{dbl[], dbl[]}[], "Sqrt Sat"=w2897:cluster{dbl[], dbl[]}[], "Log Sat"=w2894:cluster{dbl[], dbl[]}[], "Raw Lin"=w2893:cluster{dbl[], dbl[]}[], "Sqrt Lin"=w2896:cluster{dbl[], dbl[]}[], "Log Lin"=w2892:cluster{dbl[], dbl[]}[])
                n1613 = Decimate 1D Array(w2896) -> (w2946:cluster{dbl[], dbl[]}[])  [unwired: 1 out]
                n1614 = Array To Cluster(array=w2946) -> (cluster=w2944:T11)
                n1615 = Unbundle(w2944) -> ("[0]"=w2945:cluster{dbl[], dbl[]})  [unwired: 8 out]
                n1616 = Unbundle(w2945) -> (w2943:dbl[], w2942:dbl[])
                n1617 = Array Subset(array=w2942, index=w2938, length=w2939) -> (w2940:dbl[])
                n1618 = Array Subset(array=w2943, index=w2938, length=w2939) -> (w2941:dbl[])
                n1619 = call "STS Calculator-File.vi"("NumPts"=w2950, "Path"=w2907) -> ("STS Index-Sat"=w2949:dbl, "XY Graph-Sat"=w2948:cluster{dbl[], dbl[]}[], "Ouput"=w2947:cluster{"STS-Sat":dbl, "STS-Lin":dbl})  [unwired: 5 in, 2 out]
                n1620 = local read "New: Dielectric"() -> (w2934:dbl)
                n1621 = local write "Sat-Trans Slider"(w2932) -> ()
                n1622 = local write "Lin Id-Used"(w2940) -> ()
                n1623 = local write "Lin-Vg Array-Used"(w2941) -> ()
                n1624 = local write "MobVi Index"(w2932) -> ()
                n1625 = local write "Index 2"(w2949) -> ()
                n1626 = local write "Sqrt-Sat"(w2897) -> ()
                n1627 = local write "Log-Sat"(w2948) -> ()
                n1628 = Unbundle By Name(w2952) -> ("Mobility-Sat"=w2937:dbl, "Vt-Sat"=w2899:dbl, "Mobility-Lin"=w2936:dbl, "Mobility-Lin"=w2935:dbl, "Off I-Sat"=w2930:dbl, "On/Off I-Sat"=w2900:dbl)
                n1629 = local write "Sqrt-Lin"(w2896) -> ()
                n1630 = Array Size(array=w2998) -> (size(s)=w2997:i32[])
                n1631 = local write "Raw- Sat"(w2895) -> ()
                n1632 = local write "New: Temp"(w2902) -> ()
                n1633 = Unbundle By Name(w2947) -> ("STS-Sat"=w2933:dbl)
                n1634 = call "Trap Density_STS.vi"("Temp (T) [K]"=w2902, "S.T.S. (S)"=w2933, "Dielectric"=w2934) -> ("Trap Density (N)"=w2906:dbl)  [unwired: 8 in]
                n1635 = local write "Calc: Mobility-Lin"(w2936) -> ()
                n1636 = local write "Raw- Lin"(w2893) -> ()
                n1637 = local write "Log-Sat"(w2894) -> ()
                n1638 = local write "Calc: Mobility-Sat"(w2937) -> ()
                n1639 = local write "Log-Lin"(w2892) -> ()
                n1640 = local write "Calc: Off I-Sat"(w2930) -> ()
                n1641 = local write "Calc: VT-Sat"(w2899) -> ()
                n1642 = local write "New: VT-Lin"(w2935) -> ()
                n1643 = local write "New: Trap Density-STS"(w2906) -> ()
                n1644 = local write "Calc: Trap Density-STS"(w2906) -> ()
                n1645 = local read "Image Folder"() -> (w2986:path)
                n1646 = local read "New: Dielectric"() -> (w2931:dbl)
                n1647 = Decimate 1D Array(w2897) -> (w2981:cluster{dbl[], dbl[]}[])  [unwired: 1 out]
                n1648 = Decimate 1D Array(w2948) -> (w2971:cluster{dbl[], dbl[]}[])  [unwired: 1 out]
                n1649 = Index Array(array=w2997, index=w2996) -> (element=w2977:i32)
                n1650 = Array Subset(array=w2998, index (row)=w2996, index (col)=w2996, length (col)=3) -> (w2999:string[][])  [unwired: 1 in]
                n1651 = local write "Calc: STS"(w2933) -> ()
                n1652 = local write "New: VT-Sat"(w2899) -> ()
                n1653 = local write "New: Mobility-Sat"(w2937) -> ()
                n1654 = local write "Calc: On/Off"(w2900) -> ()
                n1655 = local write "New: Mobility-Lin"(w2936) -> ()
                n1656 = List Folder(path=w2986) -> (filenames=w2991:string[])  [unwired: 3 in, 3 out]
                n1657 = local write "New: VT-Lin"(w2935) -> ()
                n1658 = Array To Cluster(array=w2981) -> (cluster=w2983:T11)
                n1659 = Array To Cluster(array=w2971) -> (cluster=w2969:T11)
                n1660 = Reshape Array(w2999, w2977) -> (w2984:string[])
                n1661 = Subtract(x=w2977, y=20) -> (x-y=w2976:i32)
                n1662 = local write "New: STS"(w2933) -> ()
                n1663 = property on="Sat-Trans Slider" class="Slide (strict)"("Scale.Maximum"=w2976) -> ()  [unwired: 2 in, 2 out]
                n1664 = call "Trap Density_VT.vi"("VT"=w2899, "Dielectric"=w2931) -> ("Trap Density-VT"=w2903:dbl)
                n1665 = Unbundle(w2983) -> ("[0]"=w2982:cluster{dbl[], dbl[]})  [unwired: 8 out]
                n1666 = Unbundle(w2969) -> ("[0]"=w2970:cluster{dbl[], dbl[]})  [unwired: 8 out]
                n1667 = Search 1D Array(1D array=w2984, element="Index:") -> (index of element=w2993:i32)  [unwired: 1 in]
                n1668 = local write "New: Trap Density-VT"(w2903) -> ()
                n1669 = local write "Calc: Trap Density-VT"(w2903) -> ()
                n1670 = Unbundle(w2982) -> (w2973:dbl[], w2972:dbl[])
                n1671 = Unbundle(w2970) -> (w2968:dbl[], w2967:dbl[])
                n1672 = Increment(x=w2993) -> (x+1=w2994:i32)
                n1673 = Array Subset(array=w2973, index=w2932, length=w2951) -> (w2980:dbl[])
                n1674 = Array Subset(array=w2972, index=w2932, length=w2951) -> (w2979:dbl[])
                n1675 = Array Subset(array=w2968, index=w2949, length=w2950) -> (w2975:dbl[])
                n1676 = Array Subset(array=w2967, index=w2949, length=w2950) -> (w2974:dbl[])
                n1677 = Index Array(array=w2984, index=w2994) -> (element=w2989:string)
                n1678 = local write "Vg Array-Log-Used"(w2974) -> ()
                n1679 = local write "Sat Id-Log-Used"(w2975) -> ()
                n1680 = local write "Sat Id-Used"(w2979) -> ()
                n1681 = local write "Index"(w2989) -> ()
                n1682 = local write "Sat Vg Array-Used"(w2980) -> ()
                n1683 = while {
                  tunnel: w2991 -> [w3021]
                  tunnel: w2989 -> [w3019]
                  tunnel: [w3018] -> _
                  tunnel: [w3018] -> w2990
                  tunnel: w2977 -> [w3017]
                  i -> [w3018]
                  stop <- w3014 stop-if-true
                  n1684 = Index Array(array=w3021, index=w3018) -> (element=w3022:string)
                  n1685 = xnode "Match Regular Expression"("input string"=w3022, "regular expression"=w3019) -> ("whole match"=w3020:string)  [unwired: 4 in, 4 out]
                  n1686 = Equal?(x=w3020, y=w3019) -> (x = y?=w3016:bool)
                  n1687 = Equal?(x=w3017, y=w3018) -> (x = y?=w3015:bool)
                  n1688 = Or(x=w3016, y=w3015) -> (x .or. y?=w3014:bool)
                }
                n1689 = Path To String(path=w2986) -> (string=w2988:string)
                n1690 = Index Array(array=w2991, index=w2990) -> (element=w2965:string)
                n1691 = local write "Image Name"(w2965) -> ()
                n1692 = Empty String/Path?(string/path=w2965) -> (empty?=w2966:bool)
                n1693 = Concatenate Strings(w2988, "\\", w2965) -> (w2987:string)
                n1694 = String To Path(string=w2987) -> (path=w2964:path)
                n1695 = local read "No Image File"() -> (w2963:path)
                n1696 = Select(t=w2963, s=w2966, f=w2964) -> (s? t:f=w2957:path)
                n1697 = local write "Image File"(w2957) -> ()
                n1698 = local read "Image Out"() -> (w2955:T2)
                n1699 = call "IMAQ ReadFile"("File Path"=w2957, "Image"=w2955) -> ("Image Out"=w2956:T2)  [unwired: 5 in, 4 out]
                n1700 = local write "Image Out"(w2956) -> ()
                n1701 = local write "Image Out 2"(w2956) -> ()
              }
              frame #4 {
                # "Output ROI data"
                n1702 = local read "Image Folder"() -> (w3137:path)
                n1703 = Build Path(base path=w3137, name or relative path="ROI") -> (appended path=w3139:path)
                n1704 = local read "Index"() -> (w3138:string)
                n1705 = Build Path(base path=w3139, name or relative path=w3138) -> (appended path=w3144:path)
                n1706 = invoke on="Image Out" class="ImageControl" method="Clear ROI"() -> (error out=w3143:errorcluster)  [unwired: 3 in, 2 out]
                n1707 = call <vilib>:"Check if File or Folder Exists.vi"("error in (no error)"=w3143, "path"=w3144) -> ("file or folder exists?"=w3141:bool, "dup path"=w3142:path)  [unwired: 7 in, 1 out]
                n1708 = case shown="True" w3141 {
                  tunnel: w3142 -> [_ w3145]
                  frame False {
                  }
                  frame True {
                    n1709 = Read from Text File(file (use dialog)=w3145) -> (text=w3149:string)  [unwired: 3 in, 3 out]
                    n1710 = property on="Image Out" class="ImageControl"() -> ("ROI"=w3146:T12)  [unwired: 2 in, 2 out]
                    n1711 = Unflatten From String(type=w3146, binary string=w3149) -> (value=w3147:T12, error out=w3148:errorcluster)  [unwired: 3 in, 1 out]
                    n1712 = property on="Image Out" class="ImageControl"(error in=w3148, "ROI"=w3147) -> ()  [unwired: 1 in, 2 out]
                  }
                }
              }
            }
            n1713 = flat-sequence {
              tunnel: [w2358] -> w2345
              tunnel: w2345 -> [w2372]
              frame #0 {
                # "Makes Empty File for Transformer Data"
                n1714 = local read "Transfer Folder"() -> (w2347:path)
                n1715 = Build Path(base path=w2347, name or relative path="Stats") -> (appended path=w2349:path)
                n1716 = call <vilib>:"Check if File or Folder Exists.vi"("path"=w2349) -> ("file or folder exists?"=w2350:bool, "dup path"=w2351:path)  [unwired: 8 in, 1 out]
                n1717 = case shown="False" w2350 {
                  tunnel: [w2355 w2357] -> w2352
                  tunnel: w2351 -> [w2356 w2357]
                  frame False {
                    n1718 = Create Folder(path (use dialog)=w2356) -> (created path=w2355:path)  [unwired: 2 in, 2 out]
                  }
                  frame True {
                  }
                }
                n1719 = Build Path(base path=w2352, name or relative path="Tranformer Data.txt") -> (appended path=w2354:path)
                n1720 = call-poly <vilib>:"Write To Spreadsheet File.vi"("append to file? (new file:F)"=TRUE, "file path (dialog if empty)"=w2354) -> ()  [unwired: 6 in, 1 out]
              }
              frame #1 {
                # "Adds Headers if they don't exist"
                n1721 = local read "Transfer Folder"() -> (w2364:path)
                n1722 = Concatenate Strings("Stats\\", "Tranformer Data.txt") -> (w2365:string)
                n1723 = Build Path(base path=w2364, name or relative path=w2365) -> (appended path=w2358:path)
                n1724 = call-poly <vilib>:"Read From Spreadsheet File.vi"("file path (dialog if empty)"=w2358) -> ("first row"=w2363:string[])  [unwired: 6 in, 4 out]
                n1725 = Search 1D Array(1D array=w2363, element="DeviceID") -> (index of element=w2361:i32)  [unwired: 1 in]
                n1726 = Equal?(x=w2361, y=0) -> (x = y?=w2359:bool)
                n1727 = case shown="False" w2359 {
                  tunnel: w2358 -> [w2369 _]
                  frame False {
                    n1728 = local read "Transformer \nHeaders"() -> (w2368:string[])
                    n1729 = call-poly <vilib>:"Write To Spreadsheet File.vi"("1D data"=w2368, "file path (dialog if empty)"=w2369) -> ()  [unwired: 6 in, 1 out]
                  }
                  frame True {
                  }
                }
              }
              frame #2 {
                # "Adds current device if it doesn't exist"
                n1730 = local read "Current \nRecord"() -> (w2375:string[])
                n1731 = Index Array(array=w2375, index=0) -> (element=w2374:string)
                n1732 = local read "Transfer Folder"() -> (w2377:path)
                n1733 = Concatenate Strings("Stats\\", "Tranformer Data.txt") -> (w2378:string)
                n1734 = local write "Current Device ID"(w2374) -> ()
                n1735 = local read "Current Device ID"() -> (w2384:string)
                n1736 = Build Path(base path=w2377, name or relative path=w2378) -> (appended path=w2376:path)
                n1737 = call-poly <vilib>:"Read From Spreadsheet File.vi"("file path (dialog if empty)"=w2376) -> ("all rows"=w2371:string[][])  [unwired: 6 in, 4 out]
                n1738 = Index Array(array=w2371, index (col)=0) -> (element=w2382:string[])  [unwired: 1 in]
                n1739 = Search 1D Array(1D array=w2382, element=w2384) -> (index of element=w2370:i32)  [unwired: 1 in]
                n1740 = Equal?(x=w2370, y=-1) -> (x = y?=w2373:bool)
                n1741 = case shown="False" w2373 {
                  tunnel: w2372 -> [w2386 w2399]
                  tunnel: w2370 -> [w2391 _]
                  tunnel: w2371 -> [w2392 _]
                  frame False {
                    n1742 = local read "Current \nRecord"() -> (w2390:string[])
                    n1743 = Replace Array Subset(array=w2392, new element=w2390, index (row)=w2391) -> (w2387:string[][])  [unwired: 1 in]
                    n1744 = flat-sequence {
                      tunnel: [w2393] -> _
                      tunnel: [w2394] -> _
                      tunnel: [w2394] -> w2389
                      tunnel: [w2393] -> w2388
                      tunnel: w2387 -> [w2394]
                      tunnel: w2386 -> [w2393]
                      tunnel: w2389 -> [w2396]
                      tunnel: w2388 -> [w2395]
                      frame #0 {
                        n1745 = Delete(path (use dialog)=w2393) -> ()  [unwired: 4 in, 3 out]
                      }
                      frame #1 {
                        n1746 = call-poly <vilib>:"Write To Spreadsheet File.vi"("append to file? (new file:F)"=TRUE, "2D data"=w2396, "file path (dialog if empty)"=w2395) -> ()  [unwired: 5 in, 1 out]
                      }
                    }
                  }
                  frame True {
                    n1747 = local read "Current \nRecord"() -> (w2398:string[])
                    n1748 = call-poly <vilib>:"Write To Spreadsheet File.vi"("append to file? (new file:F)"=TRUE, "1D data"=w2398, "file path (dialog if empty)"=w2399) -> ()  [unwired: 5 in, 1 out]
                  }
                }
              }
            }
          }
          event "Export": Mouse Down {
            n1749 = event-data() -> ()  [unwired: 1 in, 7 out]
            n1750 = flat-sequence {
              frame #0 {
                n1751 = stacked-sequence {
                  frame #0 {
                    n1752 = local read "Independant Variable"() -> (w3151:string)
                    n1753 = Equal?(x=w3151, y="Length (um):") -> (x = y?=w3152:bool)
                    n1754 = case shown="True" w3152 {
                      frame False {
                      }
                      frame True {
                        n1755 = local write "X Axis Display Type"("1") -> ()
                        n1756 = local write "Opj X Axis"("2") -> ()
                      }
                    }
                  }
                  frame #1 {
                    n1757 = local read "Independant Variable"() -> (w3156:string)
                    n1758 = Equal?(x=w3156, y="Sample Temp (K):") -> (x = y?=w3157:bool)
                    n1759 = case shown="True" w3157 {
                      frame False {
                      }
                      frame True {
                        n1760 = local write "X Axis Display Type"("1") -> ()
                        n1761 = local write "Opj X Axis"("1") -> ()
                      }
                    }
                  }
                  frame #2 {
                    n1762 = local read "Independant Variable"() -> (w3161:string)
                    n1763 = Equal?(x=w3161, y="Mobility-Sat (cm^2/Vs):") -> (x = y?=w3162:bool)
                    n1764 = case shown="True" w3162 {
                      frame False {
                      }
                      frame True {
                        n1765 = local write "X Axis Display Type"("2") -> ()
                        n1766 = local write "Opj X Axis"("2") -> ()
                      }
                    }
                  }
                  frame #3 {
                    n1767 = local read "Independant Variable"() -> (w3166:string)
                    n1768 = Equal?(x=w3166, y="Mobility-Lin (cm^2/Vs):") -> (x = y?=w3167:bool)
                    n1769 = case shown="True" w3167 {
                      frame False {
                      }
                      frame True {
                        n1770 = local write "X Axis Display Type"("2") -> ()
                        n1771 = local write "Opj X Axis"("2") -> ()
                      }
                    }
                  }
                  frame #4 {
                    n1772 = local read "Independant Variable"() -> (w3171:string)
                    n1773 = Equal?(x=w3171, y="On/Off I-Sat:") -> (x = y?=w3172:bool)
                    n1774 = case shown="True" w3172 {
                      frame False {
                      }
                      frame True {
                        n1775 = local write "X Axis Display Type"("2") -> ()
                        n1776 = local write "Opj X Axis"("2") -> ()
                      }
                    }
                  }
                  frame #5 {
                    n1777 = local read "Independant Variable"() -> (w3176:string)
                    n1778 = Equal?(x=w3176, y="Off I-Sat (A):") -> (x = y?=w3177:bool)
                    n1779 = case shown="True" w3177 {
                      frame False {
                      }
                      frame True {
                        n1780 = local write "X Axis Display Type"("2") -> ()
                        n1781 = local write "Opj X Axis"("2") -> ()
                      }
                    }
                  }
                  frame #6 {
                    n1782 = local read "Independant Variable"() -> (w3181:string)
                    n1783 = Equal?(x=w3181, y="Vt-Sat (V):") -> (x = y?=w3182:bool)
                    n1784 = case shown="True" w3182 {
                      frame False {
                      }
                      frame True {
                        n1785 = local write "X Axis Display Type"("1") -> ()
                        n1786 = local write "Opj X Axis"("1") -> ()
                      }
                    }
                  }
                  frame #7 {
                    n1787 = local read "Independant Variable"() -> (w3186:string)
                    n1788 = Equal?(x=w3186, y="STS-Sat (V/decade):") -> (x = y?=w3187:bool)
                    n1789 = case shown="True" w3187 {
                      frame False {
                      }
                      frame True {
                        n1790 = local write "X Axis Display Type"("1") -> ()
                        n1791 = local write "Opj X Axis"("1") -> ()
                      }
                    }
                  }
                  frame #8 {
                    n1792 = local read "Independant Variable"() -> (w3191:string)
                    n1793 = Equal?(x=w3191, y="Trap Density-VT (Traps/Vcm^2):") -> (x = y?=w3192:bool)
                    n1794 = case shown="True" w3192 {
                      frame False {
                      }
                      frame True {
                        n1795 = local write "X Axis Display Type"("2") -> ()
                        n1796 = local write "Opj X Axis"("2") -> ()
                      }
                    }
                  }
                  frame #9 {
                    n1797 = local read "Independant Variable"() -> (w3196:string)
                    n1798 = Equal?(x=w3196, y="Trap Density-STS (Traps/Vcm^2):") -> (x = y?=w3197:bool)
                    n1799 = case shown="True" w3197 {
                      frame False {
                      }
                      frame True {
                        n1800 = local write "X Axis Display Type"("2") -> ()
                        n1801 = local write "Opj X Axis"("2") -> ()
                      }
                    }
                  }
                }
              }
              frame #1 {
                n1802 = local read "Transfer Folder"() -> (w3205:path)
                n1803 = Build Path(base path=w3205, name or relative path="Stats") -> (appended path=w3206:path)
                n1804 = local read "Origin Project File"() -> (w3217:path)
                n1805 = call <vilib>:"Check if File or Folder Exists.vi"("path"=w3206) -> ("file or folder exists?"=w3221:bool, "dup path"=w3220:path)  [unwired: 8 in, 1 out]
                n1806 = call <userlib>:"OA_ConnectToOrigin.vi"() -> ("error out"=w3218:errorcluster, "Origin.IOApplication"=w3219:refnum<k7>)  [unwired: 8 in]
                n1807 = case shown="False" w3221 {
                  tunnel: w3220 -> [w3394 w3395]
                  tunnel: [w3393 w3395] -> w3204
                  frame False {
                    n1808 = Create Folder(path (use dialog)=w3394) -> (created path=w3393:path)  [unwired: 2 in, 2 out]
                  }
                  frame True {
                  }
                }
                n1809 = call <userlib>:"OA_Load.vi"("error in (no error)"=w3218, "Path"=w3217, "Origin.IOApplication"=w3219) -> ("error out"=w3215:errorcluster, "Origin.IOApplication"=w3216:refnum<k7>)  [unwired: 1 out]
                n1810 = call "OAExecute.vi"("script"="document -m 3;", "Error IO"=w3215, "Origin.IOApplication"=w3216) -> ("Error IO Out"=w3213:errorcluster, "Origin.IOApplication"=w3214:refnum<k7>)  [unwired: 1 in, 1 out]
                n1811 = call "File Dialog"("start path"=w3206) -> ("selected path"=w3208:path)  [unwired: 11 in, 3 out]
                n1812 = local read "Independant Variable"() -> (w3201:string)
                n1813 = stacked-sequence {
                  tunnel: w3205 -> [w3232 w3262 w3274 w3296 w3316 w3337 w3358 w3381]
                  tunnel: w3204 -> [w3233 w3261 w3275 w3295 w3317 w3338 w3359 w3382]
                  tunnel: w3214 -> [w3235 w3259 w3277 w3298 w3319 w3340 w3361 w3384]
                  tunnel: w3213 -> [w3234 w3260 w3276 w3297 w3318 w3339 w3360 w3383]
                  tunnel: [_ _ _ _ _ _ _ w3379] -> w3203
                  tunnel: [_ _ _ _ _ _ _ w3380] -> w3202
                  tunnel: w3201 -> [w3231 w3252 w3273 w3294 w3315 w3336 w3357 w3378]
                  frame #0 {
                    n1814 = local read "X Axis Display Type"() -> (w3223:string)
                    n1815 = local read "Opj X Axis"() -> (w3228:string)
                    n1816 = Concatenate Strings("window -a MOBLGraph;\nlayer.x.type=", w3228, "; layer.x.label.numFormat = ", w3223, "; Y3 = 1; X3 = 1;", "window -a MOBLTable;\nwindow -s TV;") -> (w3226:string)
                    n1817 = call "Param_Analysis_7_24b_JW.vi"("Independant Variable"=w3231, "error in (no error)"=w3234, "Data Folder"=w3232, "Parameter String"="Mobility-Lin (cm^2/Vs):", "Parameter Name"="Mobility-Lin", "Stats Folder"=w3233) -> ("error out"=w3237:errorcluster, "Output Array"=w3239:string[][], "Variables"=w3230:T18)  [unwired: 2 in, 1 out]
                    n1818 = call "Origin_Export_7_27a_JW.vi"("Input Conditions"=w3230, "Analysis Array"=w3239, "error in (no error)"=w3237, "Parameter Worksheet Name"="[MOBLTable]Mobilities", "Parameter Folder Script"="pe_cd \"Mobility-Lin\";", "Origin.IOApplication"=w3235) -> ("error out"=w3236:errorcluster, "reference out"=w3238:refnum<k7>)  [unwired: 3 in, 1 out]
                    n1819 = call "OAExecute.vi"("script"=w3226, "Error IO"=w3236, "Origin.IOApplication"=w3238) -> ()  [unwired: 1 in, 3 out]
                  }
                  frame #1 {
                    n1820 = local read "X Axis Display Type"() -> (w3244:string)
                    n1821 = local read "Opj X Axis"() -> (w3249:string)
                    n1822 = Concatenate Strings("window -a MOBSGraph;\nlayer.x.type=", w3249, "; layer.x.label.numFormat = ", w3244, "; Y3 = 1; X3 = 1;", "window -a MOBSTable;\nwindow -s TV;") -> (w3247:string)
                    n1823 = call "Param_Analysis_7_24b_JW.vi"("Independant Variable"=w3252, "error in (no error)"=w3260, "Data Folder"=w3262, "Parameter String"="Mobility-Sat (cm^2/Vs):", "Parameter Name"="Mobility-Sat", "Stats Folder"=w3261) -> ("error out"=w3255:errorcluster, "Output Array"=w3253:string[][], "Variables"=w3251:T18)  [unwired: 2 in, 1 out]
                    n1824 = call "Origin_Export_7_27a_JW.vi"("Input Conditions"=w3251, "Analysis Array"=w3253, "error in (no error)"=w3255, "Parameter Worksheet Name"="[MOBSTable]Mobilities", "Parameter Folder Script"="pe_cd \"Mobility-Sat\";", "Origin.IOApplication"=w3259) -> ("error out"=w3254:errorcluster, "reference out"=w3256:refnum<k7>)  [unwired: 3 in, 1 out]
                    n1825 = call "OAExecute.vi"("script"=w3247, "Error IO"=w3254, "Origin.IOApplication"=w3256) -> ()  [unwired: 1 in, 3 out]
                  }
                  frame #2 {
                    n1826 = local read "X Axis Display Type"() -> (w3265:string)
                    n1827 = local read "Opj X Axis"() -> (w3270:string)
                    n1828 = Concatenate Strings("window -a NSTSGraph;\nlayer.x.type=", w3270, "; layer.x.label.numFormat = ", w3265, "; Y3 = 1; X3 = 1;", "window -a NSTSTable;\nwindow -s TV;") -> (w3268:string)
                    n1829 = call "Param_Analysis_7_24b_JW.vi"("Independant Variable"=w3273, "error in (no error)"=w3276, "Data Folder"=w3274, "Parameter String"="Trap Density-STS (Traps/Vcm^2):", "Parameter Name"="Trap Density-STS", "Stats Folder"=w3275) -> ("error out"=w3280:errorcluster, "Output Array"=w3278:string[][], "Variables"=w3272:T18)  [unwired: 2 in, 1 out]
                    n1830 = call "Origin_Export_7_27a_JW.vi"("Input Conditions"=w3272, "Analysis Array"=w3278, "error in (no error)"=w3280, "Parameter Worksheet Name"="[NSTSTable]Trap Densities", "Parameter Folder Script"="pe_cd \"N-STS\";", "Origin.IOApplication"=w3277) -> ("error out"=w3279:errorcluster, "reference out"=w3281:refnum<k7>)  [unwired: 3 in, 1 out]
                    n1831 = call "OAExecute.vi"("script"=w3268, "Error IO"=w3279, "Origin.IOApplication"=w3281) -> ()  [unwired: 1 in, 3 out]
                  }
                  frame #3 {
                    n1832 = local read "X Axis Display Type"() -> (w3286:string)
                    n1833 = local read "Opj X Axis"() -> (w3291:string)
                    n1834 = call "Param_Analysis_7_24b_JW.vi"("Independant Variable"=w3294, "error in (no error)"=w3297, "Data Folder"=w3296, "Parameter String"="Trap Density-VT (Traps/Vcm^2):", "Parameter Name"="Trap Density-Vt", "Stats Folder"=w3295) -> ("error out"=w3301:errorcluster, "Output Array"=w3299:string[][], "Variables"=w3293:T18)  [unwired: 2 in, 1 out]
                    n1835 = Concatenate Strings("window -a NVtGraph;\nlayer.x.type=", w3291, "; layer.x.label.numFormat = ", w3286, "; Y3 = 1; X3 = 1;", "window -a NVtTable;\nwindow -s TV;") -> (w3289:string)
                    n1836 = call "Origin_Export_7_27a_JW.vi"("Input Conditions"=w3293, "Analysis Array"=w3299, "error in (no error)"=w3301, "Parameter Worksheet Name"="[NVTTable]Trap Densities", "Parameter Folder Script"="pe_cd \"N-Vt\";", "Origin.IOApplication"=w3298) -> ("error out"=w3300:errorcluster, "reference out"=w3302:refnum<k7>)  [unwired: 3 in, 1 out]
                    n1837 = call "OAExecute.vi"("script"=w3289, "Error IO"=w3300, "Origin.IOApplication"=w3302) -> ()  [unwired: 1 in, 3 out]
                  }
                  frame #4 {
                    n1838 = local read "X Axis Display Type"() -> (w3307:string)
                    n1839 = local read "Opj X Axis"() -> (w3312:string)
                    n1840 = Concatenate Strings("window -a OffIGraph;\nlayer.x.type=", w3312, "; layer.x.label.numFormat = ", w3307, "; Y3 = 1; X3 = 1;", "window -a OffITable;\nwindow -s TV;") -> (w3310:string)
                    n1841 = call "Param_Analysis_7_24b_JW.vi"("Independant Variable"=w3315, "error in (no error)"=w3318, "Data Folder"=w3316, "Parameter String"="Off I-Sat (A):", "Parameter Name"="Off I-Sat", "Stats Folder"=w3317) -> ("error out"=w3322:errorcluster, "Output Array"=w3320:string[][], "Variables"=w3314:T18)  [unwired: 2 in, 1 out]
                    n1842 = call "Origin_Export_7_27a_JW.vi"("Input Conditions"=w3314, "Analysis Array"=w3320, "error in (no error)"=w3322, "Parameter Worksheet Name"="[OffItable]OffCurrents", "Parameter Folder Script"="pe_cd \"OffI-Sat\";", "Origin.IOApplication"=w3319) -> ("error out"=w3321:errorcluster, "reference out"=w3323:refnum<k7>)  [unwired: 3 in, 1 out]
                    n1843 = call "OAExecute.vi"("script"=w3310, "Error IO"=w3321, "Origin.IOApplication"=w3323) -> ()  [unwired: 1 in, 3 out]
                  }
                  frame #5 {
                    n1844 = local read "X Axis Display Type"() -> (w3328:string)
                    n1845 = local read "Opj X Axis"() -> (w3333:string)
                    n1846 = Concatenate Strings("window -a OnOffGraph;\nlayer.x.type=", w3333, "; layer.x.label.numFormat = ", w3328, "; Y3 = 1; X3 = 1;", "window -a OnOffTable;\nwindow -s TV;") -> (w3331:string)
                    n1847 = call "Param_Analysis_7_24b_JW.vi"("Independant Variable"=w3336, "error in (no error)"=w3339, "Data Folder"=w3337, "Parameter String"="On/Off I-Sat:", "Parameter Name"="OnOff Ratio", "Stats Folder"=w3338) -> ("error out"=w3343:errorcluster, "Output Array"=w3341:string[][], "Variables"=w3335:T18)  [unwired: 2 in, 1 out]
                    n1848 = call "Origin_Export_7_27a_JW.vi"("Input Conditions"=w3335, "Analysis Array"=w3341, "error in (no error)"=w3343, "Parameter Worksheet Name"="[OnOffTable]On/Off Ratios", "Parameter Folder Script"="pe_cd \"OnOff-Ratio\";", "Origin.IOApplication"=w3340) -> ("error out"=w3342:errorcluster, "reference out"=w3344:refnum<k7>)  [unwired: 3 in, 1 out]
                    n1849 = call "OAExecute.vi"("script"=w3331, "Error IO"=w3342, "Origin.IOApplication"=w3344) -> ()  [unwired: 1 in, 3 out]
                  }
                  frame #6 {
                    n1850 = local read "X Axis Display Type"() -> (w3349:string)
                    n1851 = local read "Opj X Axis"() -> (w3354:string)
                    n1852 = call "Param_Analysis_7_24b_JW.vi"("Independant Variable"=w3357, "error in (no error)"=w3360, "Data Folder"=w3358, "Parameter String"="STS-Sat (V/decade):", "Parameter Name"="STS-Sat", "Stats Folder"=w3359) -> ("error out"=w3364:errorcluster, "Output Array"=w3362:string[][], "Variables"=w3356:T18)  [unwired: 2 in, 1 out]
                    n1853 = Concatenate Strings("window -a SGraph;\nlayer.x.type=", w3354, "; layer.x.label.numFormat = ", w3349, "; Y3 = 1; X3 = 1;", "window -a STable;\nwindow -s TV;") -> (w3352:string)
                    n1854 = call "Origin_Export_7_27a_JW.vi"("Input Conditions"=w3356, "Analysis Array"=w3362, "error in (no error)"=w3364, "Parameter Worksheet Name"="[STable]Threshold Swing", "Parameter Folder Script"="pe_cd \"STS-Sat\";", "Origin.IOApplication"=w3361) -> ("error out"=w3363:errorcluster, "reference out"=w3365:refnum<k7>)  [unwired: 3 in, 1 out]
                    n1855 = call "OAExecute.vi"("script"=w3352, "Error IO"=w3363, "Origin.IOApplication"=w3365) -> ()  [unwired: 1 in, 3 out]
                  }
                  frame #7 {
                    n1856 = local read "X Axis Display Type"() -> (w3370:string)
                    n1857 = local read "Opj X Axis"() -> (w3375:string)
                    n1858 = Concatenate Strings("window -a VtGraph;\nlayer.x.type=", w3375, "; layer.x.label.numFormat = ", w3370, "; Y3 = 1; X3 = 1;", "window -a VtTable;\nwindow -s TV;") -> (w3373:string)
                    n1859 = call "Param_Analysis_7_24b_JW.vi"("Independant Variable"=w3378, "error in (no error)"=w3383, "Data Folder"=w3381, "Parameter String"="Vt-Sat (V):", "Parameter Name"="Vt-Sat", "Stats Folder"=w3382) -> ("error out"=w3387:errorcluster, "Output Array"=w3385:string[][], "Variables"=w3377:T18)  [unwired: 2 in, 1 out]
                    n1860 = call "Origin_Export_7_27a_JW.vi"("Input Conditions"=w3377, "Analysis Array"=w3385, "error in (no error)"=w3387, "Parameter Worksheet Name"="[VtTable]Threshold Voltages", "Parameter Folder Script"="pe_cd \"Vt-Sat\";", "Origin.IOApplication"=w3384) -> ("error out"=w3386:errorcluster, "reference out"=w3388:refnum<k7>)  [unwired: 3 in, 1 out]
                    n1861 = call "OAExecute.vi"("script"=w3373, "Error IO"=w3386, "Origin.IOApplication"=w3388) -> ("Error IO Out"=w3379:errorcluster, "Origin.IOApplication"=w3380:refnum<k7>)  [unwired: 1 in, 1 out]
                  }
                }
                n1862 = Path To String(path=w3208) -> (string=w3207:string)
                n1863 = call "OAExecute.vi"("script"="pe_cd /; ", "Error IO"=w3203, "Origin.IOApplication"=w3202) -> ("Error IO Out"=w3209:errorcluster, "Origin.IOApplication"=w3210:refnum<k7>)  [unwired: 1 in, 1 out]
                n1864 = call <userlib>:"OASaveProject.vi"("path"=w3207, "Error IO"=w3209, "Origin.IOApplication"=w3210) -> ()  [unwired: 3 out]
              }
            }
          }
          event "Blank Button": Mouse Down {
            n1865 = event-data() -> ()  [unwired: 1 in, 7 out]
            n1866 = local read "Transfer File"() -> (w3403:path)
            n1867 = disable-structure shown="Disabled" {
              frame Disabled {
                n1868 = local read "Folder Index"() -> (w3404:dbl)
                n1869 = Decrement(x=w3404) -> (x-1=w3405:dbl)
                n1870 = local write "Folder Index"(w3405) -> ()
              }
              frame Enabled {
              }
            }
            n1871 = Strip Path(path=w3403) -> (stripped path=w3399:path, name=w3401:string)
            n1872 = Path To String(path=w3399) -> (string=w3398:string)
            n1873 = Concatenate Strings(w3398, "\\", "X_", w3401) -> (w3397:string)
            n1874 = String To Path(string=w3397) -> (path=w3396:path)
            n1875 = Move(source path=w3403, 10:w3396) -> ()  [unwired: 3 in, 3 out]
            n1876 = local write "Transfer File"(w3396) -> ()
          }
          event "Cancel Button": Mouse Down {
            (unwired) 6
            n1877 = event-data() -> ()  [unwired: 1 in, 7 out]
            n1878 = call "Simulate_Keyboard.vi"("Action"=2, "Virtual Key"=162) -> ()  [unwired: 7 in, 1 out]
          }
        }
        n1879 = Multiply(x=w555, y=10) -> (x*y=w557:sgl)
        n1880 = case shown="\"0\"" w596 {
          tunnel: w570 -> [w667 w673 w677 w679 w683 w685 w687 w689 w691 w693 w695 w697 w699 w701 w703 w705 w707 w709 w711 w713 w715 w717 w719 w721 w723 w725 w727 w729 w731 w733 w735 w737 w739 w741 w743 w745 w747 w749 w751 w753 w755 w757 w759 w761 w763 w765 w767 w769 w771 w773 w775 w777 w779 w781 w783 w785 w787 w789 w791 w793 w795 w797 w799 w801 w803 w805 w807 w809 w811 w813 w815 w817 w819 w821 w823 w825 w827 w829 w831 w833 w835 w837 w839 w841 w843 w845 w847 w849 w851 w853 w855 w857 w859 w861 w863 w865 w867 w869 w871 w873 w875 w877 w879 w881 w883]
          tunnel: [w667 w672 w676 w679 w683 w685 w687 w689 w691 w693 w695 w697 w699 w701 w703 w705 w707 w709 w711 w713 w715 w717 w719 w721 w723 w725 w727 w729 w731 w733 w735 w737 w739 w741 w743 w745 w747 w749 w751 w753 w755 w757 w759 w761 w763 w765 w767 w769 w771 w773 w775 w777 w779 w781 w783 w785 w787 w789 w791 w793 w795 w797 w799 w801 w803 w805 w807 w809 w811 w813 w815 w817 w819 w821 w823 w825 w827 w829 w831 w833 w835 w837 w839 w841 w843 w845 w847 w849 w851 w853 w855 w857 w859 w861 w863 w865 w867 w869 w871 w873 w875 w877 w879 w881 w883] -> w595
          tunnel: w571 -> [w669 w671 w675 w681 w682 w684 w686 w688 w690 w692 w694 w696 w698 w700 w702 w704 w706 w708 w710 w712 w714 w716 w718 w720 w722 w724 w726 w728 w730 w732 w734 w736 w738 w740 w742 w744 w746 w748 w750 w752 w754 w756 w758 w760 w762 w764 w766 w768 w770 w772 w774 w776 w778 w780 w782 w784 w786 w788 w790 w792 w794 w796 w798 w800 w802 w804 w806 w808 w810 w812 w814 w816 w818 w820 w822 w824 w826 w828 w830 w832 w834 w836 w838 w840 w842 w844 w846 w848 w850 w852 w854 w856 w858 w860 w862 w864 w866 w868 w870 w872 w874 w876 w878 w880 w882]
          tunnel: [w668 w671 w675 w680 w682 w684 w686 w688 w690 w692 w694 w696 w698 w700 w702 w704 w706 w708 w710 w712 w714 w716 w718 w720 w722 w724 w726 w728 w730 w732 w734 w736 w738 w740 w742 w744 w746 w748 w750 w752 w754 w756 w758 w760 w762 w764 w766 w768 w770 w772 w774 w776 w778 w780 w782 w784 w786 w788 w790 w792 w794 w796 w798 w800 w802 w804 w806 w808 w810 w812 w814 w816 w818 w820 w822 w824 w826 w828 w830 w832 w834 w836 w838 w840 w842 w844 w846 w848 w850 w852 w854 w856 w858 w860 w862 w864 w866 w868 w870 w872 w874 w876 w878 w880 w882] -> w594
          tunnel: w557 -> [w666 w670 w674 w678 _ _ _ _ _ _ _ _ _ _ _ _ _ _ _ _ _ _ _ _ _ _ _ _ _ _ _ _ _ _ _ _ _ _ _ _ _ _ _ _ _ _ _ _ _ _ _ _ _ _ _ _ _ _ _ _ _ _ _ _ _ _ _ _ _ _ _ _ _ _ _ _ _ _ _ _ _ _ _ _ _ _ _ _ _ _ _ _ _ _ _ _ _ _ _ _ _ _ _ _ _]
          frame "DOWN" {
            n1881 = Add(x=w669, y=w666) -> (x+y=w668:sgl)
          }
          frame "LEFT" {
            n1882 = Subtract(x=w673, y=w670) -> (x-y=w672:sgl)
          }
          frame "RIGHT" {
            n1883 = Add(x=w677, y=w674) -> (x+y=w676:sgl)
          }
          frame "UP" {
            n1884 = Subtract(x=w681, y=w678) -> (x-y=w680:sgl)
          }
          frame "ENTER (num pad)" {
          }
          frame "' (quote)" {
          }
          frame "END" {
          }
          frame "EQUALS" {
          }
          frame "ESCAPE" {
          }
          frame "GRAVE (`)" {
          }
          frame "HOME" {
          }
          frame "INSERT" {
          }
          frame "LBRACKET" {
          }
          frame "LCONTROL" {
          }
          frame "L ALT" {
          }
          frame "LSHIFT" {
          }
          frame "LWIN" {
          }
          frame "MINUS" {
          }
          frame "MULTIPLY" {
          }
          frame "NEXT" {
          }
          frame "NUMLOCK" {
          }
          frame "NUMPAD_0" {
          }
          frame "NUMPAD_1" {
          }
          frame "NUMPAD_2" {
          }
          frame "NUMPAD_3" {
          }
          frame "NUMPAD_4" {
          }
          frame "NUMPAD_5" {
          }
          frame "NUMPAD_6" {
          }
          frame "NUMPAD_7" {
          }
          frame "NUMPAD_8" {
          }
          frame "NUMPAD_9" {
          }
          frame "PAUSE" {
          }
          frame "PERIOD" {
          }
          frame "PRIOR (PG UP)" {
          }
          frame "RBRACKET" {
          }
          frame "RCONTROL" {
          }
          frame "RETURN" {
          }
          frame "R ALT" {
          }
          frame "RSHIFT" {
          }
          frame "RWIN" {
          }
          frame "SCROLL" {
          }
          frame "SEMICOLON" {
          }
          frame "SLASH" {
          }
          frame "SPACE" {
          }
          frame "SUBTRACT" {
          }
          frame "TAB" {
          }
          frame "DIVIDE" {
          }
          frame "DELETE" {
          }
          frame "DECIMAL" {
          }
          frame "COMMA" {
          }
          frame "CAPITAL" {
          }
          frame "BACKSLASH" {
          }
          frame "BACK" {
          }
          frame "ADD" {
          }
          frame "F15" {
          }
          frame "F14" {
          }
          frame "F13" {
          }
          frame "F12" {
          }
          frame "F11" {
          }
          frame "F10" {
          }
          frame "F9" {
          }
          frame "F8" {
          }
          frame "F7" {
          }
          frame "F6" {
          }
          frame "F5" {
          }
          frame "F4" {
          }
          frame "F3" {
          }
          frame "F2" {
          }
          frame "F1" {
          }
          frame "Z" {
          }
          frame "Y" {
          }
          frame "X" {
          }
          frame "W" {
          }
          frame "V" {
          }
          frame "U" {
          }
          frame "T" {
          }
          frame "S" {
          }
          frame "R" {
          }
          frame "Q" {
          }
          frame "P" {
          }
          frame "O" {
          }
          frame "N" {
          }
          frame "M" {
          }
          frame "L" {
          }
          frame "K" {
          }
          frame "J" {
          }
          frame "I" {
          }
          frame "H" {
          }
          frame "G" {
          }
          frame "F" {
          }
          frame "E" {
          }
          frame "D" {
          }
          frame "C" {
          }
          frame "B" {
          }
          frame "A" {
          }
          frame "9" {
          }
          frame "8" {
          }
          frame "7" {
          }
          frame "6" {
          }
          frame "5" {
          }
          frame "4" {
          }
          frame "3" {
          }
          frame "2" {
          }
          frame "1" {
          }
          frame "0" {
          }
        }
        n1885 = Bundle(w573, w572, w587, w586, 0.0) -> (w585:cluster{dbl, dbl, dbl, dbl, dbl})  [unwired: 1 in]
        n1886 = Bundle("X"=w595, "Y"=w594) -> (w589:cluster{"X":sgl, "Y":sgl})  [unwired: 1 in]
        n1887 = Divide(x=20, y=w556) -> (x/y=w559:sgl)
        n1888 = property on="Image Out" class="ImageControl"("Image Center Position"=w589) -> ()  [unwired: 2 in, 2 out]
        n1889 = call "IMAQ Convert Rectangle to ROI (Polygon)"("Rectangle"=w585) -> ("ROI Descriptor"=w583:T4)  [unwired: 7 in, 2 out]
        n1890 = Bundle("Application Font", w559, w563, w563, w563, w563, w563, TRUE, w561) -> (w565:T19)  [unwired: 1 in]
        n1891 = property on="Image Out 2" class="ImageControl"("ROI"=w583) -> ()  [unwired: 2 in, 2 out]
        n1892 = Bundle(w561, w565, w561, w561) -> (w564:T20)  [unwired: 1 in]
        n1893 = property on="Image Out" class="ImageControl"() -> ("ROI"=w548:T12)  [unwired: 2 in, 2 out]
        n1894 = Unbundle By Name(w548) -> ("Contours"=w612:T16)
        n1895 = local read "Image Out"() -> (w567:T2)
        n1896 = call "IMAQ Clear Overlay"("Image"=w567) -> ("Image Out"=w566:T2)  [unwired: 9 in, 1 out]
        n1897 = Initialize Array(0) -> (w610:i32[])  [unwired: 1 in]
        n1898 = local read "Magnification"() -> (w601:u16)
        n1899 = Array Size(array=w612) -> (size(s)=w611:i32)
        n1900 = Build Array(0.505025, 0.252522, 0.127742, 0.050345, 0.031129) -> (w602:dbl[])
        n1901 = Array Subset(array=w602, index=w601, length=1) -> (w599:dbl[])
        n1902 = property on="Image Out" class="ImageControl"() -> ("ZoomInteger"=w591:cluster{"X":i32, "Y":i32})  [unwired: 2 in, 2 out]
        n1903 = To Double Precision Float(number=w599) -> (double precision float=w598:dbl[])
        n1904 = for {
          N: w611 -> [_]
          shift-right: [w906] -> _
          shift-left: w612 -> [w906]
          shift-right: [w904] -> w597
          shift-left: w610 -> [w903]
          tunnel: w598 -> [w902]
          shift-right: [w899] -> _
          shift-left: w566 -> [w901]
          tunnel: w564 -> [w894]
          i -> [w898]
          n1905 = Index Array(array=w906, index=w898) -> (element=w915:T21)
          n1906 = Unbundle(w915) -> ("Points"=w914:i32[])  [unwired: 2 out]
          n1907 = Array To Cluster(array=w914) -> (cluster=w913:T22)
          n1908 = Unbundle(w913) -> ("Points[0]"=w893:i32, "Points[1]"=w890:i32, "Points[2]"=w905:i32, "Points[3]"=w911:i32)  [unwired: 5 out]
          n1909 = Add(x=w893, y=10) -> (x+y=w891:i32)
          n1910 = Subtract(x=w890, y=w911) -> (x-y=w910:i32)
          n1911 = Subtract(x=w893, y=w905) -> (x-y=w912:i32)
          n1912 = Square(x=w910) -> (x^2=w908:i32)
          n1913 = Square(x=w912) -> (x^2=w909:i32)
          n1914 = Add(x=w909, y=w908) -> (x+y=w907:i32)
          n1915 = Square Root(x=w907) -> (sqrt(x)=w884:dbl)
          n1916 = Multiply(x=w884, y=0.5) -> (x*y=w887:dbl)
          n1917 = Add(x=w887, y=w890) -> (x+y=w889:dbl)
          n1918 = Bundle(w891, w889) -> (w900:cluster{i32, dbl})  [unwired: 1 in]
          n1919 = Multiply(x=w884, y=w902) -> (x*y=w897:dbl[])
          n1920 = Index Array(array=w897) -> (element=w896:dbl)  [unwired: 1 in]
          n1921 = Number To Fractional String(number=w896) -> (F-format string=w895:string)  [unwired: 3 in]
          n1922 = call "IMAQ Overlay Text"("BG Color (Transparent)"=u32 0, "Text Color (black)"=u32 16448250, "Font, Size & Style"=w894, "String"=w895, "Origin"=w900, "Image"=w901) -> ("Image Out"=w899:T2)  [unwired: 4 in, 1 out]
          n1923 = Build Array (concatenate)(w903, w897) -> (w904:dbl[])
          n1924 = local write "Numeric 3"(w884) -> ()
        }
        n1925 = local write "ROI Descriptor"(w548) -> ()
        n1926 = Unbundle(w591) -> ("X"=w590:i32)  [unwired: 1 out]
        n1927 = Add Array Elements(numeric array=w597) -> (sum=w608:dbl)
        n1928 = local write "Distances"(w597) -> ()
        n1929 = local write "Total Width"(w608) -> ()
        n1930 = local write "Zoom"(w590) -> ()
        n1931 = local read "Manual-Width"() -> (w446:bool)
        n1932 = local read "Total Width"() -> (w551:dbl)
        n1933 = local read "Rec: Width"() -> (w549:dbl)
        n1934 = case shown="False" w446 {
          frame False {
            n1935 = property on="New: Width" class="DigNum (strict)"("DisabledEnum"=1) -> ()  [unwired: 2 in, 2 out]
          }
          frame True {
            n1936 = property on="New: Width" class="DigNum (strict)"("DisabledEnum"=0) -> ()  [unwired: 2 in, 2 out]
          }
        }
        n1937 = Not(x=w446) -> (.not. x?=w546:bool)
        n1938 = Equal To 0?(x=w551) -> (x = 0?=w547:bool)
        n1939 = Or(x=w547, y=w446) -> (x .or. y?=w550:bool)
        n1940 = And(x=w547, y=w546) -> (x .and. y?=w545:bool)
        n1941 = case shown="True" w545 {
          tunnel: w549 -> [_ w642]
          frame False {
          }
          frame True {
            n1942 = local write "New: Width"(w642) -> ()
          }
        }
        n1943 = case shown="False" w550 {
          tunnel: w551 -> [w644 _]
          frame False {
            n1944 = local write "New: Width"(w644) -> ()
            n1945 = property on="New: Width" class="DigNum (strict)"("DisabledEnum"=1) -> ()  [unwired: 2 in, 2 out]
          }
          frame True {
            n1946 = property on="New: Width" class="DigNum (strict)"("DisabledEnum"=0) -> ()  [unwired: 2 in, 2 out]
          }
        }
        n1947 = local read "Manual Comments"() -> (w447:bool)
        n1948 = local read "Rec: Comments"() -> (w448:string)
        n1949 = local read "Manuel-Dielectric"() -> (w474:bool)
        n1950 = local read "Rec: Dielectric (d)"() -> (w473:dbl)
        n1951 = local read "Manuel-Length"() -> (w475:bool)
        n1952 = local read "Rec: Length"() -> (w476:dbl)
        n1953 = case shown="True" w447 {
          tunnel: w448 -> [w617 _]
          frame False {
            n1954 = local write "Comments:"(w617) -> ()
            n1955 = property on="Comments:" class="Str"("DisabledEnum"=1) -> ()  [unwired: 2 in, 2 out]
          }
          frame True {
            n1956 = property on="Comments:" class="Str"("DisabledEnum"=0) -> ()  [unwired: 2 in, 2 out]
          }
        }
        n1957 = case shown="True" w475 {
          tunnel: w476 -> [w632 _]
          frame False {
            n1958 = local write "New: Length"(w632) -> ()
            n1959 = property on="New: Length" class="DigNum (strict)"("DisabledEnum"=1) -> ()  [unwired: 2 in, 2 out]
          }
          frame True {
            n1960 = property on="New: Length" class="DigNum (strict)"("DisabledEnum"=0) -> ()  [unwired: 2 in, 2 out]
          }
        }
        n1961 = case shown="True" w474 {
          tunnel: w473 -> [w629 _]
          frame False {
            n1962 = local write "New: Dielectric"(w629) -> ()
            n1963 = property on="New: Dielectric" class="DigNum (strict)"("DisabledEnum"=1) -> ()  [unwired: 2 in, 2 out]
          }
          frame True {
            n1964 = property on="New: Dielectric" class="DigNum (strict)"("DisabledEnum"=0) -> ()  [unwired: 2 in, 2 out]
          }
        }
      }
    }
  }
  n1965 = Build Array("DeviceID", "Fabricator", "Deposition", "Date", "Sample", "Row", "Column", "L (um)", "W (um)", "Material", "Treatment", "TC (mM)", "Solvent", "C (%)", "ST (C)", "Drops", "Wait (s)", "RT (F)", "RH (%)", "Ramp (s)", "RPM", "Accel (RPM/s)", "Time (s)", "Mobility", "On/Off", "Vt", "S.T.S") -> (→"Transformer \nHeaders":string[])
